vi "Decode PTU File Header.vi"(8 "error in (no error)":errorcluster, 11 "Tag Array":T1[](array[typedef]) {"TagType" format="%.0x"}) -> (0 "error out":errorcluster, 1 "Tags with Error":string[](array[string]), 3 "PicoQuant Data File Information":T2)   [LabVIEW 2021, in "PTU Files.lvlib"]
uses:
  PTU Files.lvlib
  PicoQuant Data File Information.ctl
  PicoQuant File Information.ctl
  PicoQuant Software Information.ctl
  PicoQuant Remote Request Information.ctl
  PicoQuant Hardware Information.ctl
  PicoQuant Input Channels.ctl
  PicoQuant Markers.ctl
  PicoQuant Modules.ctl
  PicoQuant Router Channels.ctl
  PicoQuant Measurement Information.ctl
  PicoQuant Image Information.ctl
  PicoQuant Results Format.ctl
  PicoQuant Measurement Results.ctl
  PicoQuant Header Tag.ctl
  PicoQuant File Header Tags.ctl
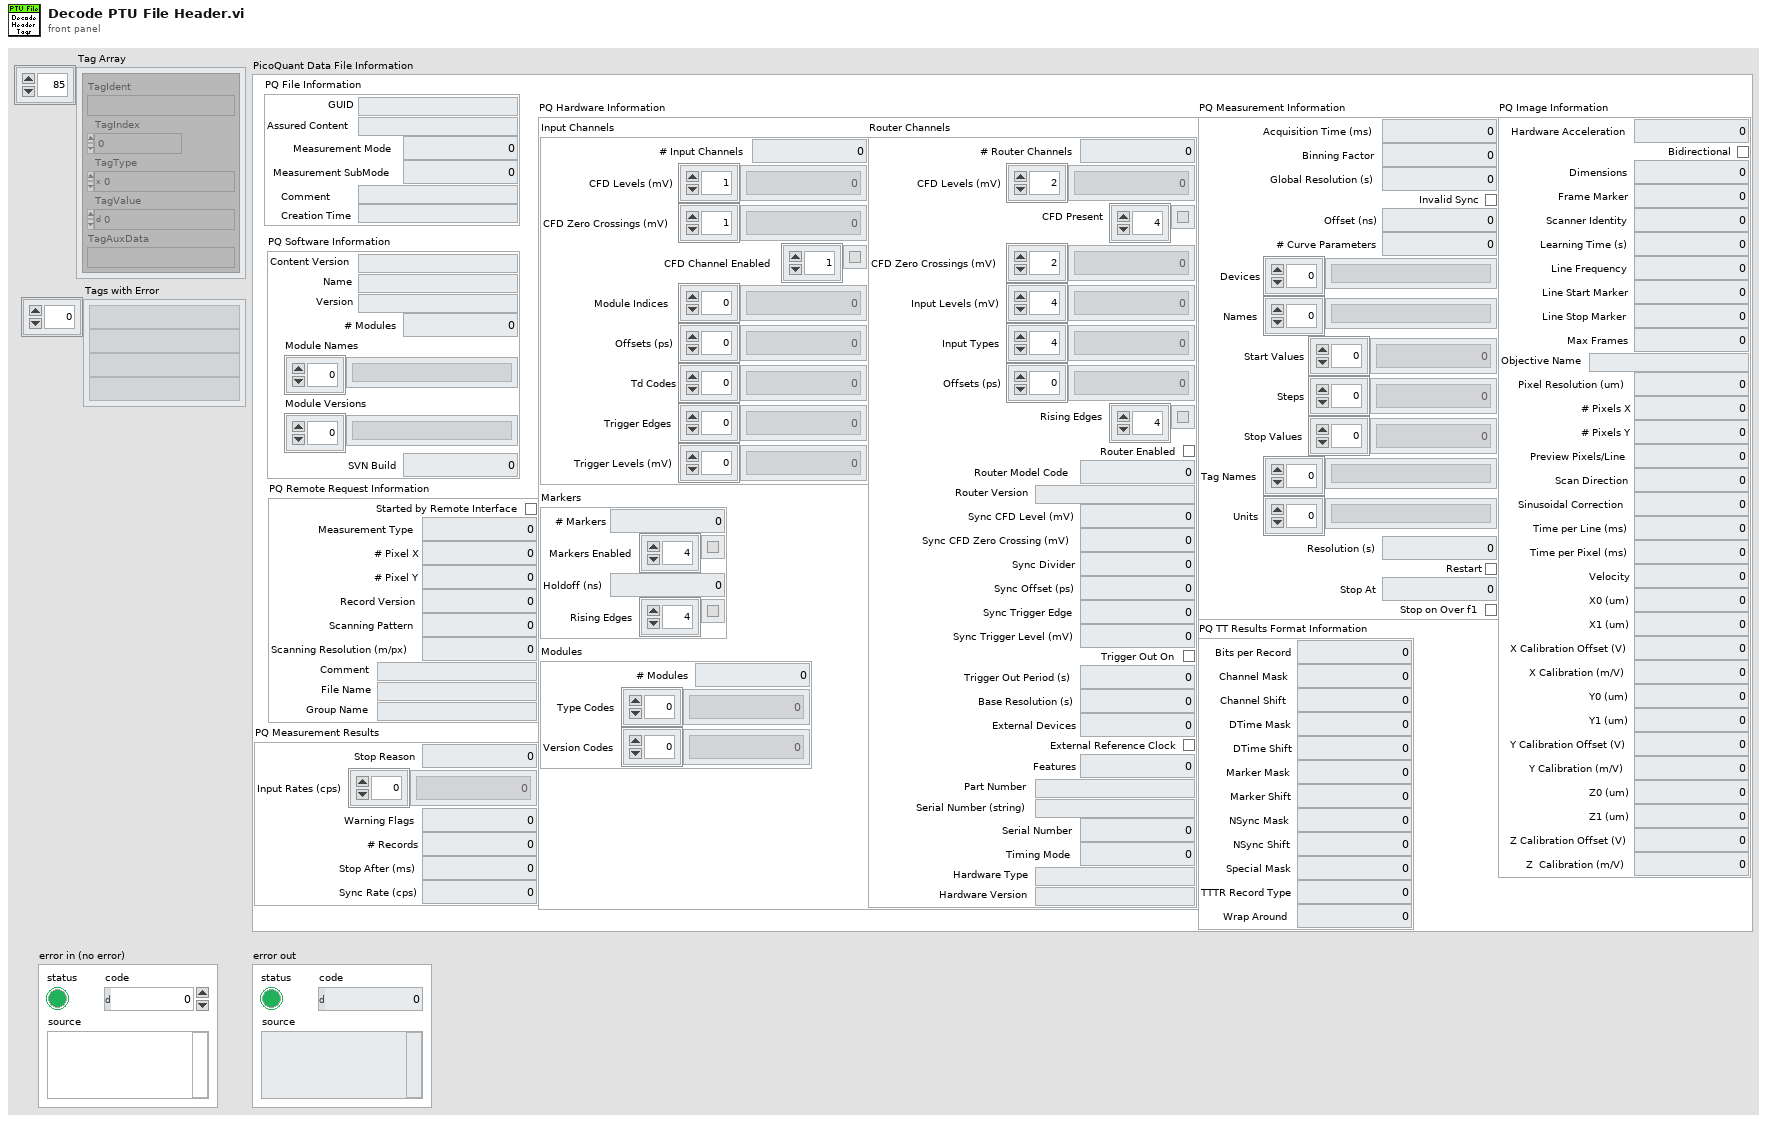
[diagram p1: front panel]
types:
  T1 = typedef "PTU Files.lvlib/PicoQuant Header Tag.ctl" = cluster{"TagIdent":string, "TagIndex":i32, "TagType":i32, "TagValue":i64, "TagAuxData":string}
  T2 = typedef "PTU Files.lvlib/PicoQuant Data File Information.ctl" = cluster{"PQ File Information":T3, "PQ Software Information":T4, "PQ Remote Request Information":T5, "PQ Hardware Information":T6, "PQ Measurement Information":T11, "PQ Image Information":T12, "PQ TT Results Format Information":T13, "PQ Measurement Results":T14}
  T3 = typedef "PTU Files.lvlib/PicoQuant File Information.ctl" = cluster{"GUID":string, "Assured Content":string, "Measurement Mode":i64, "Measurement SubMode":i64, "Comment":string, "Creation Time":string}
  T4 = typedef "PTU Files.lvlib/PicoQuant Software Information.ctl" = cluster{"Content Version":string, "Name":string, "Version":string, "# Modules":i64, "Module Names":string[], "Module Versions":string[], "SVN Build":i64}
  T5 = typedef "PTU Files.lvlib/PicoQuant Remote Request Information.ctl" = cluster{"Started by Remote Interface":bool, "Measurement Type":i64, "# Pixel X":i64, "# Pixel Y":i64, "Record Version":i64, "Scanning Pattern":i64, "Scanning Resolution (m/px)":dbl, "Comment":string, "File Name":string, "Group Name":string}
  T6 = typedef "PTU Files.lvlib/PicoQuant Hardware Information.ctl" = cluster{"Input Channels":T7, "Markers":T8, "Modules":T9, "Router Channels":T10}
  T7 = typedef "PTU Files.lvlib/PicoQuant Input Channels.ctl" = cluster{"# Input Channels":i64, "CFD Levels (mV)":i64[], "CFD Zero Crossings (mV)":i64[], "CFD Channel Enabled":bool[], "Module Indices":i64[], "Offsets (ps)":i64[], "Td Codes":i64[], "Trigger Edges":i64[], "Trigger Levels (mV)":i64[]}
  T8 = typedef "PTU Files.lvlib/PicoQuant Markers.ctl" = cluster{"# Markers":i64, "Markers Enabled":bool[], "Holdoff (ns)":i64, "Rising Edges":bool[]}
  T9 = typedef "PTU Files.lvlib/PicoQuant Modules.ctl" = cluster{"# Modules":i64, "Type Codes":i64[], "Version Codes":i64[]}
  T10 = typedef "PTU Files.lvlib/PicoQuant Router Channels.ctl" = cluster{"# Router Channels":i64, "CFD Levels (mV)":i64[], "CFD Present":bool[], "CFD Zero Crossings (mV)":i64[], "Input Levels (mV)":i64[], "Input Types":i64[], "Offsets (ps)":i64[], "Rising Edges":bool[], "Router Enabled":bool, "Router Model Code":i64, "Router Version":string, "Sync CFD Level (mV)":i64, "Sync CFD Zero Crossing (mV)":i64, "Sync Divider":i64, "Sync Offset (ps)":i64, "Sync Trigger Edge":i64, "Sync Trigger Level (mV)":i64, "Trigger Out On":bool, "Trigger Out Period (s)":dbl, "Base Resolution (s)":dbl, "External Devices":i64, "External Reference Clock":bool, "Features":u64, "Part Number":string, "Serial Number (string)":string, "Serial Number":i64, "Timing Mode":i64, "Hardware Type":string, "Hardware Version":string}
  T11 = typedef "PTU Files.lvlib/PicoQuant Measurement Information.ctl" = cluster{"Acquisition Time (ms)":i64, "Binning Factor":i64, "Global Resolution (s)":dbl, "Invalid Sync":bool, "Offset (ns)":u64, "# Curve Parameters":u64, "Devices":string[], "Names":string[], "Start Values":dbl[], "Steps":dbl[], "Stop Values":dbl[], "Tag Names":string[], "Units":string[], "Resolution (s)":dbl, "Restart":bool, "Stop At":u64, "Stop on Over f1":bool}
  T12 = typedef "PTU Files.lvlib/PicoQuant Image Information.ctl" = cluster{"Hardware Acceleration":i64, "Bidirectional":bool, "Dimensions":i64, "Frame Marker":i64, "Scanner Identity":i64, "Learning Time (s)":i64, "Line Frequency":dbl, "Line Start Marker":i64, "Line Stop Marker":i64, "Max Frames":i64, "Objective Name":string, "Pixel Resolution (um)":dbl, "# Pixels X":i64, "# Pixels Y":i64, "Preview Pixels/Line":i64, "Scan Direction":i64, "Sinusoidal Correction":i64, "Time per Line (ms)":dbl, "Time per Pixel (ms)":i64, "Velocity":i64, "X0 (um)":dbl, "X1 (um)":dbl, "X Calibration Offset (V)":dbl, "X Calibration (m/V)":dbl, "Y0 (um)":dbl, "Y1 (um)":dbl, "Y Calibration Offset (V)":dbl, "Y Calibration (m/V)":dbl, "Z0 (um)":dbl, "Z1 (um)":dbl, "Z Calibration Offset (V)":dbl, "Z  Calibration (m/V)":dbl}
  T13 = typedef "PTU Files.lvlib/PicoQuant Results Format.ctl" = cluster{"Bits per Record":i64, "Channel Mask":i64, "Channel Shift ":i64, "DTime Mask":i64, "DTime Shift":i64, "Marker Mask":i64, "Marker Shift":i64, "NSync Mask":i64, "NSync Shift":i64, "Special Mask":i64, "TTTR Record Type":i64, "Wrap Around":i64}
  T14 = typedef "PTU Files.lvlib/PicoQuant Measurement Results.ctl" = cluster{"Stop Reason":i64, "Input Rates (cps)":i64[], "Warning Flags":u64, "# Records":i64, "Stop After (ms)":i64, "Sync Rate (cps)":i64}
  T15 = typedef "PTU Files.lvlib/PicoQuant File Header Tags.ctl" = enum16{"<File Header>", "File_GUID", "File_AssuredContent", "File_Comment", "File_CreatingTime", "File_ParentResult_GUID", "File_RawData_GUID", "File_EditedBy", "Measurement_Mode", "Measurement_SubMode", "<Creator Software>", "CreatorSW_ContentVersion", "CreatorSW_Name", "CreatorSW_Version", "CreatorSW_Modules", "CreatorSW_ModuleName", "CreatorSW_ModuleVers", "CreatorSW_SVNBuild", "<Remote Request Data>", "$StartedByRemoteInterface", "<Remote Request Header mand.>", "$ReqHdr_MeasurementType", "$ReqHdr_PixelNumber_X", "$ReqHdr_PixelNumber_Y", "$ReqHdr_RecordVersion", "$ReqHdr_ScanningPattern", "$ReqHdr_SpatialResolution", "<Remote Request Header opt.>", "$Comment", "$Filename", "$Groupname", "<Remote Request Header undef.>", "$<Ident>", "<Hardware Header>", "HW_InpChannels", "HWInpChan_CFDLevel", "HWInpChan_CFDZeroCross", "HWInpChan_Enabled", "HWInpChan_ModuleIdx", "HWInpChan_Offset", "HWInpChan_TdCode", "HWInpChan_TrgEdge", "HWInpChan_TrgLevel", "HW_Markers", "HWMarkers_Enabled", "HWMarkers_HoldOff", "HWMarkers_RisingEdge", "HW_Modules", "HWModule_TypeCode", "HWModule_VersCode", "HWRouter_Channels", "HWRouterChan_CFDLevel", "HWRouterChan_CFDPresent", "HWRouterChan_CFDZeroCross", "HWRouterChan_InputLevel", "HWRouterChan_InputType", "HWRouterChan_Offset", "HWRouterChan_RisingEdge", "HWRouter_Enabled", "HWRouter_ModelCode", "HWRouter_Version", "HWSync_CFDLevel", "HWSync_CFDZeroCross", "HWSync_Divider", "HWSync_Offset", "HWSync_TrgEdge", "HWSync_TrgLevel", "HWTriggerOut_On", "HWTriggerOut_Period", "HW_BaseResolution", "HW_ExternalDevices", "HW_ExternalRefClock", "HW_Features", "HW_PartNo", "HW_RoutingChannels", "HW_SerialNo", "HW_Timingmode", "HW_Type", "HW_Version", "<Measurement Description>", "MeasDesc_AcquisitionTime", "MeasDesc_BinningFactor", "MeasDesc_GlobalResolution", "MeasDesc_InvalidSync", "MeasDesc_Offset", "MeasDesc_Params", "MeasDesc_Param_Device", "MeasDesc_Param_Name", "MeasDesc_Param_Start", "MeasDesc_Param_Step", "MeasDesc_Param_Stop", "MeasDesc_Param_TagName", "MeasDesc_Param_Unit", "MeasDesc_Resolution", "MeasDesc_Restart", "MeasDesc_StopAt", "MeasDesc_StopOnOvfl", "<Image Header>", "ImgHdr_Acceleration", "ImgHdr_BiDirect", "ImgHdr_Dimensions", "ImgHdr_Frame", "ImgHdr_Ident", "ImgHdr_LearningTime", "ImgHdr_LineFrequency", "ImgHdr_LineStart", "ImgHdr_LineStop", "ImgHdr_MaxFrames", "ImgHdr_ObjectiveName", "ImgHdr_PixResol", "ImgHdr_PixX", "ImgHdr_PixY", "ImgHdr_PrevPix", "ImgHdr_ScanDirection", "ImgHdr_SinCorrection", "ImgHdr_TimePerLine", "ImgHdr_TimePerPixel", "ImgHdr_TStartFro", "ImgHdr_TStartTo", "ImgHdr_TStopFro", "ImgHdr_TStopTo", "ImgHdr_Velocity", "ImgHdr_X0", "ImgHdr_X1", "ImgHdr_XCalibOffset", "ImgHdr_XCalibration", "ImgHdr_Y0", "ImgHdr_Y1", "ImgHdr_YCalibOffset", "ImgHdr_YCalibration", "ImgHdr_Z0", "ImgHdr_Z1", "ImgHdr_ZCalibOffset", "ImgHdr_ZCalibration", "<TT Measurement Results>", "TTResult_StopReason", "TTResult_InputRate", "TTResult_MDescWarningFlags", "TTResult_NumberOfRecords", "TTResult_StopAfter", "TTResult_SyncRate", "<TT Results Format>", "TTResultFormat_BitsPerRecord", "TTResultFormat_ChannelMask", "TTResultFormat_ChannelShift", "TTResultFormat_DTimeMask", "TTResultFormat_DTimeShift", "TTResultFormat_MarkerMask", "TTResultFormat_MarkerShift", "TTResultFormat_NSyncMask", "TTResultFormat_NSyncShift", "TTResultFormat_SpecialMask", "TTResultFormat_TTTRRecType", "TTResultFormat_WrapAround", "Header_End"}
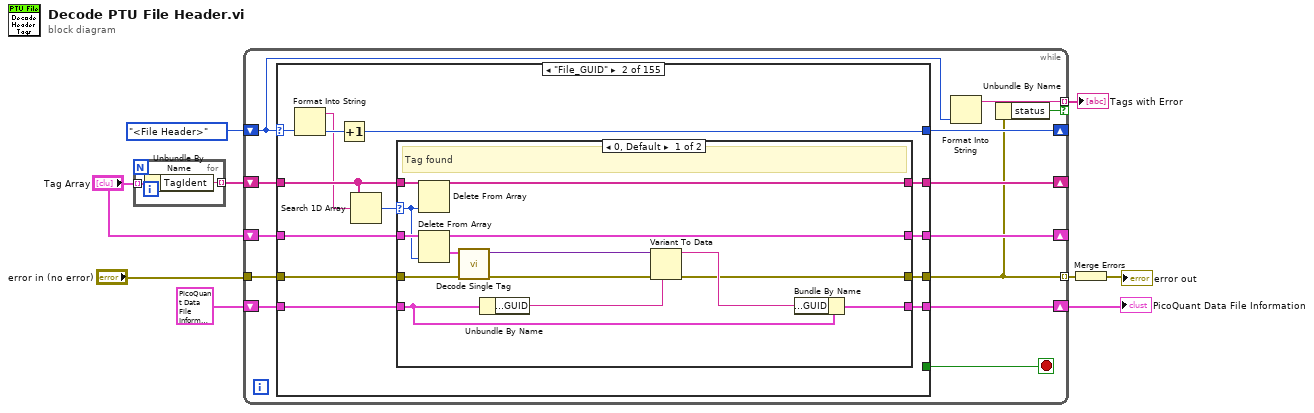
[diagram p0: block diagram]
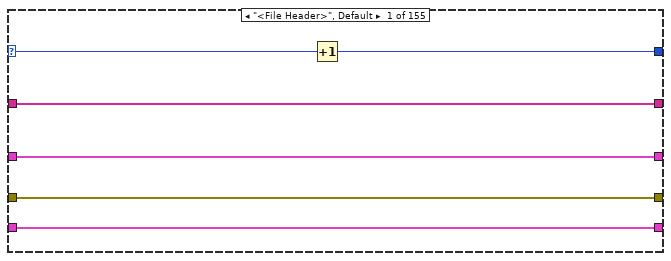
[diagram p2: hidden frame]
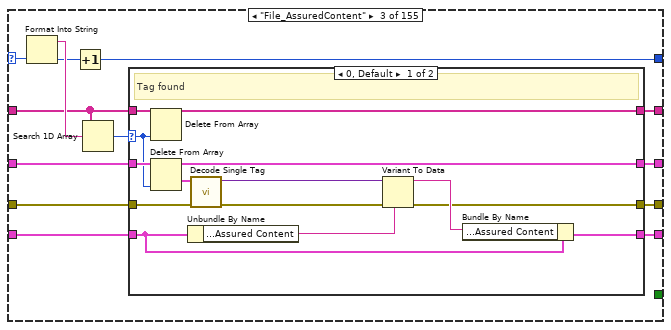
[diagram p4: hidden frame]
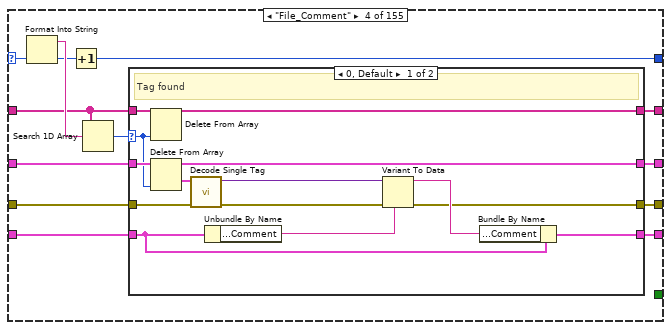
[diagram p6: hidden frame]
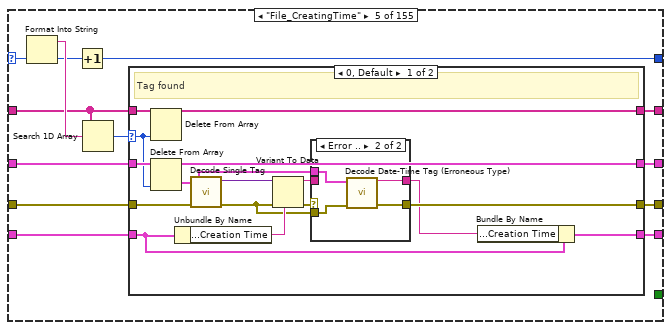
[diagram p8: hidden frame]
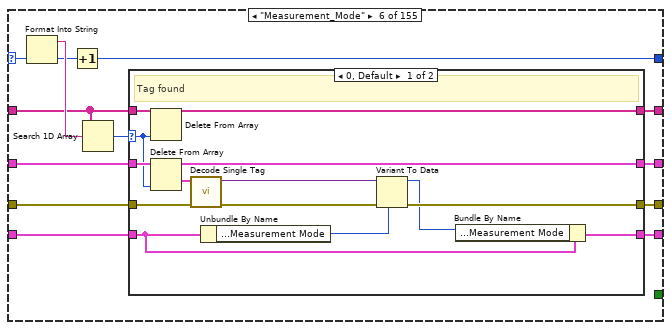
[diagram p11: hidden frame]
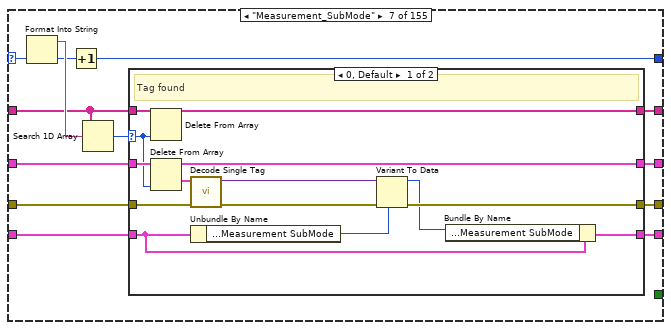
[diagram p13: hidden frame]
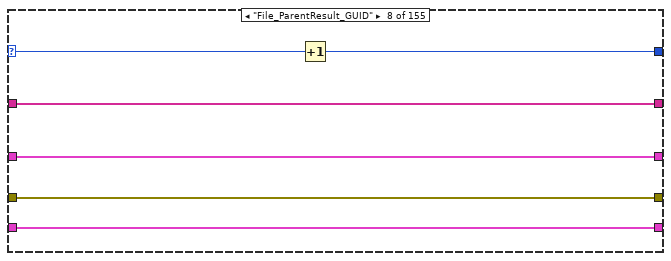
[diagram p15: hidden frame]
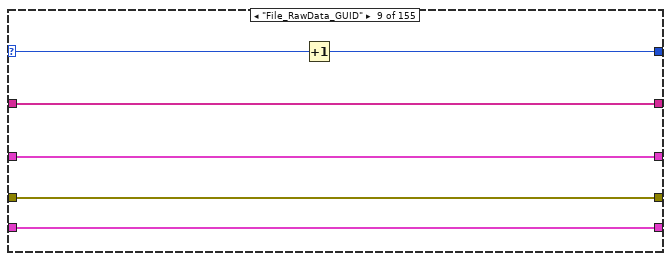
[diagram p16: hidden frame]
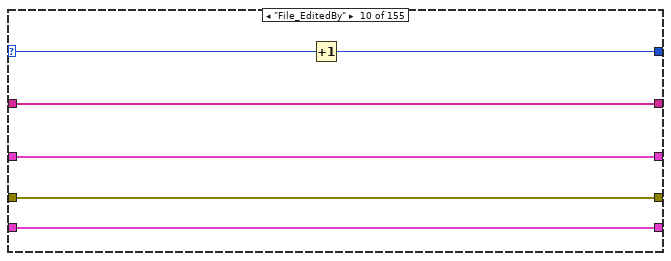
[diagram p17: hidden frame]
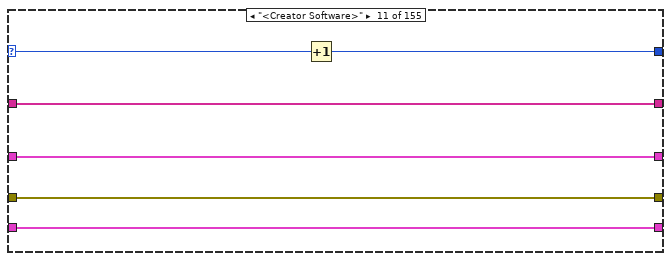
[diagram p18: hidden frame]
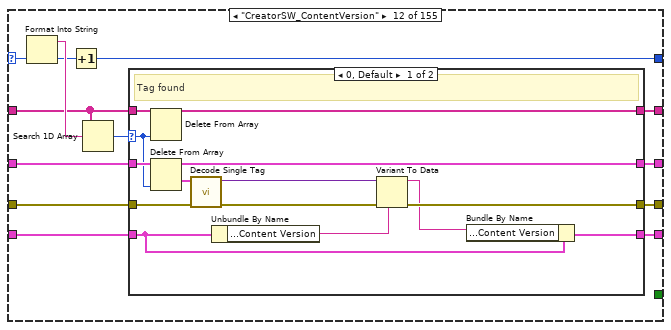
[diagram p19: hidden frame]
diagram:
  n1 = for {
    tunnel: "Tag Array" -> [w11] mode=indexing
    tunnel: [w10] -> w9 mode=indexing
    n2 = Unbundle By Name(w11) -> ("TagIdent"=w10:string)
  }
  n3 = while {
    shift-right: [w23] -> _
    shift-left: w9 -> [w24]
    shift-right: [w16] -> _
    shift-left: PicoQuant_File_Header_Tags."<File Header>" ("PQ File Header Tag") -> [w13]
    shift-right: [w21] -> w6
    shift-left: T2 {"PQ File Information"={"GUID"="", "Assured Content"="", "Measurement Mode"=0, "Measurement SubMode"=0, "Comment"="", "Creation Time"=""}, "PQ Software Information"={"Content Version"="", "Name"="", "Version"="", "# Modules"=0, "Module Names"=[], "Module Versions"=[], "SVN Build"=0}, "PQ Remote Request Information"={"Started by Remote Interface"=FALSE, "Measurement Type"=0, "# Pixel X"=0, "# Pixel Y"=0, "Record Version"=0, "Scanning Pattern"=0, "Scanning Resolution (m/px)"=0.0, "Comment"="", "File Name"="", "Group Name"=""}, "PQ Hardware Information"={"Input Channels"={"# Input Channels"=0, "CFD Levels (mV)"=[], "CFD Zero Crossings (mV)"=[], "CFD Channel Enabled"=[], "Module Indices"=[], "Offsets (ps)"=[], "Td Codes"=[], "Trigger Edges"=[], "Trigger Levels (mV)"=[]}, "Markers"={"# Markers"=0, "Markers Enabled"=[], "Holdoff (ns)"=0, "Rising Edges"=[]}, "Modules"={"# Modules"=0, "Type Codes"=[], "Version Codes"=[]}, "Router Channels"={"# Router Channels"=0, "CFD Levels (mV)"=[], "CFD Present"=[], "CFD Zero Crossings (mV)"=[], "Input Levels (mV)"=[], "Input Types"=[], "Offsets (ps)"=[], "Rising Edges"=[], "Router Enabled"=FALSE, "Router Model Code"=0, "Router Version"="", "Sync CFD Level (mV)"=0, "Sync CFD Zero Crossing (mV)"=0, "Sync Divider"=0, "Sync Offset (ps)"=0, "Sync Trigger Edge"=0, "Sync Trigger Level (mV)"=0, "Trigger Out On"=FALSE, "Trigger Out Period (s)"=0.0, "Base Resolution (s)"=0.0, "External Devices"=0, "External Reference Clock"=FALSE, "Features"=0, "Part Number"="", "Serial Number (string)"="", "Serial Number"=0, "Timing Mode"=0, "Hardware Type"="", "Hardware Version"=""}}, "PQ Measurement Information"={"Acquisition Time (ms)"=0, "Binning Factor"=0, "Global Resolution (s)"=0.0, "Invalid Sync"=FALSE, "Offset (ns)"=0, "# Curve Parameters"=0, "Devices"=[], "Names"=[], "Start Values"=[], "Steps"=[], "Stop Values"=[], "Tag Names"=[], "Units"=[], "Resolution (s)"=0.0, "Restart"=FALSE, "Stop At"=0, "Stop on Over f1"=FALSE}, "PQ Image Information"={"Hardware Acceleration"=0, "Bidirectional"=FALSE, "Dimensions"=0, "Frame Marker"=0, "Scanner Identity"=0, "Learning Time (s)"=0, "Line Frequency"=0.0, "Line Start Marker"=0, "Line Stop Marker"=0, "Max Frames"=0, "Objective Name"="", "Pixel Resolution (um)"=0.0, "# Pixels X"=0, "# Pixels Y"=0, "Preview Pixels/Line"=0, "Scan Direction"=0, "Sinusoidal Correction"=0, "Time per Line (ms)"=0.0, "Time per Pixel (ms)"=0, "Velocity"=0, "X0 (um)"=0.0, "X1 (um)"=0.0, "X Calibration Offset (V)"=0.0, "X Calibration (m/V)"=0.0, "Y0 (um)"=0.0, "Y1 (um)"=0.0, "Y Calibration Offset (V)"=0.0, "Y Calibration (m/V)"=0.0, "Z0 (um)"=0.0, "Z1 (um)"=0.0, "Z Calibration Offset (V)"=0.0, "Z  Calibration (m/V)"=0.0}, "PQ TT Results Format Information"={"Bits per Record"=0, "Channel Mask"=0, "Channel Shift "=0, "DTime Mask"=0, "DTime Shift"=0, "Marker Mask"=0, "Marker Shift"=0, "NSync Mask"=0, "NSync Shift"=0, "Special Mask"=0, "TTTR Record Type"=0, "Wrap Around"=0}, "PQ Measurement Results"={"Stop Reason"=0, "Input Rates (cps)"=[], "Warning Flags"=0, "# Records"=0, "Stop After (ms)"=0, "Sync Rate (cps)"=0}} ("PicoQuant Data File Information") -> [w22]
    shift-right: [w19] -> _
    shift-left: "Tag Array" -> [w20]
    tunnel: "error in (no error)" -> [w18]
    tunnel: [w15] -> w3 mode=indexing
    tunnel: [w12] -> w1 mode=indexing if=w14
    stop <- w17 stop-if-true
    n4 = case shown="\"File_GUID\"" w13 {
      selector: w13 -> [w26 w33 w62 w92 w122 w160 w190 w220 w226 w232 w238 w244 w274 w304 w334 w364 w399 w434 w464 w470 w500 w506 w536 w566 w596 w626 w656 w686 w692 w722 w752 w782 w788 w794 w800 w830 w865 w900 w935 w970 w1005 w1040 w1075 w1110 w1140 w1175 w1205 w1240 w1270 w1305 w1340 w1370 w1405 w1440 w1475 w1510 w1545 w1580 w1615 w1645 w1675 w1705 w1735 w1765 w1795 w1825 w1855 w1885 w1915 w1945 w1975 w2005 w2035 w2065 w2095 w2102 w2145 w2175 w2205 w2235 w2241 w2271 w2301 w2331 w2361 w2391 w2421 w2456 w2491 w2526 w2561 w2596 w2631 w2666 w2696 w2726 w2756 w2786 w2792 w2822 w2860 w2890 w2920 w2950 w2980 w3010 w3040 w3070 w3100 w3130 w3160 w3190 w3220 w3250 w3280 w3310 w3340 w3370 w3376 w3382 w3388 w3394 w3424 w3454 w3484 w3514 w3544 w3574 w3604 w3634 w3664 w3694 w3724 w3754 w3784 w3790 w3820 w3855 w3885 w3915 w3945 w3975 w3981 w4011 w4041 w4071 w4101 w4131 w4161 w4191 w4221 w4251 w4281 w4311 w4340]
      tunnel: w24 -> [w30 w39 w68 w98 w128 w166 w196 w223 w229 w235 w241 w250 w280 w310 w340 w370 w405 w440 w467 w476 w503 w512 w542 w572 w602 w632 w662 w689 w698 w728 w758 w785 w791 w797 w806 w836 w871 w906 w941 w976 w1011 w1046 w1081 w1116 w1146 w1181 w1211 w1246 w1276 w1311 w1346 w1376 w1411 w1446 w1481 w1516 w1551 w1586 w1621 w1651 w1681 w1711 w1741 w1771 w1801 w1831 w1861 w1891 w1921 w1951 w1981 w2011 w2041 w2071 w2098 w2108 w2151 w2181 w2211 w2238 w2247 w2277 w2307 w2337 w2367 w2397 w2427 w2462 w2497 w2532 w2567 w2602 w2637 w2672 w2702 w2732 w2762 w2789 w2798 w2828 w2866 w2896 w2926 w2956 w2986 w3016 w3046 w3076 w3106 w3136 w3166 w3196 w3226 w3256 w3286 w3316 w3346 w3371 w3379 w3385 w3391 w3400 w3430 w3460 w3490 w3520 w3550 w3580 w3610 w3640 w3670 w3700 w3730 w3760 w3787 w3796 w3826 w3861 w3891 w3921 w3951 w3976 w3987 w4017 w4047 w4077 w4107 w4137 w4167 w4197 w4227 w4257 w4287 w4317 w4344]
      tunnel: [w30 w38 w67 w97 w127 w165 w195 w223 w229 w235 w241 w249 w279 w309 w339 w369 w404 w439 w467 w475 w503 w511 w541 w571 w601 w631 w661 w689 w697 w727 w757 w785 w791 w797 w805 w835 w870 w905 w940 w975 w1010 w1045 w1080 w1115 w1145 w1180 w1210 w1245 w1275 w1310 w1345 w1375 w1410 w1445 w1480 w1515 w1550 w1585 w1620 w1650 w1680 w1710 w1740 w1770 w1800 w1830 w1860 w1890 w1920 w1950 w1980 w2010 w2040 w2070 w2098 w2107 w2150 w2180 w2210 w2238 w2246 w2276 w2306 w2336 w2366 w2396 w2426 w2461 w2496 w2531 w2566 w2601 w2636 w2671 w2701 w2731 w2761 w2789 w2797 w2827 w2865 w2895 w2925 w2955 w2985 w3015 w3045 w3075 w3105 w3135 w3165 w3195 w3225 w3255 w3285 w3315 w3345 w3371 w3379 w3385 w3391 w3399 w3429 w3459 w3489 w3519 w3549 w3579 w3609 w3639 w3669 w3699 w3729 w3759 w3787 w3795 w3825 w3860 w3890 w3920 w3950 w3976 w3986 w4016 w4046 w4076 w4106 w4136 w4166 w4196 w4226 w4256 w4286 w4316 w4344] -> w23
      tunnel: w22 -> [w28 w41 w70 w100 w130 w168 w198 w224 w230 w236 w242 w252 w282 w312 w342 w372 w407 w442 w468 w478 w504 w514 w544 w574 w604 w634 w664 w690 w700 w730 w760 w786 w792 w798 w808 w838 w873 w908 w943 w978 w1013 w1048 w1083 w1118 w1148 w1183 w1213 w1248 w1278 w1313 w1348 w1378 w1413 w1448 w1483 w1518 w1553 w1588 w1623 w1653 w1683 w1713 w1743 w1773 w1803 w1833 w1863 w1893 w1923 w1953 w1983 w2013 w2043 w2073 w2099 w2110 w2153 w2183 w2213 w2239 w2249 w2279 w2309 w2339 w2369 w2399 w2429 w2464 w2499 w2534 w2569 w2604 w2639 w2674 w2704 w2734 w2764 w2790 w2800 w2830 w2868 w2898 w2928 w2958 w2988 w3018 w3048 w3078 w3108 w3138 w3168 w3198 w3228 w3258 w3288 w3318 w3348 w3374 w3380 w3386 w3392 w3402 w3432 w3462 w3492 w3522 w3552 w3582 w3612 w3642 w3672 w3702 w3732 w3762 w3788 w3798 w3828 w3863 w3893 w3923 w3953 w3979 w3989 w4019 w4049 w4079 w4109 w4139 w4169 w4199 w4229 w4259 w4289 w4319 w4345]
      tunnel: [w28 w40 w69 w99 w129 w167 w197 w224 w230 w236 w242 w251 w281 w311 w341 w371 w406 w441 w468 w477 w504 w513 w543 w573 w603 w633 w663 w690 w699 w729 w759 w786 w792 w798 w807 w837 w872 w907 w942 w977 w1012 w1047 w1082 w1117 w1147 w1182 w1212 w1247 w1277 w1312 w1347 w1377 w1412 w1447 w1482 w1517 w1552 w1587 w1622 w1652 w1682 w1712 w1742 w1772 w1802 w1832 w1862 w1892 w1922 w1952 w1982 w2012 w2042 w2072 w2099 w2109 w2152 w2182 w2212 w2239 w2248 w2278 w2308 w2338 w2368 w2398 w2428 w2463 w2498 w2533 w2568 w2603 w2638 w2673 w2703 w2733 w2763 w2790 w2799 w2829 w2867 w2897 w2927 w2957 w2987 w3017 w3047 w3077 w3107 w3137 w3167 w3197 w3227 w3257 w3287 w3317 w3347 w3374 w3380 w3386 w3392 w3401 w3431 w3461 w3491 w3521 w3551 w3581 w3611 w3641 w3671 w3701 w3731 w3761 w3788 w3797 w3827 w3862 w3892 w3922 w3952 w3979 w3988 w4018 w4048 w4078 w4108 w4138 w4168 w4198 w4228 w4258 w4288 w4318 w4345] -> w21
      tunnel: w20 -> [w29 w37 w66 w96 w126 w164 w194 w222 w228 w234 w240 w248 w278 w308 w338 w368 w403 w438 w466 w474 w502 w510 w540 w570 w600 w630 w660 w688 w696 w726 w756 w784 w790 w796 w804 w834 w869 w904 w939 w974 w1009 w1044 w1079 w1114 w1144 w1179 w1209 w1244 w1274 w1309 w1344 w1374 w1409 w1444 w1479 w1514 w1549 w1584 w1619 w1649 w1679 w1709 w1739 w1769 w1799 w1829 w1859 w1889 w1919 w1949 w1979 w2009 w2039 w2069 w2097 w2106 w2149 w2179 w2209 w2237 w2245 w2275 w2305 w2335 w2365 w2395 w2425 w2460 w2495 w2530 w2565 w2600 w2635 w2670 w2700 w2730 w2760 w2788 w2796 w2826 w2864 w2894 w2924 w2954 w2984 w3014 w3044 w3074 w3104 w3134 w3164 w3194 w3224 w3254 w3284 w3314 w3344 w3373 w3378 w3384 w3390 w3398 w3428 w3458 w3488 w3518 w3548 w3578 w3608 w3638 w3668 w3698 w3728 w3758 w3786 w3794 w3824 w3859 w3889 w3919 w3949 w3978 w3985 w4015 w4045 w4075 w4105 w4135 w4165 w4195 w4225 w4255 w4285 w4315 w4343]
      tunnel: [w29 w36 w65 w95 w125 w163 w193 w222 w228 w234 w240 w247 w277 w307 w337 w367 w402 w437 w466 w473 w502 w509 w539 w569 w599 w629 w659 w688 w695 w725 w755 w784 w790 w796 w803 w833 w868 w903 w938 w973 w1008 w1043 w1078 w1113 w1143 w1178 w1208 w1243 w1273 w1308 w1343 w1373 w1408 w1443 w1478 w1513 w1548 w1583 w1618 w1648 w1678 w1708 w1738 w1768 w1798 w1828 w1858 w1888 w1918 w1948 w1978 w2008 w2038 w2068 w2097 w2105 w2148 w2178 w2208 w2237 w2244 w2274 w2304 w2334 w2364 w2394 w2424 w2459 w2494 w2529 w2564 w2599 w2634 w2669 w2699 w2729 w2759 w2788 w2795 w2825 w2863 w2893 w2923 w2953 w2983 w3013 w3043 w3073 w3103 w3133 w3163 w3193 w3223 w3253 w3283 w3313 w3343 w3373 w3378 w3384 w3390 w3397 w3427 w3457 w3487 w3517 w3547 w3577 w3607 w3637 w3667 w3697 w3727 w3757 w3786 w3793 w3823 w3858 w3888 w3918 w3948 w3978 w3984 w4014 w4044 w4074 w4104 w4134 w4164 w4194 w4224 w4254 w4284 w4314 w4343] -> w19
      tunnel: [w27 w35 w64 w94 w124 w162 w192 w221 w227 w233 w239 w246 w276 w306 w336 w366 w401 w436 w465 w472 w501 w508 w538 w568 w598 w628 w658 w687 w694 w724 w754 w783 w789 w795 w802 w832 w867 w902 w937 w972 w1007 w1042 w1077 w1112 w1142 w1177 w1207 w1242 w1272 w1307 w1342 w1372 w1407 w1442 w1477 w1512 w1547 w1582 w1617 w1647 w1677 w1707 w1737 w1767 w1797 w1827 w1857 w1887 w1917 w1947 w1977 w2007 w2037 w2067 w2096 w2104 w2147 w2177 w2207 w2236 w2243 w2273 w2303 w2333 w2363 w2393 w2423 w2458 w2493 w2528 w2563 w2598 w2633 w2668 w2698 w2728 w2758 w2787 w2794 w2824 w2862 w2892 w2922 w2952 w2982 w3012 w3042 w3072 w3102 w3132 w3162 w3192 w3222 w3252 w3282 w3312 w3342 w3372 w3377 w3383 w3389 w3396 w3426 w3456 w3486 w3516 w3546 w3576 w3606 w3636 w3666 w3696 w3726 w3756 w3785 w3792 w3822 w3857 w3887 w3917 w3947 w3977 w3983 w4013 w4043 w4073 w4103 w4133 w4163 w4193 w4223 w4253 w4283 w4313 w4342] -> w15
      tunnel: w18 -> [w27 w34 w63 w93 w123 w161 w191 w221 w227 w233 w239 w245 w275 w305 w335 w365 w400 w435 w465 w471 w501 w507 w537 w567 w597 w627 w657 w687 w693 w723 w753 w783 w789 w795 w801 w831 w866 w901 w936 w971 w1006 w1041 w1076 w1111 w1141 w1176 w1206 w1241 w1271 w1306 w1341 w1371 w1406 w1441 w1476 w1511 w1546 w1581 w1616 w1646 w1676 w1706 w1736 w1766 w1796 w1826 w1856 w1886 w1916 w1946 w1976 w2006 w2036 w2066 w2096 w2103 w2146 w2176 w2206 w2236 w2242 w2272 w2302 w2332 w2362 w2392 w2422 w2457 w2492 w2527 w2562 w2597 w2632 w2667 w2697 w2727 w2757 w2787 w2793 w2823 w2861 w2891 w2921 w2951 w2981 w3011 w3041 w3071 w3101 w3131 w3161 w3191 w3221 w3251 w3281 w3311 w3341 w3372 w3377 w3383 w3389 w3395 w3425 w3455 w3485 w3515 w3545 w3575 w3605 w3635 w3665 w3695 w3725 w3755 w3785 w3791 w3821 w3856 w3886 w3916 w3946 w3977 w3982 w4012 w4042 w4072 w4102 w4132 w4162 w4192 w4222 w4252 w4282 w4312 w4342]
      tunnel: [_ _ _ _ _ _ _ _ _ _ _ _ _ _ _ _ _ _ _ _ _ _ _ _ _ _ _ _ _ _ _ _ _ _ _ _ _ _ _ _ _ _ _ _ _ _ _ _ _ _ _ _ _ _ _ _ _ _ _ _ _ _ _ _ _ _ _ _ _ _ _ _ _ _ _ _ _ _ _ _ _ _ _ _ _ _ _ _ _ _ _ _ _ _ _ _ _ _ _ _ _ _ _ _ _ _ _ _ _ _ _ _ _ _ _ _ _ _ _ _ _ _ _ _ _ _ _ _ _ _ _ _ _ _ _ _ _ _ _ _ _ _ _ _ _ _ _ _ _ _ _ _ _ _ TRUE] -> w17
      tunnel: [w25 w32 w61 w91 w121 w159 w189 w219 w225 w231 w237 w243 w273 w303 w333 w363 w398 w433 w463 w469 w499 w505 w535 w565 w595 w625 w655 w685 w691 w721 w751 w781 w787 w793 w799 w829 w864 w899 w934 w969 w1004 w1039 w1074 w1109 w1139 w1174 w1204 w1239 w1269 w1304 w1339 w1369 w1404 w1439 w1474 w1509 w1544 w1579 w1614 w1644 w1674 w1704 w1734 w1764 w1794 w1824 w1854 w1884 w1914 w1944 w1974 w2004 w2034 w2064 w2094 w2101 w2144 w2174 w2204 w2234 w2240 w2270 w2300 w2330 w2360 w2390 w2420 w2455 w2490 w2525 w2560 w2595 w2630 w2665 w2695 w2725 w2755 w2785 w2791 w2821 w2859 w2889 w2919 w2949 w2979 w3009 w3039 w3069 w3099 w3129 w3159 w3189 w3219 w3249 w3279 w3309 w3339 w3369 w3375 w3381 w3387 w3393 w3423 w3453 w3483 w3513 w3543 w3573 w3603 w3633 w3663 w3693 w3723 w3753 w3783 w3789 w3819 w3854 w3884 w3914 w3944 w3974 w3980 w4010 w4040 w4070 w4100 w4130 w4160 w4190 w4220 w4250 w4280 w4310 w4340] -> w16
      frame "<File Header>", Default {
        n5 = Increment(x=w26) -> (x+1=w25:T15)
      }
      frame "File_GUID" {
        n6 = Format Into String(w33) -> (resulting string=w31:string)  [unwired: 3 in, 1 out]
        n7 = Increment(x=w33) -> (x+1=w32:T15)
        n8 = Search 1D Array(1D array=w39, element=w31) -> (index of element=w42:i32)  [unwired: 1 in]
        n9 = case shown="0, Default" w42 {
          selector: w42 -> [w52 _]
          tunnel: w41 -> [w46 w60]
          tunnel: [w51 w60] -> w40
          tunnel: w39 -> [w56 w59]
          tunnel: [w55 w59] -> w38
          tunnel: w37 -> [w54 w58]
          tunnel: [w53 w58] -> w36
          tunnel: [w44 w57] -> w35
          tunnel: w34 -> [w43 w57]
          frame 0, Default {
            # "Tag found"
            n10 = Delete From Array(array=w56, index=w52) -> (array with subset deleted=w55:string[])  [unwired: 1 in, 1 out]
            n11 = Delete From Array(array=w54, index=w52) -> (deleted portion=w50:T1, array with subset deleted=w53:T1[])  [unwired: 1 in]
            n12 = call "Decode Single Tag.vi"("Error In"=w43, "PicoQuant Tag"=w50) -> ("Error Out"=w48:errorcluster, "Variant"=w49:variant)  [unwired: 8 in]
            n13 = Unbundle By Name(w46) -> ("PQ File Information.GUID"=w45:string)
            n14 = Variant To Data(error in=w48, type=w45, Variant=w49) -> (data=w47:string, error out=w44:errorcluster)
            n15 = Bundle By Name(cluster=w46, "PQ File Information.GUID"=w47) -> (w51:T2)
          }
          frame -1 {
            # "Tag not found"
          }
        }
      }
      frame "File_AssuredContent" {
        n16 = Format Into String(w62) -> (resulting string=w72:string)  [unwired: 3 in, 1 out]
        n17 = Increment(x=w62) -> (x+1=w61:T15)
        n18 = Search 1D Array(1D array=w68, element=w72) -> (index of element=w71:i32)  [unwired: 1 in]
        n19 = case shown="0, Default" w71 {
          selector: w71 -> [w82 _]
          tunnel: w70 -> [w76 w90]
          tunnel: [w81 w90] -> w69
          tunnel: w68 -> [w86 w89]
          tunnel: [w85 w89] -> w67
          tunnel: w66 -> [w84 w88]
          tunnel: [w83 w88] -> w65
          tunnel: [w74 w87] -> w64
          tunnel: w63 -> [w73 w87]
          frame 0, Default {
            # "Tag found"
            n20 = Delete From Array(array=w86, index=w82) -> (array with subset deleted=w85:string[])  [unwired: 1 in, 1 out]
            n21 = Delete From Array(array=w84, index=w82) -> (deleted portion=w80:T1, array with subset deleted=w83:T1[])  [unwired: 1 in]
            n22 = Unbundle By Name(w76) -> ("PQ File Information.Assured Content"=w75:string)
            n23 = call "Decode Single Tag.vi"("Error In"=w73, "PicoQuant Tag"=w80) -> ("Error Out"=w78:errorcluster, "Variant"=w79:variant)  [unwired: 8 in]
            n24 = Variant To Data(error in=w78, type=w75, Variant=w79) -> (data=w77:string, error out=w74:errorcluster)
            n25 = Bundle By Name(cluster=w76, "PQ File Information.Assured Content"=w77) -> (w81:T2)
          }
          frame -1 {
            # "Tag not found"
          }
        }
      }
      frame "File_Comment" {
        n26 = Format Into String(w92) -> (resulting string=w102:string)  [unwired: 3 in, 1 out]
        n27 = Increment(x=w92) -> (x+1=w91:T15)
        n28 = Search 1D Array(1D array=w98, element=w102) -> (index of element=w101:i32)  [unwired: 1 in]
        n29 = case shown="0, Default" w101 {
          selector: w101 -> [w112 _]
          tunnel: w100 -> [w106 w120]
          tunnel: [w111 w120] -> w99
          tunnel: w98 -> [w116 w119]
          tunnel: [w115 w119] -> w97
          tunnel: w96 -> [w114 w118]
          tunnel: [w113 w118] -> w95
          tunnel: [w104 w117] -> w94
          tunnel: w93 -> [w103 w117]
          frame 0, Default {
            # "Tag found"
            n30 = Delete From Array(array=w116, index=w112) -> (array with subset deleted=w115:string[])  [unwired: 1 in, 1 out]
            n31 = Delete From Array(array=w114, index=w112) -> (deleted portion=w110:T1, array with subset deleted=w113:T1[])  [unwired: 1 in]
            n32 = call "Decode Single Tag.vi"("Error In"=w103, "PicoQuant Tag"=w110) -> ("Error Out"=w108:errorcluster, "Variant"=w109:variant)  [unwired: 8 in]
            n33 = Unbundle By Name(w106) -> ("PQ File Information.Comment"=w105:string)
            n34 = Variant To Data(error in=w108, type=w105, Variant=w109) -> (data=w107:string, error out=w104:errorcluster)
            n35 = Bundle By Name(cluster=w106, "PQ File Information.Comment"=w107) -> (w111:T2)
          }
          frame -1 {
            # "Tag not found"
          }
        }
      }
      frame "File_CreatingTime" {
        n36 = Format Into String(w122) -> (resulting string=w132:string)  [unwired: 3 in, 1 out]
        n37 = Increment(x=w122) -> (x+1=w121:T15)
        n38 = Search 1D Array(1D array=w128, element=w132) -> (index of element=w131:i32)  [unwired: 1 in]
        n39 = case shown="0, Default" w131 {
          selector: w131 -> [w144 _]
          tunnel: w130 -> [w142 w158]
          tunnel: [w143 w158] -> w129
          tunnel: w128 -> [w148 w157]
          tunnel: [w147 w157] -> w127
          tunnel: w126 -> [w146 w156]
          tunnel: [w145 w156] -> w125
          tunnel: [w136 w155] -> w124
          tunnel: w123 -> [w140 w155]
          frame 0, Default {
            # "Tag found"
            n40 = Delete From Array(array=w148, index=w144) -> (array with subset deleted=w147:string[])  [unwired: 1 in, 1 out]
            n41 = Delete From Array(array=w146, index=w144) -> (deleted portion=w133:T1, array with subset deleted=w145:T1[])  [unwired: 1 in]
            n42 = Unbundle By Name(w142) -> ("PQ File Information.Creation Time"=w141:string)
            n43 = call "Decode Single Tag.vi"("Error In"=w140, "PicoQuant Tag"=w133) -> ("Error Out"=w137:errorcluster, "Variant"=w138:variant)  [unwired: 8 in]
            n44 = Variant To Data(error in=w137, type=w141, Variant=w138) -> (data=w135:string, error out=w139:errorcluster)
            n45 = case shown="Error .." w139 {
              tunnel: w133 -> [_ w154]
              tunnel: w137 -> [w149 w153]
              tunnel: [w149 w152] -> w136
              tunnel: w135 -> [w150 _]
              tunnel: [w150 w151] -> w134
              frame No Error {
              }
              frame Error {
                n46 = call "Decode Date-Time Tag (Erroneous Type).vi"("error in (no error)"=w153, "PicoQuant Tag"=w154) -> ("error out"=w152:errorcluster, "Creation Time"=w151:string)  [unwired: 8 in]
              }
            }
            n47 = Bundle By Name(cluster=w142, "PQ File Information.Creation Time"=w134) -> (w143:T2)
          }
          frame -1 {
            # "Tag not found"
          }
        }
      }
      frame "Measurement_Mode" {
        n48 = Format Into String(w160) -> (resulting string=w170:string)  [unwired: 3 in, 1 out]
        n49 = Increment(x=w160) -> (x+1=w159:T15)
        n50 = Search 1D Array(1D array=w166, element=w170) -> (index of element=w169:i32)  [unwired: 1 in]
        n51 = case shown="0, Default" w169 {
          selector: w169 -> [w180 _]
          tunnel: w168 -> [w176 w188]
          tunnel: [w179 w188] -> w167
          tunnel: w166 -> [w184 w187]
          tunnel: [w183 w187] -> w165
          tunnel: w164 -> [w182 w186]
          tunnel: [w181 w186] -> w163
          tunnel: [w173 w185] -> w162
          tunnel: w161 -> [w174 w185]
          frame 0, Default {
            # "Tag found"
            n52 = Delete From Array(array=w184, index=w180) -> (array with subset deleted=w183:string[])  [unwired: 1 in, 1 out]
            n53 = Delete From Array(array=w182, index=w180) -> (deleted portion=w178:T1, array with subset deleted=w181:T1[])  [unwired: 1 in]
            n54 = call "Decode Single Tag.vi"("Error In"=w174, "PicoQuant Tag"=w178) -> ("Error Out"=w177:errorcluster, "Variant"=w171:variant)  [unwired: 8 in]
            n55 = Unbundle By Name(w176) -> ("PQ File Information.Measurement Mode"=w175:i64)
            n56 = Variant To Data(error in=w177, type=w175, Variant=w171) -> (data=w172:i64, error out=w173:errorcluster)
            n57 = Bundle By Name(cluster=w176, "PQ File Information.Measurement Mode"=w172) -> (w179:T2)
          }
          frame -1 {
            # "Tag not found"
          }
        }
      }
      frame "Measurement_SubMode" {
        n58 = Format Into String(w190) -> (resulting string=w200:string)  [unwired: 3 in, 1 out]
        n59 = Increment(x=w190) -> (x+1=w189:T15)
        n60 = Search 1D Array(1D array=w196, element=w200) -> (index of element=w199:i32)  [unwired: 1 in]
        n61 = case shown="0, Default" w199 {
          selector: w199 -> [w210 _]
          tunnel: w198 -> [w206 w218]
          tunnel: [w209 w218] -> w197
          tunnel: w196 -> [w214 w217]
          tunnel: [w213 w217] -> w195
          tunnel: w194 -> [w212 w216]
          tunnel: [w211 w216] -> w193
          tunnel: [w203 w215] -> w192
          tunnel: w191 -> [w204 w215]
          frame 0, Default {
            # "Tag found"
            n62 = Delete From Array(array=w214, index=w210) -> (array with subset deleted=w213:string[])  [unwired: 1 in, 1 out]
            n63 = Delete From Array(array=w212, index=w210) -> (deleted portion=w208:T1, array with subset deleted=w211:T1[])  [unwired: 1 in]
            n64 = call "Decode Single Tag.vi"("Error In"=w204, "PicoQuant Tag"=w208) -> ("Error Out"=w207:errorcluster, "Variant"=w201:variant)  [unwired: 8 in]
            n65 = Unbundle By Name(w206) -> ("PQ File Information.Measurement SubMode"=w205:i64)
            n66 = Variant To Data(error in=w207, type=w205, Variant=w201) -> (data=w202:i64, error out=w203:errorcluster)
            n67 = Bundle By Name(cluster=w206, "PQ File Information.Measurement SubMode"=w202) -> (w209:T2)
          }
          frame -1 {
            # "Tag not found"
          }
        }
      }
      frame "File_ParentResult_GUID" {
        n68 = Increment(x=w220) -> (x+1=w219:T15)
      }
      frame "File_RawData_GUID" {
        n69 = Increment(x=w226) -> (x+1=w225:T15)
      }
      frame "File_EditedBy" {
        n70 = Increment(x=w232) -> (x+1=w231:T15)
      }
      frame "<Creator Software>" {
        n71 = Increment(x=w238) -> (x+1=w237:T15)
      }
      frame "CreatorSW_ContentVersion" {
        n72 = Format Into String(w244) -> (resulting string=w254:string)  [unwired: 3 in, 1 out]
        n73 = Increment(x=w244) -> (x+1=w243:T15)
        n74 = Search 1D Array(1D array=w250, element=w254) -> (index of element=w253:i32)  [unwired: 1 in]
        n75 = case shown="0, Default" w253 {
          selector: w253 -> [w264 _]
          tunnel: w252 -> [w260 w272]
          tunnel: [w263 w272] -> w251
          tunnel: w250 -> [w268 w271]
          tunnel: [w267 w271] -> w249
          tunnel: w248 -> [w266 w270]
          tunnel: [w265 w270] -> w247
          tunnel: [w257 w269] -> w246
          tunnel: w245 -> [w258 w269]
          frame 0, Default {
            # "Tag found"
            n76 = Delete From Array(array=w268, index=w264) -> (array with subset deleted=w267:string[])  [unwired: 1 in, 1 out]
            n77 = Delete From Array(array=w266, index=w264) -> (deleted portion=w262:T1, array with subset deleted=w265:T1[])  [unwired: 1 in]
            n78 = call "Decode Single Tag.vi"("Error In"=w258, "PicoQuant Tag"=w262) -> ("Error Out"=w261:errorcluster, "Variant"=w255:variant)  [unwired: 8 in]
            n79 = Unbundle By Name(w260) -> ("PQ Software Information.Content Version"=w259:string)
            n80 = Variant To Data(error in=w261, type=w259, Variant=w255) -> (data=w256:string, error out=w257:errorcluster)
            n81 = Bundle By Name(cluster=w260, "PQ Software Information.Content Version"=w256) -> (w263:T2)
          }
          frame -1 {
            # "Tag not found"
          }
        }
      }
      frame "CreatorSW_Name" {
        n82 = Format Into String(w274) -> (resulting string=w284:string)  [unwired: 3 in, 1 out]
        n83 = Increment(x=w274) -> (x+1=w273:T15)
        n84 = Search 1D Array(1D array=w280, element=w284) -> (index of element=w283:i32)  [unwired: 1 in]
        n85 = case shown="0, Default" w283 {
          selector: w283 -> [w294 _]
          tunnel: w282 -> [w290 w302]
          tunnel: [w293 w302] -> w281
          tunnel: w280 -> [w298 w301]
          tunnel: [w297 w301] -> w279
          tunnel: w278 -> [w296 w300]
          tunnel: [w295 w300] -> w277
          tunnel: [w287 w299] -> w276
          tunnel: w275 -> [w288 w299]
          frame 0, Default {
            # "Tag found"
            n86 = Delete From Array(array=w298, index=w294) -> (array with subset deleted=w297:string[])  [unwired: 1 in, 1 out]
            n87 = Delete From Array(array=w296, index=w294) -> (deleted portion=w292:T1, array with subset deleted=w295:T1[])  [unwired: 1 in]
            n88 = call "Decode Single Tag.vi"("Error In"=w288, "PicoQuant Tag"=w292) -> ("Error Out"=w291:errorcluster, "Variant"=w285:variant)  [unwired: 8 in]
            n89 = Unbundle By Name(w290) -> ("PQ Software Information.Name"=w289:string)
            n90 = Variant To Data(error in=w291, type=w289, Variant=w285) -> (data=w286:string, error out=w287:errorcluster)
            n91 = Bundle By Name(cluster=w290, "PQ Software Information.Name"=w286) -> (w293:T2)
          }
          frame -1 {
            # "Tag not found"
          }
        }
      }
      frame "CreatorSW_Version" {
        n92 = Format Into String(w304) -> (resulting string=w314:string)  [unwired: 3 in, 1 out]
        n93 = Increment(x=w304) -> (x+1=w303:T15)
        n94 = Search 1D Array(1D array=w310, element=w314) -> (index of element=w313:i32)  [unwired: 1 in]
        n95 = case shown="0, Default" w313 {
          selector: w313 -> [w324 _]
          tunnel: w312 -> [w320 w332]
          tunnel: [w323 w332] -> w311
          tunnel: w310 -> [w328 w331]
          tunnel: [w327 w331] -> w309
          tunnel: w308 -> [w326 w330]
          tunnel: [w325 w330] -> w307
          tunnel: [w317 w329] -> w306
          tunnel: w305 -> [w318 w329]
          frame 0, Default {
            # "Tag found"
            n96 = Delete From Array(array=w328, index=w324) -> (array with subset deleted=w327:string[])  [unwired: 1 in, 1 out]
            n97 = Delete From Array(array=w326, index=w324) -> (deleted portion=w322:T1, array with subset deleted=w325:T1[])  [unwired: 1 in]
            n98 = call "Decode Single Tag.vi"("Error In"=w318, "PicoQuant Tag"=w322) -> ("Error Out"=w321:errorcluster, "Variant"=w315:variant)  [unwired: 8 in]
            n99 = Unbundle By Name(w320) -> ("PQ Software Information.Version"=w319:string)
            n100 = Variant To Data(error in=w321, type=w319, Variant=w315) -> (data=w316:string, error out=w317:errorcluster)
            n101 = Bundle By Name(cluster=w320, "PQ Software Information.Version"=w316) -> (w323:T2)
          }
          frame -1 {
            # "Tag not found"
          }
        }
      }
      frame "CreatorSW_Modules" {
        n102 = Format Into String(w334) -> (resulting string=w344:string)  [unwired: 3 in, 1 out]
        n103 = Increment(x=w334) -> (x+1=w333:T15)
        n104 = Search 1D Array(1D array=w340, element=w344) -> (index of element=w343:i32)  [unwired: 1 in]
        n105 = case shown="0, Default" w343 {
          selector: w343 -> [w354 _]
          tunnel: w342 -> [w350 w362]
          tunnel: [w353 w362] -> w341
          tunnel: w340 -> [w358 w361]
          tunnel: [w357 w361] -> w339
          tunnel: w338 -> [w356 w360]
          tunnel: [w355 w360] -> w337
          tunnel: [w347 w359] -> w336
          tunnel: w335 -> [w348 w359]
          frame 0, Default {
            # "Tag found"
            n106 = Delete From Array(array=w358, index=w354) -> (array with subset deleted=w357:string[])  [unwired: 1 in, 1 out]
            n107 = Delete From Array(array=w356, index=w354) -> (deleted portion=w352:T1, array with subset deleted=w355:T1[])  [unwired: 1 in]
            n108 = call "Decode Single Tag.vi"("Error In"=w348, "PicoQuant Tag"=w352) -> ("Error Out"=w351:errorcluster, "Variant"=w346:variant)  [unwired: 8 in]
            n109 = Unbundle By Name(w350) -> ("PQ Software Information.# Modules"=w349:i64)
            n110 = Variant To Data(error in=w351, type=w349, Variant=w346) -> (data=w345:i64, error out=w347:errorcluster)
            n111 = Bundle By Name(cluster=w350, "PQ Software Information.# Modules"=w345) -> (w353:T2)
          }
          frame -1 {
            # "Tag not found"
          }
        }
      }
      frame "CreatorSW_ModuleName" {
        n112 = Format Into String(w364) -> (resulting string=w374:string)  [unwired: 3 in, 1 out]
        n113 = Search 1D Array(1D array=w370, element=w374) -> (index of element=w373:i32)  [unwired: 1 in]
        n114 = case shown="0, Default" w373 {
          selector: w373 -> [w387 _]
          tunnel: w372 -> [w383 w397]
          tunnel: [w386 w397] -> w371
          tunnel: w370 -> [w391 w396]
          tunnel: [w390 w396] -> w369
          tunnel: w368 -> [w389 w395]
          tunnel: [w388 w395] -> w367
          tunnel: [w380 w394] -> w366
          tunnel: w365 -> [w381 w394]
          tunnel: w364 -> [w375 w393]
          tunnel: [w375 w392] -> w363
          frame 0, Default {
            # "Tag found"
            n115 = Delete From Array(array=w391, index=w387) -> (array with subset deleted=w390:string[])  [unwired: 1 in, 1 out]
            n116 = Delete From Array(array=w389, index=w387) -> (deleted portion=w385:T1, array with subset deleted=w388:T1[])  [unwired: 1 in]
            n117 = Unbundle By Name(w383) -> ("PQ Software Information.Module Names"=w382:string[])
            n118 = call "Decode Single Tag.vi"("Error In"=w381, "PicoQuant Tag"=w385) -> ("Error Out"=w384:errorcluster, "Variant"=w379:variant)  [unwired: 8 in]
            n119 = Variant To Data(error in=w384, type=" ", Variant=w379) -> (data=w377:string, error out=w380:errorcluster)
            n120 = Build Array (concatenate)(w382, w377) -> (w376:string[])
            n121 = Bundle By Name(cluster=w383, "PQ Software Information.Module Names"=w376) -> (w386:T2)
          }
          frame -1 {
            # "Tag not found"
            n122 = Increment(x=w393) -> (x+1=w392:T15)
          }
        }
      }
      frame "CreatorSW_ModuleVers" {
        n123 = Format Into String(w399) -> (resulting string=w409:string)  [unwired: 3 in, 1 out]
        n124 = Search 1D Array(1D array=w405, element=w409) -> (index of element=w408:i32)  [unwired: 1 in]
        n125 = case shown="-1" w408 {
          selector: w408 -> [w422 _]
          tunnel: w407 -> [w418 w432]
          tunnel: [w421 w432] -> w406
          tunnel: w405 -> [w426 w431]
          tunnel: [w425 w431] -> w404
          tunnel: w403 -> [w424 w430]
          tunnel: [w423 w430] -> w402
          tunnel: [w415 w429] -> w401
          tunnel: w400 -> [w416 w429]
          tunnel: w399 -> [w410 w428]
          tunnel: [w410 w427] -> w398
          frame 0, Default {
            # "Tag found"
            n126 = Delete From Array(array=w426, index=w422) -> (array with subset deleted=w425:string[])  [unwired: 1 in, 1 out]
            n127 = Delete From Array(array=w424, index=w422) -> (deleted portion=w420:T1, array with subset deleted=w423:T1[])  [unwired: 1 in]
            n128 = Unbundle By Name(w418) -> ("PQ Software Information.Module Versions"=w417:string[])
            n129 = call "Decode Single Tag.vi"("Error In"=w416, "PicoQuant Tag"=w420) -> ("Error Out"=w419:errorcluster, "Variant"=w414:variant)  [unwired: 8 in]
            n130 = Variant To Data(error in=w419, type=" ", Variant=w414) -> (data=w412:string, error out=w415:errorcluster)
            n131 = Build Array (concatenate)(w417, w412) -> (w411:string[])
            n132 = Bundle By Name(cluster=w418, "PQ Software Information.Module Versions"=w411) -> (w421:T2)
          }
          frame -1 {
            # "Tag not found"
            n133 = Increment(x=w428) -> (x+1=w427:T15)
          }
        }
      }
      frame "CreatorSW_SVNBuild" {
        n134 = Format Into String(w434) -> (resulting string=w444:string)  [unwired: 3 in, 1 out]
        n135 = Increment(x=w434) -> (x+1=w433:T15)
        n136 = Search 1D Array(1D array=w440, element=w444) -> (index of element=w443:i32)  [unwired: 1 in]
        n137 = case shown="0, Default" w443 {
          selector: w443 -> [w454 _]
          tunnel: w442 -> [w450 w462]
          tunnel: [w453 w462] -> w441
          tunnel: w440 -> [w458 w461]
          tunnel: [w457 w461] -> w439
          tunnel: w438 -> [w456 w460]
          tunnel: [w455 w460] -> w437
          tunnel: [w448 w459] -> w436
          tunnel: w435 -> [w449 w459]
          frame 0, Default {
            # "Tag found"
            n138 = Delete From Array(array=w458, index=w454) -> (array with subset deleted=w457:string[])  [unwired: 1 in, 1 out]
            n139 = Delete From Array(array=w456, index=w454) -> (deleted portion=w452:T1, array with subset deleted=w455:T1[])  [unwired: 1 in]
            n140 = Unbundle By Name(w450) -> ("PQ Software Information.SVN Build"=w446:i64)
            n141 = call "Decode Single Tag.vi"("Error In"=w449, "PicoQuant Tag"=w452) -> ("Error Out"=w451:errorcluster, "Variant"=w447:variant)  [unwired: 8 in]
            n142 = Variant To Data(error in=w451, type=w446, Variant=w447) -> (data=w445:i64, error out=w448:errorcluster)
            n143 = Bundle By Name(cluster=w450, "PQ Software Information.SVN Build"=w445) -> (w453:T2)
          }
          frame -1 {
            # "Tag not found"
          }
        }
      }
      frame "<Remote Request Data>" {
        n144 = Increment(x=w464) -> (x+1=w463:T15)
      }
      frame "$StartedByRemoteInterface" {
        n145 = Format Into String(w470) -> (resulting string=w480:string)  [unwired: 3 in, 1 out]
        n146 = Increment(x=w470) -> (x+1=w469:T15)
        n147 = Search 1D Array(1D array=w476, element=w480) -> (index of element=w479:i32)  [unwired: 1 in]
        n148 = case shown="0, Default" w479 {
          selector: w479 -> [w490 _]
          tunnel: w478 -> [w486 w498]
          tunnel: [w489 w498] -> w477
          tunnel: w476 -> [w494 w497]
          tunnel: [w493 w497] -> w475
          tunnel: w474 -> [w492 w496]
          tunnel: [w491 w496] -> w473
          tunnel: [w484 w495] -> w472
          tunnel: w471 -> [w485 w495]
          frame 0, Default {
            # "Tag found"
            n149 = Unbundle By Name(w486) -> ("PQ Remote Request Information.Started by Remote Interface"=w482:bool)
            n150 = Delete From Array(array=w494, index=w490) -> (array with subset deleted=w493:string[])  [unwired: 1 in, 1 out]
            n151 = Delete From Array(array=w492, index=w490) -> (deleted portion=w488:T1, array with subset deleted=w491:T1[])  [unwired: 1 in]
            n152 = call "Decode Single Tag.vi"("Error In"=w485, "PicoQuant Tag"=w488) -> ("Error Out"=w487:errorcluster, "Variant"=w483:variant)  [unwired: 8 in]
            n153 = Variant To Data(error in=w487, type=w482, Variant=w483) -> (data=w481:bool, error out=w484:errorcluster)
            n154 = Bundle By Name(cluster=w486, "PQ Remote Request Information.Started by Remote Interface"=w481) -> (w489:T2)
          }
          frame -1 {
            # "Tag not found"
          }
        }
      }
      frame "<Remote Request Header mand.>" {
        n155 = Increment(x=w500) -> (x+1=w499:T15)
      }
      frame "$ReqHdr_MeasurementType" {
        n156 = Format Into String(w506) -> (resulting string=w516:string)  [unwired: 3 in, 1 out]
        n157 = Increment(x=w506) -> (x+1=w505:T15)
        n158 = Search 1D Array(1D array=w512, element=w516) -> (index of element=w515:i32)  [unwired: 1 in]
        n159 = case shown="0, Default" w515 {
          selector: w515 -> [w526 _]
          tunnel: w514 -> [w522 w534]
          tunnel: [w525 w534] -> w513
          tunnel: w512 -> [w530 w533]
          tunnel: [w529 w533] -> w511
          tunnel: w510 -> [w528 w532]
          tunnel: [w527 w532] -> w509
          tunnel: [w520 w531] -> w508
          tunnel: w507 -> [w521 w531]
          frame 0, Default {
            # "Tag found"
            n160 = Delete From Array(array=w530, index=w526) -> (array with subset deleted=w529:string[])  [unwired: 1 in, 1 out]
            n161 = Delete From Array(array=w528, index=w526) -> (deleted portion=w524:T1, array with subset deleted=w527:T1[])  [unwired: 1 in]
            n162 = Unbundle By Name(w522) -> ("PQ Remote Request Information.Measurement Type"=w518:i64)
            n163 = call "Decode Single Tag.vi"("Error In"=w521, "PicoQuant Tag"=w524) -> ("Error Out"=w523:errorcluster, "Variant"=w519:variant)  [unwired: 8 in]
            n164 = Variant To Data(error in=w523, type=w518, Variant=w519) -> (data=w517:i64, error out=w520:errorcluster)
            n165 = Bundle By Name(cluster=w522, "PQ Remote Request Information.Measurement Type"=w517) -> (w525:T2)
          }
          frame -1 {
            # "Tag not found"
          }
        }
      }
      frame "$ReqHdr_PixelNumber_X" {
        n166 = Format Into String(w536) -> (resulting string=w546:string)  [unwired: 3 in, 1 out]
        n167 = Increment(x=w536) -> (x+1=w535:T15)
        n168 = Search 1D Array(1D array=w542, element=w546) -> (index of element=w545:i32)  [unwired: 1 in]
        n169 = case shown="0, Default" w545 {
          selector: w545 -> [w556 _]
          tunnel: w544 -> [w552 w564]
          tunnel: [w555 w564] -> w543
          tunnel: w542 -> [w560 w563]
          tunnel: [w559 w563] -> w541
          tunnel: w540 -> [w558 w562]
          tunnel: [w557 w562] -> w539
          tunnel: [w550 w561] -> w538
          tunnel: w537 -> [w551 w561]
          frame 0, Default {
            # "Tag found"
            n170 = Delete From Array(array=w560, index=w556) -> (array with subset deleted=w559:string[])  [unwired: 1 in, 1 out]
            n171 = Delete From Array(array=w558, index=w556) -> (deleted portion=w554:T1, array with subset deleted=w557:T1[])  [unwired: 1 in]
            n172 = call "Decode Single Tag.vi"("Error In"=w551, "PicoQuant Tag"=w554) -> ("Error Out"=w553:errorcluster, "Variant"=w549:variant)  [unwired: 8 in]
            n173 = Unbundle By Name(w552) -> ("PQ Remote Request Information.# Pixel X"=w548:i64)
            n174 = Variant To Data(error in=w553, type=w548, Variant=w549) -> (data=w547:i64, error out=w550:errorcluster)
            n175 = Bundle By Name(cluster=w552, "PQ Remote Request Information.# Pixel X"=w547) -> (w555:T2)
          }
          frame -1 {
            # "Tag not found"
          }
        }
      }
      frame "$ReqHdr_PixelNumber_Y" {
        n176 = Format Into String(w566) -> (resulting string=w576:string)  [unwired: 3 in, 1 out]
        n177 = Increment(x=w566) -> (x+1=w565:T15)
        n178 = Search 1D Array(1D array=w572, element=w576) -> (index of element=w575:i32)  [unwired: 1 in]
        n179 = case shown="0, Default" w575 {
          selector: w575 -> [w586 _]
          tunnel: w574 -> [w582 w594]
          tunnel: [w585 w594] -> w573
          tunnel: w572 -> [w590 w593]
          tunnel: [w589 w593] -> w571
          tunnel: w570 -> [w588 w592]
          tunnel: [w587 w592] -> w569
          tunnel: [w580 w591] -> w568
          tunnel: w567 -> [w581 w591]
          frame 0, Default {
            # "Tag found"
            n180 = Delete From Array(array=w590, index=w586) -> (array with subset deleted=w589:string[])  [unwired: 1 in, 1 out]
            n181 = Delete From Array(array=w588, index=w586) -> (deleted portion=w584:T1, array with subset deleted=w587:T1[])  [unwired: 1 in]
            n182 = call "Decode Single Tag.vi"("Error In"=w581, "PicoQuant Tag"=w584) -> ("Error Out"=w583:errorcluster, "Variant"=w579:variant)  [unwired: 8 in]
            n183 = Unbundle By Name(w582) -> ("PQ Remote Request Information.# Pixel Y"=w578:i64)
            n184 = Variant To Data(error in=w583, type=w578, Variant=w579) -> (data=w577:i64, error out=w580:errorcluster)
            n185 = Bundle By Name(cluster=w582, "PQ Remote Request Information.# Pixel Y"=w577) -> (w585:T2)
          }
          frame -1 {
            # "Tag not found"
          }
        }
      }
      frame "$ReqHdr_RecordVersion" {
        n186 = Format Into String(w596) -> (resulting string=w606:string)  [unwired: 3 in, 1 out]
        n187 = Increment(x=w596) -> (x+1=w595:T15)
        n188 = Search 1D Array(1D array=w602, element=w606) -> (index of element=w605:i32)  [unwired: 1 in]
        n189 = case shown="0, Default" w605 {
          selector: w605 -> [w616 _]
          tunnel: w604 -> [w612 w624]
          tunnel: [w615 w624] -> w603
          tunnel: w602 -> [w620 w623]
          tunnel: [w619 w623] -> w601
          tunnel: w600 -> [w618 w622]
          tunnel: [w617 w622] -> w599
          tunnel: [w610 w621] -> w598
          tunnel: w597 -> [w611 w621]
          frame 0, Default {
            # "Tag found"
            n190 = Delete From Array(array=w620, index=w616) -> (array with subset deleted=w619:string[])  [unwired: 1 in, 1 out]
            n191 = Delete From Array(array=w618, index=w616) -> (deleted portion=w614:T1, array with subset deleted=w617:T1[])  [unwired: 1 in]
            n192 = Unbundle By Name(w612) -> ("PQ Remote Request Information.Record Version"=w608:i64)
            n193 = call "Decode Single Tag.vi"("Error In"=w611, "PicoQuant Tag"=w614) -> ("Error Out"=w613:errorcluster, "Variant"=w609:variant)  [unwired: 8 in]
            n194 = Variant To Data(error in=w613, type=w608, Variant=w609) -> (data=w607:i64, error out=w610:errorcluster)
            n195 = Bundle By Name(cluster=w612, "PQ Remote Request Information.Record Version"=w607) -> (w615:T2)
          }
          frame -1 {
            # "Tag not found"
          }
        }
      }
      frame "$ReqHdr_ScanningPattern" {
        n196 = Format Into String(w626) -> (resulting string=w636:string)  [unwired: 3 in, 1 out]
        n197 = Increment(x=w626) -> (x+1=w625:T15)
        n198 = Search 1D Array(1D array=w632, element=w636) -> (index of element=w635:i32)  [unwired: 1 in]
        n199 = case shown="0, Default" w635 {
          selector: w635 -> [w646 _]
          tunnel: w634 -> [w642 w654]
          tunnel: [w645 w654] -> w633
          tunnel: w632 -> [w650 w653]
          tunnel: [w649 w653] -> w631
          tunnel: w630 -> [w648 w652]
          tunnel: [w647 w652] -> w629
          tunnel: [w640 w651] -> w628
          tunnel: w627 -> [w641 w651]
          frame 0, Default {
            # "Tag found"
            n200 = Delete From Array(array=w650, index=w646) -> (array with subset deleted=w649:string[])  [unwired: 1 in, 1 out]
            n201 = Delete From Array(array=w648, index=w646) -> (deleted portion=w644:T1, array with subset deleted=w647:T1[])  [unwired: 1 in]
            n202 = Unbundle By Name(w642) -> ("PQ Remote Request Information.Scanning Pattern"=w638:i64)
            n203 = call "Decode Single Tag.vi"("Error In"=w641, "PicoQuant Tag"=w644) -> ("Error Out"=w643:errorcluster, "Variant"=w639:variant)  [unwired: 8 in]
            n204 = Variant To Data(error in=w643, type=w638, Variant=w639) -> (data=w637:i64, error out=w640:errorcluster)
            n205 = Bundle By Name(cluster=w642, "PQ Remote Request Information.Scanning Pattern"=w637) -> (w645:T2)
          }
          frame -1 {
            # "Tag not found"
          }
        }
      }
      frame "$ReqHdr_SpatialResolution" {
        n206 = Format Into String(w656) -> (resulting string=w666:string)  [unwired: 3 in, 1 out]
        n207 = Increment(x=w656) -> (x+1=w655:T15)
        n208 = Search 1D Array(1D array=w662, element=w666) -> (index of element=w665:i32)  [unwired: 1 in]
        n209 = case shown="0, Default" w665 {
          selector: w665 -> [w676 _]
          tunnel: w664 -> [w672 w684]
          tunnel: [w675 w684] -> w663
          tunnel: w662 -> [w680 w683]
          tunnel: [w679 w683] -> w661
          tunnel: w660 -> [w678 w682]
          tunnel: [w677 w682] -> w659
          tunnel: [w670 w681] -> w658
          tunnel: w657 -> [w671 w681]
          frame 0, Default {
            # "Tag found"
            n210 = Delete From Array(array=w680, index=w676) -> (array with subset deleted=w679:string[])  [unwired: 1 in, 1 out]
            n211 = Delete From Array(array=w678, index=w676) -> (deleted portion=w674:T1, array with subset deleted=w677:T1[])  [unwired: 1 in]
            n212 = Unbundle By Name(w672) -> ("PQ Remote Request Information.Scanning Resolution (m/px)"=w668:dbl)
            n213 = call "Decode Single Tag.vi"("Error In"=w671, "PicoQuant Tag"=w674) -> ("Error Out"=w673:errorcluster, "Variant"=w669:variant)  [unwired: 8 in]
            n214 = Variant To Data(error in=w673, type=w668, Variant=w669) -> (data=w667:dbl, error out=w670:errorcluster)
            n215 = Bundle By Name(cluster=w672, "PQ Remote Request Information.Scanning Resolution (m/px)"=w667) -> (w675:T2)
          }
          frame -1 {
            # "Tag not found"
          }
        }
      }
      frame "<Remote Request Header opt.>" {
        n216 = Increment(x=w686) -> (x+1=w685:T15)
      }
      frame "$Comment" {
        n217 = Format Into String(w692) -> (resulting string=w702:string)  [unwired: 3 in, 1 out]
        n218 = Increment(x=w692) -> (x+1=w691:T15)
        n219 = Search 1D Array(1D array=w698, element=w702) -> (index of element=w701:i32)  [unwired: 1 in]
        n220 = case shown="0, Default" w701 {
          selector: w701 -> [w712 _]
          tunnel: w700 -> [w708 w720]
          tunnel: [w711 w720] -> w699
          tunnel: w698 -> [w716 w719]
          tunnel: [w715 w719] -> w697
          tunnel: w696 -> [w714 w718]
          tunnel: [w713 w718] -> w695
          tunnel: [w706 w717] -> w694
          tunnel: w693 -> [w707 w717]
          frame 0, Default {
            # "Tag found"
            n221 = Delete From Array(array=w716, index=w712) -> (array with subset deleted=w715:string[])  [unwired: 1 in, 1 out]
            n222 = Delete From Array(array=w714, index=w712) -> (deleted portion=w710:T1, array with subset deleted=w713:T1[])  [unwired: 1 in]
            n223 = call "Decode Single Tag.vi"("Error In"=w707, "PicoQuant Tag"=w710) -> ("Error Out"=w709:errorcluster, "Variant"=w705:variant)  [unwired: 8 in]
            n224 = Unbundle By Name(w708) -> ("PQ Remote Request Information.Comment"=w704:string)
            n225 = Variant To Data(error in=w709, type=w704, Variant=w705) -> (data=w703:string, error out=w706:errorcluster)
            n226 = Bundle By Name(cluster=w708, "PQ Remote Request Information.Comment"=w703) -> (w711:T2)
          }
          frame -1 {
            # "Tag not found"
          }
        }
      }
      frame "$Filename" {
        n227 = Format Into String(w722) -> (resulting string=w732:string)  [unwired: 3 in, 1 out]
        n228 = Increment(x=w722) -> (x+1=w721:T15)
        n229 = Search 1D Array(1D array=w728, element=w732) -> (index of element=w731:i32)  [unwired: 1 in]
        n230 = case shown="0, Default" w731 {
          selector: w731 -> [w742 _]
          tunnel: w730 -> [w738 w750]
          tunnel: [w741 w750] -> w729
          tunnel: w728 -> [w746 w749]
          tunnel: [w745 w749] -> w727
          tunnel: w726 -> [w744 w748]
          tunnel: [w743 w748] -> w725
          tunnel: [w736 w747] -> w724
          tunnel: w723 -> [w737 w747]
          frame 0, Default {
            # "Tag found"
            n231 = Delete From Array(array=w746, index=w742) -> (array with subset deleted=w745:string[])  [unwired: 1 in, 1 out]
            n232 = Delete From Array(array=w744, index=w742) -> (deleted portion=w740:T1, array with subset deleted=w743:T1[])  [unwired: 1 in]
            n233 = call "Decode Single Tag.vi"("Error In"=w737, "PicoQuant Tag"=w740) -> ("Error Out"=w739:errorcluster, "Variant"=w735:variant)  [unwired: 8 in]
            n234 = Unbundle By Name(w738) -> ("PQ Remote Request Information.File Name"=w734:string)
            n235 = Variant To Data(error in=w739, type=w734, Variant=w735) -> (data=w733:string, error out=w736:errorcluster)
            n236 = Bundle By Name(cluster=w738, "PQ Remote Request Information.File Name"=w733) -> (w741:T2)
          }
          frame -1 {
            # "Tag not found"
          }
        }
      }
      frame "$Groupname" {
        n237 = Format Into String(w752) -> (resulting string=w762:string)  [unwired: 3 in, 1 out]
        n238 = Increment(x=w752) -> (x+1=w751:T15)
        n239 = Search 1D Array(1D array=w758, element=w762) -> (index of element=w761:i32)  [unwired: 1 in]
        n240 = case shown="0, Default" w761 {
          selector: w761 -> [w772 _]
          tunnel: w760 -> [w768 w780]
          tunnel: [w771 w780] -> w759
          tunnel: w758 -> [w776 w779]
          tunnel: [w775 w779] -> w757
          tunnel: w756 -> [w774 w778]
          tunnel: [w773 w778] -> w755
          tunnel: [w766 w777] -> w754
          tunnel: w753 -> [w767 w777]
          frame 0, Default {
            # "Tag found"
            n241 = Delete From Array(array=w776, index=w772) -> (array with subset deleted=w775:string[])  [unwired: 1 in, 1 out]
            n242 = Delete From Array(array=w774, index=w772) -> (deleted portion=w770:T1, array with subset deleted=w773:T1[])  [unwired: 1 in]
            n243 = call "Decode Single Tag.vi"("Error In"=w767, "PicoQuant Tag"=w770) -> ("Error Out"=w769:errorcluster, "Variant"=w765:variant)  [unwired: 8 in]
            n244 = Unbundle By Name(w768) -> ("PQ Remote Request Information.Group Name"=w764:string)
            n245 = Variant To Data(error in=w769, type=w764, Variant=w765) -> (data=w763:string, error out=w766:errorcluster)
            n246 = Bundle By Name(cluster=w768, "PQ Remote Request Information.Group Name"=w763) -> (w771:T2)
          }
          frame -1 {
            # "Tag not found"
          }
        }
      }
      frame "<Remote Request Header undef.>" {
        n247 = Increment(x=w782) -> (x+1=w781:T15)
      }
      frame "$<Ident>" {
        n248 = Increment(x=w788) -> (x+1=w787:T15)
      }
      frame "<Hardware Header>" {
        n249 = Increment(x=w794) -> (x+1=w793:T15)
      }
      frame "HW_InpChannels" {
        n250 = Format Into String(w800) -> (resulting string=w810:string)  [unwired: 3 in, 1 out]
        n251 = Increment(x=w800) -> (x+1=w799:T15)
        n252 = Search 1D Array(1D array=w806, element=w810) -> (index of element=w809:i32)  [unwired: 1 in]
        n253 = case shown="0, Default" w809 {
          selector: w809 -> [w820 _]
          tunnel: w808 -> [w816 w828]
          tunnel: [w819 w828] -> w807
          tunnel: w806 -> [w824 w827]
          tunnel: [w823 w827] -> w805
          tunnel: w804 -> [w822 w826]
          tunnel: [w821 w826] -> w803
          tunnel: [w814 w825] -> w802
          tunnel: w801 -> [w815 w825]
          frame 0, Default {
            # "Tag found"
            n254 = Delete From Array(array=w824, index=w820) -> (array with subset deleted=w823:string[])  [unwired: 1 in, 1 out]
            n255 = Delete From Array(array=w822, index=w820) -> (deleted portion=w818:T1, array with subset deleted=w821:T1[])  [unwired: 1 in]
            n256 = call "Decode Single Tag.vi"("Error In"=w815, "PicoQuant Tag"=w818) -> ("Error Out"=w817:errorcluster, "Variant"=w813:variant)  [unwired: 8 in]
            n257 = Unbundle By Name(w816) -> ("PQ Hardware Information.Input Channels.# Input Channels"=w812:i64)
            n258 = Variant To Data(error in=w817, type=w812, Variant=w813) -> (data=w811:i64, error out=w814:errorcluster)
            n259 = Bundle By Name(cluster=w816, "PQ Hardware Information.Input Channels.# Input Channels"=w811) -> (w819:T2)
          }
          frame -1 {
            # "Tag not found"
          }
        }
      }
      frame "HWInpChan_CFDLevel" {
        n260 = Format Into String(w830) -> (resulting string=w840:string)  [unwired: 3 in, 1 out]
        n261 = Search 1D Array(1D array=w836, element=w840) -> (index of element=w839:i32)  [unwired: 1 in]
        n262 = case shown="-1" w839 {
          selector: w839 -> [w853 _]
          tunnel: w838 -> [w849 w863]
          tunnel: [w852 w863] -> w837
          tunnel: w836 -> [w857 w862]
          tunnel: [w856 w862] -> w835
          tunnel: w834 -> [w855 w861]
          tunnel: [w854 w861] -> w833
          tunnel: [w847 w860] -> w832
          tunnel: w831 -> [w848 w860]
          tunnel: w830 -> [w841 w859]
          tunnel: [w841 w858] -> w829
          frame 0, Default {
            # "Tag found"
            n263 = Delete From Array(array=w857, index=w853) -> (array with subset deleted=w856:string[])  [unwired: 1 in, 1 out]
            n264 = Delete From Array(array=w855, index=w853) -> (deleted portion=w851:T1, array with subset deleted=w854:T1[])  [unwired: 1 in]
            n265 = call "Decode Single Tag.vi"("Error In"=w848, "PicoQuant Tag"=w851) -> ("Error Out"=w850:errorcluster, "Variant"=w846:variant)  [unwired: 8 in]
            n266 = Unbundle By Name(w849) -> ("PQ Hardware Information.Input Channels.CFD Levels (mV)"=w845:i64[])
            n267 = Variant To Data(error in=w850, type=i64 0 ("array"), Variant=w846) -> (data=w842:i64, error out=w847:errorcluster)
            n268 = Build Array (concatenate)(w845, w842) -> (w844:i64[])
            n269 = Bundle By Name(cluster=w849, "PQ Hardware Information.Input Channels.CFD Levels (mV)"=w844) -> (w852:T2)
          }
          frame -1 {
            # "Tag not found"
            n270 = Increment(x=w859) -> (x+1=w858:T15)
          }
        }
      }
      frame "HWInpChan_CFDZeroCross" {
        n271 = Format Into String(w865) -> (resulting string=w875:string)  [unwired: 3 in, 1 out]
        n272 = Search 1D Array(1D array=w871, element=w875) -> (index of element=w874:i32)  [unwired: 1 in]
        n273 = case shown="-1" w874 {
          selector: w874 -> [w888 _]
          tunnel: w873 -> [w884 w898]
          tunnel: [w887 w898] -> w872
          tunnel: w871 -> [w892 w897]
          tunnel: [w891 w897] -> w870
          tunnel: w869 -> [w890 w896]
          tunnel: [w889 w896] -> w868
          tunnel: [w882 w895] -> w867
          tunnel: w866 -> [w883 w895]
          tunnel: w865 -> [w876 w894]
          tunnel: [w876 w893] -> w864
          frame 0, Default {
            # "Tag found"
            n274 = Delete From Array(array=w892, index=w888) -> (array with subset deleted=w891:string[])  [unwired: 1 in, 1 out]
            n275 = Delete From Array(array=w890, index=w888) -> (deleted portion=w886:T1, array with subset deleted=w889:T1[])  [unwired: 1 in]
            n276 = Unbundle By Name(w884) -> ("PQ Hardware Information.Input Channels.CFD Zero Crossings (mV)"=w880:i64[])
            n277 = call "Decode Single Tag.vi"("Error In"=w883, "PicoQuant Tag"=w886) -> ("Error Out"=w885:errorcluster, "Variant"=w881:variant)  [unwired: 8 in]
            n278 = Variant To Data(error in=w885, type=i64 0 ("array"), Variant=w881) -> (data=w877:i64, error out=w882:errorcluster)
            n279 = Build Array (concatenate)(w880, w877) -> (w879:i64[])
            n280 = Bundle By Name(cluster=w884, "PQ Hardware Information.Input Channels.CFD Zero Crossings (mV)"=w879) -> (w887:T2)
          }
          frame -1 {
            # "Tag not found"
            n281 = Increment(x=w894) -> (x+1=w893:T15)
          }
        }
      }
      frame "HWInpChan_Enabled" {
        n282 = Format Into String(w900) -> (resulting string=w910:string)  [unwired: 3 in, 1 out]
        n283 = Search 1D Array(1D array=w906, element=w910) -> (index of element=w909:i32)  [unwired: 1 in]
        n284 = case shown="-1" w909 {
          selector: w909 -> [w923 _]
          tunnel: w908 -> [w919 w933]
          tunnel: [w922 w933] -> w907
          tunnel: w906 -> [w927 w932]
          tunnel: [w926 w932] -> w905
          tunnel: w904 -> [w925 w931]
          tunnel: [w924 w931] -> w903
          tunnel: [w917 w930] -> w902
          tunnel: w901 -> [w918 w930]
          tunnel: w900 -> [w911 w929]
          tunnel: [w911 w928] -> w899
          frame 0, Default {
            # "Tag found"
            n285 = Delete From Array(array=w927, index=w923) -> (array with subset deleted=w926:string[])  [unwired: 1 in, 1 out]
            n286 = Delete From Array(array=w925, index=w923) -> (deleted portion=w921:T1, array with subset deleted=w924:T1[])  [unwired: 1 in]
            n287 = call "Decode Single Tag.vi"("Error In"=w918, "PicoQuant Tag"=w921) -> ("Error Out"=w920:errorcluster, "Variant"=w916:variant)  [unwired: 8 in]
            n288 = Unbundle By Name(w919) -> ("PQ Hardware Information.Input Channels.CFD Channel Enabled"=w915:bool[])
            n289 = Variant To Data(error in=w920, type=FALSE, Variant=w916) -> (data=w912:bool, error out=w917:errorcluster)
            n290 = Build Array (concatenate)(w915, w912) -> (w914:bool[])
            n291 = Bundle By Name(cluster=w919, "PQ Hardware Information.Input Channels.CFD Channel Enabled"=w914) -> (w922:T2)
          }
          frame -1 {
            # "Tag not found"
            n292 = Increment(x=w929) -> (x+1=w928:T15)
          }
        }
      }
      frame "HWInpChan_ModuleIdx" {
        n293 = Format Into String(w935) -> (resulting string=w945:string)  [unwired: 3 in, 1 out]
        n294 = Search 1D Array(1D array=w941, element=w945) -> (index of element=w944:i32)  [unwired: 1 in]
        n295 = case shown="-1" w944 {
          selector: w944 -> [w958 _]
          tunnel: w943 -> [w954 w968]
          tunnel: [w957 w968] -> w942
          tunnel: w941 -> [w962 w967]
          tunnel: [w961 w967] -> w940
          tunnel: w939 -> [w960 w966]
          tunnel: [w959 w966] -> w938
          tunnel: [w952 w965] -> w937
          tunnel: w936 -> [w953 w965]
          tunnel: w935 -> [w946 w964]
          tunnel: [w946 w963] -> w934
          frame 0, Default {
            # "Tag found"
            n296 = Delete From Array(array=w962, index=w958) -> (array with subset deleted=w961:string[])  [unwired: 1 in, 1 out]
            n297 = Delete From Array(array=w960, index=w958) -> (deleted portion=w956:T1, array with subset deleted=w959:T1[])  [unwired: 1 in]
            n298 = call "Decode Single Tag.vi"("Error In"=w953, "PicoQuant Tag"=w956) -> ("Error Out"=w955:errorcluster, "Variant"=w951:variant)  [unwired: 8 in]
            n299 = Unbundle By Name(w954) -> ("PQ Hardware Information.Input Channels.Module Indices"=w950:i64[])
            n300 = Variant To Data(error in=w955, type=i64 0 ("PQ Hardware Information.Input Channels.Module Indices"), Variant=w951) -> (data=w948:i64, error out=w952:errorcluster)
            n301 = Build Array (concatenate)(w950, w948) -> (w949:i64[])
            n302 = Bundle By Name(cluster=w954, "PQ Hardware Information.Input Channels.Module Indices"=w949) -> (w957:T2)
          }
          frame -1 {
            # "Tag not found"
            n303 = Increment(x=w964) -> (x+1=w963:T15)
          }
        }
      }
      frame "HWInpChan_Offset" {
        n304 = Format Into String(w970) -> (resulting string=w980:string)  [unwired: 3 in, 1 out]
        n305 = Search 1D Array(1D array=w976, element=w980) -> (index of element=w979:i32)  [unwired: 1 in]
        n306 = case shown="-1" w979 {
          selector: w979 -> [w993 _]
          tunnel: w978 -> [w989 w1003]
          tunnel: [w992 w1003] -> w977
          tunnel: w976 -> [w997 w1002]
          tunnel: [w996 w1002] -> w975
          tunnel: w974 -> [w995 w1001]
          tunnel: [w994 w1001] -> w973
          tunnel: [w987 w1000] -> w972
          tunnel: w971 -> [w988 w1000]
          tunnel: w970 -> [w981 w999]
          tunnel: [w981 w998] -> w969
          frame 0, Default {
            # "Tag found"
            n307 = Delete From Array(array=w997, index=w993) -> (array with subset deleted=w996:string[])  [unwired: 1 in, 1 out]
            n308 = Delete From Array(array=w995, index=w993) -> (deleted portion=w991:T1, array with subset deleted=w994:T1[])  [unwired: 1 in]
            n309 = call "Decode Single Tag.vi"("Error In"=w988, "PicoQuant Tag"=w991) -> ("Error Out"=w990:errorcluster, "Variant"=w986:variant)  [unwired: 8 in]
            n310 = Unbundle By Name(w989) -> ("PQ Hardware Information.Input Channels.Offsets (ps)"=w985:i64[])
            n311 = Variant To Data(error in=w990, type=i64 0 ("PQ Hardware Information.Input Channels.Module Indices"), Variant=w986) -> (data=w983:i64, error out=w987:errorcluster)
            n312 = Build Array (concatenate)(w985, w983) -> (w984:i64[])
            n313 = Bundle By Name(cluster=w989, "PQ Hardware Information.Input Channels.Offsets (ps)"=w984) -> (w992:T2)
          }
          frame -1 {
            # "Tag not found"
            n314 = Increment(x=w999) -> (x+1=w998:T15)
          }
        }
      }
      frame "HWInpChan_TdCode" {
        n315 = Format Into String(w1005) -> (resulting string=w1015:string)  [unwired: 3 in, 1 out]
        n316 = Search 1D Array(1D array=w1011, element=w1015) -> (index of element=w1014:i32)  [unwired: 1 in]
        n317 = case shown="-1" w1014 {
          selector: w1014 -> [w1028 _]
          tunnel: w1013 -> [w1024 w1038]
          tunnel: [w1027 w1038] -> w1012
          tunnel: w1011 -> [w1032 w1037]
          tunnel: [w1031 w1037] -> w1010
          tunnel: w1009 -> [w1030 w1036]
          tunnel: [w1029 w1036] -> w1008
          tunnel: [w1022 w1035] -> w1007
          tunnel: w1006 -> [w1023 w1035]
          tunnel: w1005 -> [w1016 w1034]
          tunnel: [w1016 w1033] -> w1004
          frame 0, Default {
            # "Tag found"
            n318 = Delete From Array(array=w1032, index=w1028) -> (array with subset deleted=w1031:string[])  [unwired: 1 in, 1 out]
            n319 = Delete From Array(array=w1030, index=w1028) -> (deleted portion=w1026:T1, array with subset deleted=w1029:T1[])  [unwired: 1 in]
            n320 = call "Decode Single Tag.vi"("Error In"=w1023, "PicoQuant Tag"=w1026) -> ("Error Out"=w1025:errorcluster, "Variant"=w1021:variant)  [unwired: 8 in]
            n321 = Unbundle By Name(w1024) -> ("PQ Hardware Information.Input Channels.Td Codes"=w1020:i64[])
            n322 = Variant To Data(error in=w1025, type=i64 0 ("PQ Hardware Information.Input Channels.Module Indices"), Variant=w1021) -> (data=w1018:i64, error out=w1022:errorcluster)
            n323 = Build Array (concatenate)(w1020, w1018) -> (w1019:i64[])
            n324 = Bundle By Name(cluster=w1024, "PQ Hardware Information.Input Channels.Td Codes"=w1019) -> (w1027:T2)
          }
          frame -1 {
            # "Tag not found"
            n325 = Increment(x=w1034) -> (x+1=w1033:T15)
          }
        }
      }
      frame "HWInpChan_TrgEdge" {
        n326 = Format Into String(w1040) -> (resulting string=w1050:string)  [unwired: 3 in, 1 out]
        n327 = Search 1D Array(1D array=w1046, element=w1050) -> (index of element=w1049:i32)  [unwired: 1 in]
        n328 = case shown="-1" w1049 {
          selector: w1049 -> [w1063 _]
          tunnel: w1048 -> [w1059 w1073]
          tunnel: [w1062 w1073] -> w1047
          tunnel: w1046 -> [w1067 w1072]
          tunnel: [w1066 w1072] -> w1045
          tunnel: w1044 -> [w1065 w1071]
          tunnel: [w1064 w1071] -> w1043
          tunnel: [w1057 w1070] -> w1042
          tunnel: w1041 -> [w1058 w1070]
          tunnel: w1040 -> [w1051 w1069]
          tunnel: [w1051 w1068] -> w1039
          frame 0, Default {
            # "Tag found"
            n329 = Delete From Array(array=w1067, index=w1063) -> (array with subset deleted=w1066:string[])  [unwired: 1 in, 1 out]
            n330 = Delete From Array(array=w1065, index=w1063) -> (deleted portion=w1061:T1, array with subset deleted=w1064:T1[])  [unwired: 1 in]
            n331 = call "Decode Single Tag.vi"("Error In"=w1058, "PicoQuant Tag"=w1061) -> ("Error Out"=w1060:errorcluster, "Variant"=w1056:variant)  [unwired: 8 in]
            n332 = Unbundle By Name(w1059) -> ("PQ Hardware Information.Input Channels.Trigger Edges"=w1055:i64[])
            n333 = Variant To Data(error in=w1060, type=i64 0 ("PQ Hardware Information.Input Channels.Module Indices"), Variant=w1056) -> (data=w1053:i64, error out=w1057:errorcluster)
            n334 = Build Array (concatenate)(w1055, w1053) -> (w1054:i64[])
            n335 = Bundle By Name(cluster=w1059, "PQ Hardware Information.Input Channels.Trigger Edges"=w1054) -> (w1062:T2)
          }
          frame -1 {
            # "Tag not found"
            n336 = Increment(x=w1069) -> (x+1=w1068:T15)
          }
        }
      }
      frame "HWInpChan_TrgLevel" {
        n337 = Format Into String(w1075) -> (resulting string=w1085:string)  [unwired: 3 in, 1 out]
        n338 = Search 1D Array(1D array=w1081, element=w1085) -> (index of element=w1084:i32)  [unwired: 1 in]
        n339 = case shown="-1" w1084 {
          selector: w1084 -> [w1098 _]
          tunnel: w1083 -> [w1094 w1108]
          tunnel: [w1097 w1108] -> w1082
          tunnel: w1081 -> [w1102 w1107]
          tunnel: [w1101 w1107] -> w1080
          tunnel: w1079 -> [w1100 w1106]
          tunnel: [w1099 w1106] -> w1078
          tunnel: [w1092 w1105] -> w1077
          tunnel: w1076 -> [w1093 w1105]
          tunnel: w1075 -> [w1086 w1104]
          tunnel: [w1086 w1103] -> w1074
          frame 0, Default {
            # "Tag found"
            n340 = Delete From Array(array=w1102, index=w1098) -> (array with subset deleted=w1101:string[])  [unwired: 1 in, 1 out]
            n341 = Delete From Array(array=w1100, index=w1098) -> (deleted portion=w1096:T1, array with subset deleted=w1099:T1[])  [unwired: 1 in]
            n342 = call "Decode Single Tag.vi"("Error In"=w1093, "PicoQuant Tag"=w1096) -> ("Error Out"=w1095:errorcluster, "Variant"=w1091:variant)  [unwired: 8 in]
            n343 = Unbundle By Name(w1094) -> ("PQ Hardware Information.Input Channels.Trigger Levels (mV)"=w1090:i64[])
            n344 = Variant To Data(error in=w1095, type=i64 0 ("PQ Hardware Information.Input Channels.Module Indices"), Variant=w1091) -> (data=w1088:i64, error out=w1092:errorcluster)
            n345 = Build Array (concatenate)(w1090, w1088) -> (w1089:i64[])
            n346 = Bundle By Name(cluster=w1094, "PQ Hardware Information.Input Channels.Trigger Levels (mV)"=w1089) -> (w1097:T2)
          }
          frame -1 {
            # "Tag not found"
            n347 = Increment(x=w1104) -> (x+1=w1103:T15)
          }
        }
      }
      frame "HW_Markers" {
        n348 = Format Into String(w1110) -> (resulting string=w1120:string)  [unwired: 3 in, 1 out]
        n349 = Increment(x=w1110) -> (x+1=w1109:T15)
        n350 = Search 1D Array(1D array=w1116, element=w1120) -> (index of element=w1119:i32)  [unwired: 1 in]
        n351 = case shown="0, Default" w1119 {
          selector: w1119 -> [w1130 _]
          tunnel: w1118 -> [w1126 w1138]
          tunnel: [w1129 w1138] -> w1117
          tunnel: w1116 -> [w1134 w1137]
          tunnel: [w1133 w1137] -> w1115
          tunnel: w1114 -> [w1132 w1136]
          tunnel: [w1131 w1136] -> w1113
          tunnel: [w1124 w1135] -> w1112
          tunnel: w1111 -> [w1125 w1135]
          frame 0, Default {
            # "Tag found"
            n352 = Delete From Array(array=w1134, index=w1130) -> (array with subset deleted=w1133:string[])  [unwired: 1 in, 1 out]
            n353 = Delete From Array(array=w1132, index=w1130) -> (deleted portion=w1128:T1, array with subset deleted=w1131:T1[])  [unwired: 1 in]
            n354 = call "Decode Single Tag.vi"("Error In"=w1125, "PicoQuant Tag"=w1128) -> ("Error Out"=w1127:errorcluster, "Variant"=w1123:variant)  [unwired: 8 in]
            n355 = Unbundle By Name(w1126) -> ("PQ Hardware Information.Markers.# Markers"=w1121:i64)
            n356 = Variant To Data(error in=w1127, type=w1121, Variant=w1123) -> (data=w1122:i64, error out=w1124:errorcluster)
            n357 = Bundle By Name(cluster=w1126, "PQ Hardware Information.Markers.# Markers"=w1122) -> (w1129:T2)
          }
          frame -1 {
            # "Tag not found"
          }
        }
      }
      frame "HWMarkers_Enabled" {
        n358 = Format Into String(w1140) -> (resulting string=w1150:string)  [unwired: 3 in, 1 out]
        n359 = Search 1D Array(1D array=w1146, element=w1150) -> (index of element=w1149:i32)  [unwired: 1 in]
        n360 = case shown="-1" w1149 {
          selector: w1149 -> [w1163 _]
          tunnel: w1148 -> [w1159 w1173]
          tunnel: [w1162 w1173] -> w1147
          tunnel: w1146 -> [w1167 w1172]
          tunnel: [w1166 w1172] -> w1145
          tunnel: w1144 -> [w1165 w1171]
          tunnel: [w1164 w1171] -> w1143
          tunnel: [w1157 w1170] -> w1142
          tunnel: w1141 -> [w1158 w1170]
          tunnel: w1140 -> [w1151 w1169]
          tunnel: [w1151 w1168] -> w1139
          frame 0, Default {
            # "Tag found"
            n361 = Delete From Array(array=w1167, index=w1163) -> (array with subset deleted=w1166:string[])  [unwired: 1 in, 1 out]
            n362 = Delete From Array(array=w1165, index=w1163) -> (deleted portion=w1161:T1, array with subset deleted=w1164:T1[])  [unwired: 1 in]
            n363 = call "Decode Single Tag.vi"("Error In"=w1158, "PicoQuant Tag"=w1161) -> ("Error Out"=w1160:errorcluster, "Variant"=w1156:variant)  [unwired: 8 in]
            n364 = Unbundle By Name(w1159) -> ("PQ Hardware Information.Markers.Markers Enabled"=w1152:bool[])
            n365 = Variant To Data(error in=w1160, type=FALSE ("CFD Channel Enabled"), Variant=w1156) -> (data=w1153:bool, error out=w1157:errorcluster)
            n366 = Build Array (concatenate)(w1152, w1153) -> (w1155:bool[])
            n367 = Bundle By Name(cluster=w1159, "PQ Hardware Information.Markers.Markers Enabled"=w1155) -> (w1162:T2)
          }
          frame -1 {
            # "Tag not found"
            n368 = Increment(x=w1169) -> (x+1=w1168:T15)
          }
        }
      }
      frame "HWMarkers_HoldOff" {
        n369 = Format Into String(w1175) -> (resulting string=w1185:string)  [unwired: 3 in, 1 out]
        n370 = Increment(x=w1175) -> (x+1=w1174:T15)
        n371 = Search 1D Array(1D array=w1181, element=w1185) -> (index of element=w1184:i32)  [unwired: 1 in]
        n372 = case shown="0, Default" w1184 {
          selector: w1184 -> [w1195 _]
          tunnel: w1183 -> [w1191 w1203]
          tunnel: [w1194 w1203] -> w1182
          tunnel: w1181 -> [w1199 w1202]
          tunnel: [w1198 w1202] -> w1180
          tunnel: w1179 -> [w1197 w1201]
          tunnel: [w1196 w1201] -> w1178
          tunnel: [w1189 w1200] -> w1177
          tunnel: w1176 -> [w1190 w1200]
          frame 0, Default {
            # "Tag found"
            n373 = Delete From Array(array=w1199, index=w1195) -> (array with subset deleted=w1198:string[])  [unwired: 1 in, 1 out]
            n374 = Delete From Array(array=w1197, index=w1195) -> (deleted portion=w1193:T1, array with subset deleted=w1196:T1[])  [unwired: 1 in]
            n375 = call "Decode Single Tag.vi"("Error In"=w1190, "PicoQuant Tag"=w1193) -> ("Error Out"=w1192:errorcluster, "Variant"=w1188:variant)  [unwired: 8 in]
            n376 = Unbundle By Name(w1191) -> ("PQ Hardware Information.Markers.Holdoff (ns)"=w1186:i64)
            n377 = Variant To Data(error in=w1192, type=w1186, Variant=w1188) -> (data=w1187:i64, error out=w1189:errorcluster)
            n378 = Bundle By Name(cluster=w1191, "PQ Hardware Information.Markers.Holdoff (ns)"=w1187) -> (w1194:T2)
          }
          frame -1 {
            # "Tag not found"
          }
        }
      }
      frame "HWMarkers_RisingEdge" {
        n379 = Format Into String(w1205) -> (resulting string=w1215:string)  [unwired: 3 in, 1 out]
        n380 = Search 1D Array(1D array=w1211, element=w1215) -> (index of element=w1214:i32)  [unwired: 1 in]
        n381 = case shown="-1" w1214 {
          selector: w1214 -> [w1228 _]
          tunnel: w1213 -> [w1224 w1238]
          tunnel: [w1227 w1238] -> w1212
          tunnel: w1211 -> [w1232 w1237]
          tunnel: [w1231 w1237] -> w1210
          tunnel: w1209 -> [w1230 w1236]
          tunnel: [w1229 w1236] -> w1208
          tunnel: [w1222 w1235] -> w1207
          tunnel: w1206 -> [w1223 w1235]
          tunnel: w1205 -> [w1216 w1234]
          tunnel: [w1216 w1233] -> w1204
          frame 0, Default {
            # "Tag found"
            n382 = Delete From Array(array=w1232, index=w1228) -> (array with subset deleted=w1231:string[])  [unwired: 1 in, 1 out]
            n383 = Delete From Array(array=w1230, index=w1228) -> (deleted portion=w1226:T1, array with subset deleted=w1229:T1[])  [unwired: 1 in]
            n384 = call "Decode Single Tag.vi"("Error In"=w1223, "PicoQuant Tag"=w1226) -> ("Error Out"=w1225:errorcluster, "Variant"=w1221:variant)  [unwired: 8 in]
            n385 = Unbundle By Name(w1224) -> ("PQ Hardware Information.Markers.Rising Edges"=w1217:bool[])
            n386 = Variant To Data(error in=w1225, type=FALSE ("Rising Edge"), Variant=w1221) -> (data=w1218:bool, error out=w1222:errorcluster)
            n387 = Build Array (concatenate)(w1217, w1218) -> (w1220:bool[])
            n388 = Bundle By Name(cluster=w1224, "PQ Hardware Information.Markers.Rising Edges"=w1220) -> (w1227:T2)
          }
          frame -1 {
            # "Tag not found"
            n389 = Increment(x=w1234) -> (x+1=w1233:T15)
          }
        }
      }
      frame "HW_Modules" {
        n390 = Format Into String(w1240) -> (resulting string=w1250:string)  [unwired: 3 in, 1 out]
        n391 = Increment(x=w1240) -> (x+1=w1239:T15)
        n392 = Search 1D Array(1D array=w1246, element=w1250) -> (index of element=w1249:i32)  [unwired: 1 in]
        n393 = case shown="0, Default" w1249 {
          selector: w1249 -> [w1260 _]
          tunnel: w1248 -> [w1256 w1268]
          tunnel: [w1259 w1268] -> w1247
          tunnel: w1246 -> [w1264 w1267]
          tunnel: [w1263 w1267] -> w1245
          tunnel: w1244 -> [w1262 w1266]
          tunnel: [w1261 w1266] -> w1243
          tunnel: [w1254 w1265] -> w1242
          tunnel: w1241 -> [w1255 w1265]
          frame 0, Default {
            # "Tag found"
            n394 = Delete From Array(array=w1264, index=w1260) -> (array with subset deleted=w1263:string[])  [unwired: 1 in, 1 out]
            n395 = Delete From Array(array=w1262, index=w1260) -> (deleted portion=w1258:T1, array with subset deleted=w1261:T1[])  [unwired: 1 in]
            n396 = call "Decode Single Tag.vi"("Error In"=w1255, "PicoQuant Tag"=w1258) -> ("Error Out"=w1257:errorcluster, "Variant"=w1253:variant)  [unwired: 8 in]
            n397 = Unbundle By Name(w1256) -> ("PQ Hardware Information.Modules.# Modules"=w1252:i64)
            n398 = Variant To Data(error in=w1257, type=w1252, Variant=w1253) -> (data=w1251:i64, error out=w1254:errorcluster)
            n399 = Bundle By Name(cluster=w1256, "PQ Hardware Information.Modules.# Modules"=w1251) -> (w1259:T2)
          }
          frame -1 {
            # "Tag not found"
          }
        }
      }
      frame "HWModule_TypeCode" {
        n400 = Format Into String(w1270) -> (resulting string=w1280:string)  [unwired: 3 in, 1 out]
        n401 = Search 1D Array(1D array=w1276, element=w1280) -> (index of element=w1279:i32)  [unwired: 1 in]
        n402 = case shown="-1" w1279 {
          selector: w1279 -> [w1293 _]
          tunnel: w1278 -> [w1289 w1303]
          tunnel: [w1292 w1303] -> w1277
          tunnel: w1276 -> [w1297 w1302]
          tunnel: [w1296 w1302] -> w1275
          tunnel: w1274 -> [w1295 w1301]
          tunnel: [w1294 w1301] -> w1273
          tunnel: [w1287 w1300] -> w1272
          tunnel: w1271 -> [w1288 w1300]
          tunnel: w1270 -> [w1281 w1299]
          tunnel: [w1281 w1298] -> w1269
          frame 0, Default {
            # "Tag found"
            n403 = Delete From Array(array=w1297, index=w1293) -> (array with subset deleted=w1296:string[])  [unwired: 1 in, 1 out]
            n404 = Delete From Array(array=w1295, index=w1293) -> (deleted portion=w1291:T1, array with subset deleted=w1294:T1[])  [unwired: 1 in]
            n405 = call "Decode Single Tag.vi"("Error In"=w1288, "PicoQuant Tag"=w1291) -> ("Error Out"=w1290:errorcluster, "Variant"=w1286:variant)  [unwired: 8 in]
            n406 = Unbundle By Name(w1289) -> ("PQ Hardware Information.Modules.Type Codes"=w1283:i64[])
            n407 = Variant To Data(error in=w1290, type=i64 0 ("PQ Hardware Information.Modules.Type Codes"), Variant=w1286) -> (data=w1284:i64, error out=w1287:errorcluster)
            n408 = Build Array (concatenate)(w1283, w1284) -> (w1285:i64[])
            n409 = Bundle By Name(cluster=w1289, "PQ Hardware Information.Modules.Type Codes"=w1285) -> (w1292:T2)
          }
          frame -1 {
            # "Tag not found"
            n410 = Increment(x=w1299) -> (x+1=w1298:T15)
          }
        }
      }
      frame "HWModule_VersCode" {
        n411 = Format Into String(w1305) -> (resulting string=w1315:string)  [unwired: 3 in, 1 out]
        n412 = Search 1D Array(1D array=w1311, element=w1315) -> (index of element=w1314:i32)  [unwired: 1 in]
        n413 = case shown="-1" w1314 {
          selector: w1314 -> [w1328 _]
          tunnel: w1313 -> [w1324 w1338]
          tunnel: [w1327 w1338] -> w1312
          tunnel: w1311 -> [w1332 w1337]
          tunnel: [w1331 w1337] -> w1310
          tunnel: w1309 -> [w1330 w1336]
          tunnel: [w1329 w1336] -> w1308
          tunnel: [w1322 w1335] -> w1307
          tunnel: w1306 -> [w1323 w1335]
          tunnel: w1305 -> [w1316 w1334]
          tunnel: [w1316 w1333] -> w1304
          frame 0, Default {
            # "Tag found"
            n414 = Delete From Array(array=w1332, index=w1328) -> (array with subset deleted=w1331:string[])  [unwired: 1 in, 1 out]
            n415 = Delete From Array(array=w1330, index=w1328) -> (deleted portion=w1326:T1, array with subset deleted=w1329:T1[])  [unwired: 1 in]
            n416 = call "Decode Single Tag.vi"("Error In"=w1323, "PicoQuant Tag"=w1326) -> ("Error Out"=w1325:errorcluster, "Variant"=w1321:variant)  [unwired: 8 in]
            n417 = Unbundle By Name(w1324) -> ("PQ Hardware Information.Modules.Version Codes"=w1318:i64[])
            n418 = Variant To Data(error in=w1325, type=i64 0 ("PQ Hardware Information.Modules.Type Codes"), Variant=w1321) -> (data=w1319:i64, error out=w1322:errorcluster)
            n419 = Build Array (concatenate)(w1318, w1319) -> (w1320:i64[])
            n420 = Bundle By Name(cluster=w1324, "PQ Hardware Information.Modules.Version Codes"=w1320) -> (w1327:T2)
          }
          frame -1 {
            # "Tag not found"
            n421 = Increment(x=w1334) -> (x+1=w1333:T15)
          }
        }
      }
      frame "HWRouter_Channels" {
        n422 = Format Into String(w1340) -> (resulting string=w1350:string)  [unwired: 3 in, 1 out]
        n423 = Increment(x=w1340) -> (x+1=w1339:T15)
        n424 = Search 1D Array(1D array=w1346, element=w1350) -> (index of element=w1349:i32)  [unwired: 1 in]
        n425 = case shown="0, Default" w1349 {
          selector: w1349 -> [w1360 _]
          tunnel: w1348 -> [w1356 w1368]
          tunnel: [w1359 w1368] -> w1347
          tunnel: w1346 -> [w1364 w1367]
          tunnel: [w1363 w1367] -> w1345
          tunnel: w1344 -> [w1362 w1366]
          tunnel: [w1361 w1366] -> w1343
          tunnel: [w1354 w1365] -> w1342
          tunnel: w1341 -> [w1355 w1365]
          frame 0, Default {
            # "Tag found"
            n426 = Delete From Array(array=w1364, index=w1360) -> (array with subset deleted=w1363:string[])  [unwired: 1 in, 1 out]
            n427 = Delete From Array(array=w1362, index=w1360) -> (deleted portion=w1358:T1, array with subset deleted=w1361:T1[])  [unwired: 1 in]
            n428 = call "Decode Single Tag.vi"("Error In"=w1355, "PicoQuant Tag"=w1358) -> ("Error Out"=w1357:errorcluster, "Variant"=w1353:variant)  [unwired: 8 in]
            n429 = Unbundle By Name(w1356) -> ("PQ Hardware Information.Router Channels.# Router Channels"=w1352:i64)
            n430 = Variant To Data(error in=w1357, type=w1352, Variant=w1353) -> (data=w1351:i64, error out=w1354:errorcluster)
            n431 = Bundle By Name(cluster=w1356, "PQ Hardware Information.Router Channels.# Router Channels"=w1351) -> (w1359:T2)
          }
          frame -1 {
            # "Tag not found"
          }
        }
      }
      frame "HWRouterChan_CFDLevel" {
        n432 = Format Into String(w1370) -> (resulting string=w1380:string)  [unwired: 3 in, 1 out]
        n433 = Search 1D Array(1D array=w1376, element=w1380) -> (index of element=w1379:i32)  [unwired: 1 in]
        n434 = case shown="-1" w1379 {
          selector: w1379 -> [w1393 _]
          tunnel: w1378 -> [w1389 w1403]
          tunnel: [w1392 w1403] -> w1377
          tunnel: w1376 -> [w1397 w1402]
          tunnel: [w1396 w1402] -> w1375
          tunnel: w1374 -> [w1395 w1401]
          tunnel: [w1394 w1401] -> w1373
          tunnel: [w1387 w1400] -> w1372
          tunnel: w1371 -> [w1388 w1400]
          tunnel: w1370 -> [w1381 w1399]
          tunnel: [w1381 w1398] -> w1369
          frame 0, Default {
            # "Tag found"
            n435 = Delete From Array(array=w1397, index=w1393) -> (array with subset deleted=w1396:string[])  [unwired: 1 in, 1 out]
            n436 = Delete From Array(array=w1395, index=w1393) -> (deleted portion=w1391:T1, array with subset deleted=w1394:T1[])  [unwired: 1 in]
            n437 = call "Decode Single Tag.vi"("Error In"=w1388, "PicoQuant Tag"=w1391) -> ("Error Out"=w1390:errorcluster, "Variant"=w1386:variant)  [unwired: 8 in]
            n438 = Unbundle By Name(w1389) -> ("PQ Hardware Information.Router Channels.CFD Levels (mV)"=w1384:i64[])
            n439 = Variant To Data(error in=w1390, type=i64 0 ("PQ Hardware Information.Modules.Type Codes"), Variant=w1386) -> (data=w1385:i64, error out=w1387:errorcluster)
            n440 = Build Array (concatenate)(w1384, w1385) -> (w1382:i64[])
            n441 = Bundle By Name(cluster=w1389, "PQ Hardware Information.Router Channels.CFD Levels (mV)"=w1382) -> (w1392:T2)
          }
          frame -1 {
            # "Tag not found"
            n442 = Increment(x=w1399) -> (x+1=w1398:T15)
          }
        }
      }
      frame "HWRouterChan_CFDPresent" {
        n443 = Format Into String(w1405) -> (resulting string=w1415:string)  [unwired: 3 in, 1 out]
        n444 = Search 1D Array(1D array=w1411, element=w1415) -> (index of element=w1414:i32)  [unwired: 1 in]
        n445 = case shown="-1" w1414 {
          selector: w1414 -> [w1428 _]
          tunnel: w1413 -> [w1424 w1438]
          tunnel: [w1427 w1438] -> w1412
          tunnel: w1411 -> [w1432 w1437]
          tunnel: [w1431 w1437] -> w1410
          tunnel: w1409 -> [w1430 w1436]
          tunnel: [w1429 w1436] -> w1408
          tunnel: [w1422 w1435] -> w1407
          tunnel: w1406 -> [w1423 w1435]
          tunnel: w1405 -> [w1416 w1434]
          tunnel: [w1416 w1433] -> w1404
          frame 0, Default {
            # "Tag found"
            n446 = Delete From Array(array=w1432, index=w1428) -> (array with subset deleted=w1431:string[])  [unwired: 1 in, 1 out]
            n447 = Delete From Array(array=w1430, index=w1428) -> (deleted portion=w1426:T1, array with subset deleted=w1429:T1[])  [unwired: 1 in]
            n448 = call "Decode Single Tag.vi"("Error In"=w1423, "PicoQuant Tag"=w1426) -> ("Error Out"=w1425:errorcluster, "Variant"=w1421:variant)  [unwired: 8 in]
            n449 = Unbundle By Name(w1424) -> ("PQ Hardware Information.Router Channels.CFD Present"=w1419:bool[])
            n450 = Variant To Data(error in=w1425, type=FALSE, Variant=w1421) -> (data=w1420:bool, error out=w1422:errorcluster)
            n451 = Build Array (concatenate)(w1419, w1420) -> (w1417:bool[])
            n452 = Bundle By Name(cluster=w1424, "PQ Hardware Information.Router Channels.CFD Present"=w1417) -> (w1427:T2)
          }
          frame -1 {
            # "Tag not found"
            n453 = Increment(x=w1434) -> (x+1=w1433:T15)
          }
        }
      }
      frame "HWRouterChan_CFDZeroCross" {
        n454 = Format Into String(w1440) -> (resulting string=w1450:string)  [unwired: 3 in, 1 out]
        n455 = Search 1D Array(1D array=w1446, element=w1450) -> (index of element=w1449:i32)  [unwired: 1 in]
        n456 = case shown="-1" w1449 {
          selector: w1449 -> [w1463 _]
          tunnel: w1448 -> [w1459 w1473]
          tunnel: [w1462 w1473] -> w1447
          tunnel: w1446 -> [w1467 w1472]
          tunnel: [w1466 w1472] -> w1445
          tunnel: w1444 -> [w1465 w1471]
          tunnel: [w1464 w1471] -> w1443
          tunnel: [w1457 w1470] -> w1442
          tunnel: w1441 -> [w1458 w1470]
          tunnel: w1440 -> [w1451 w1469]
          tunnel: [w1451 w1468] -> w1439
          frame 0, Default {
            # "Tag found"
            n457 = Delete From Array(array=w1467, index=w1463) -> (array with subset deleted=w1466:string[])  [unwired: 1 in, 1 out]
            n458 = Delete From Array(array=w1465, index=w1463) -> (deleted portion=w1461:T1, array with subset deleted=w1464:T1[])  [unwired: 1 in]
            n459 = Unbundle By Name(w1459) -> ("PQ Hardware Information.Router Channels.CFD Zero Crossings (mV)"=w1454:i64[])
            n460 = call "Decode Single Tag.vi"("Error In"=w1458, "PicoQuant Tag"=w1461) -> ("Error Out"=w1460:errorcluster, "Variant"=w1456:variant)  [unwired: 8 in]
            n461 = Variant To Data(error in=w1460, type=i64 0 ("PQ Hardware Information.Router Channels.CFD Zero Crossings (mV)"), Variant=w1456) -> (data=w1455:i64, error out=w1457:errorcluster)
            n462 = Build Array (concatenate)(w1454, w1455) -> (w1453:i64[])
            n463 = Bundle By Name(cluster=w1459, "PQ Hardware Information.Router Channels.CFD Zero Crossings (mV)"=w1453) -> (w1462:T2)
          }
          frame -1 {
            # "Tag not found"
            n464 = Increment(x=w1469) -> (x+1=w1468:T15)
          }
        }
      }
      frame "HWRouterChan_InputLevel" {
        n465 = Format Into String(w1475) -> (resulting string=w1485:string)  [unwired: 3 in, 1 out]
        n466 = Search 1D Array(1D array=w1481, element=w1485) -> (index of element=w1484:i32)  [unwired: 1 in]
        n467 = case shown="-1" w1484 {
          selector: w1484 -> [w1498 _]
          tunnel: w1483 -> [w1494 w1508]
          tunnel: [w1497 w1508] -> w1482
          tunnel: w1481 -> [w1502 w1507]
          tunnel: [w1501 w1507] -> w1480
          tunnel: w1479 -> [w1500 w1506]
          tunnel: [w1499 w1506] -> w1478
          tunnel: [w1492 w1505] -> w1477
          tunnel: w1476 -> [w1493 w1505]
          tunnel: w1475 -> [w1486 w1504]
          tunnel: [w1486 w1503] -> w1474
          frame 0, Default {
            # "Tag found"
            n468 = Delete From Array(array=w1502, index=w1498) -> (array with subset deleted=w1501:string[])  [unwired: 1 in, 1 out]
            n469 = Delete From Array(array=w1500, index=w1498) -> (deleted portion=w1496:T1, array with subset deleted=w1499:T1[])  [unwired: 1 in]
            n470 = call "Decode Single Tag.vi"("Error In"=w1493, "PicoQuant Tag"=w1496) -> ("Error Out"=w1495:errorcluster, "Variant"=w1491:variant)  [unwired: 8 in]
            n471 = Unbundle By Name(w1494) -> ("PQ Hardware Information.Router Channels.Input Levels (mV)"=w1489:i64[])
            n472 = Variant To Data(error in=w1495, type=i64 0 ("PQ Hardware Information.Router Channels.CFD Zero Crossings (mV)"), Variant=w1491) -> (data=w1490:i64, error out=w1492:errorcluster)
            n473 = Build Array (concatenate)(w1489, w1490) -> (w1488:i64[])
            n474 = Bundle By Name(cluster=w1494, "PQ Hardware Information.Router Channels.Input Levels (mV)"=w1488) -> (w1497:T2)
          }
          frame -1 {
            # "Tag not found"
            n475 = Increment(x=w1504) -> (x+1=w1503:T15)
          }
        }
      }
      frame "HWRouterChan_InputType" {
        n476 = Format Into String(w1510) -> (resulting string=w1520:string)  [unwired: 3 in, 1 out]
        n477 = Search 1D Array(1D array=w1516, element=w1520) -> (index of element=w1519:i32)  [unwired: 1 in]
        n478 = case shown="-1" w1519 {
          selector: w1519 -> [w1533 _]
          tunnel: w1518 -> [w1529 w1543]
          tunnel: [w1532 w1543] -> w1517
          tunnel: w1516 -> [w1537 w1542]
          tunnel: [w1536 w1542] -> w1515
          tunnel: w1514 -> [w1535 w1541]
          tunnel: [w1534 w1541] -> w1513
          tunnel: [w1527 w1540] -> w1512
          tunnel: w1511 -> [w1528 w1540]
          tunnel: w1510 -> [w1521 w1539]
          tunnel: [w1521 w1538] -> w1509
          frame 0, Default {
            # "Tag found"
            n479 = Delete From Array(array=w1537, index=w1533) -> (array with subset deleted=w1536:string[])  [unwired: 1 in, 1 out]
            n480 = Delete From Array(array=w1535, index=w1533) -> (deleted portion=w1531:T1, array with subset deleted=w1534:T1[])  [unwired: 1 in]
            n481 = call "Decode Single Tag.vi"("Error In"=w1528, "PicoQuant Tag"=w1531) -> ("Error Out"=w1530:errorcluster, "Variant"=w1526:variant)  [unwired: 8 in]
            n482 = Unbundle By Name(w1529) -> ("PQ Hardware Information.Router Channels.Input Types"=w1524:i64[])
            n483 = Variant To Data(error in=w1530, type=i64 0 ("PQ Hardware Information.Router Channels.CFD Zero Crossings (mV)"), Variant=w1526) -> (data=w1525:i64, error out=w1527:errorcluster)
            n484 = Build Array (concatenate)(w1524, w1525) -> (w1523:i64[])
            n485 = Bundle By Name(cluster=w1529, "PQ Hardware Information.Router Channels.Input Types"=w1523) -> (w1532:T2)
          }
          frame -1 {
            # "Tag not found"
            n486 = Increment(x=w1539) -> (x+1=w1538:T15)
          }
        }
      }
      frame "HWRouterChan_Offset" {
        n487 = Format Into String(w1545) -> (resulting string=w1555:string)  [unwired: 3 in, 1 out]
        n488 = Search 1D Array(1D array=w1551, element=w1555) -> (index of element=w1554:i32)  [unwired: 1 in]
        n489 = case shown="-1" w1554 {
          selector: w1554 -> [w1568 _]
          tunnel: w1553 -> [w1564 w1578]
          tunnel: [w1567 w1578] -> w1552
          tunnel: w1551 -> [w1572 w1577]
          tunnel: [w1571 w1577] -> w1550
          tunnel: w1549 -> [w1570 w1576]
          tunnel: [w1569 w1576] -> w1548
          tunnel: [w1562 w1575] -> w1547
          tunnel: w1546 -> [w1563 w1575]
          tunnel: w1545 -> [w1556 w1574]
          tunnel: [w1556 w1573] -> w1544
          frame 0, Default {
            # "Tag found"
            n490 = Delete From Array(array=w1572, index=w1568) -> (array with subset deleted=w1571:string[])  [unwired: 1 in, 1 out]
            n491 = Delete From Array(array=w1570, index=w1568) -> (deleted portion=w1566:T1, array with subset deleted=w1569:T1[])  [unwired: 1 in]
            n492 = call "Decode Single Tag.vi"("Error In"=w1563, "PicoQuant Tag"=w1566) -> ("Error Out"=w1565:errorcluster, "Variant"=w1561:variant)  [unwired: 8 in]
            n493 = Unbundle By Name(w1564) -> ("PQ Hardware Information.Router Channels.Offsets (ps)"=w1559:i64[])
            n494 = Variant To Data(error in=w1565, type=i64 0 ("PQ Hardware Information.Router Channels.CFD Zero Crossings (mV)"), Variant=w1561) -> (data=w1560:i64, error out=w1562:errorcluster)
            n495 = Build Array (concatenate)(w1559, w1560) -> (w1558:i64[])
            n496 = Bundle By Name(cluster=w1564, "PQ Hardware Information.Router Channels.Offsets (ps)"=w1558) -> (w1567:T2)
          }
          frame -1 {
            # "Tag not found"
            n497 = Increment(x=w1574) -> (x+1=w1573:T15)
          }
        }
      }
      frame "HWRouterChan_RisingEdge" {
        n498 = Format Into String(w1580) -> (resulting string=w1590:string)  [unwired: 3 in, 1 out]
        n499 = Search 1D Array(1D array=w1586, element=w1590) -> (index of element=w1589:i32)  [unwired: 1 in]
        n500 = case shown="-1" w1589 {
          selector: w1589 -> [w1603 _]
          tunnel: w1588 -> [w1599 w1613]
          tunnel: [w1602 w1613] -> w1587
          tunnel: w1586 -> [w1607 w1612]
          tunnel: [w1606 w1612] -> w1585
          tunnel: w1584 -> [w1605 w1611]
          tunnel: [w1604 w1611] -> w1583
          tunnel: [w1597 w1610] -> w1582
          tunnel: w1581 -> [w1598 w1610]
          tunnel: w1580 -> [w1591 w1609]
          tunnel: [w1591 w1608] -> w1579
          frame 0, Default {
            # "Tag found"
            n501 = Delete From Array(array=w1607, index=w1603) -> (array with subset deleted=w1606:string[])  [unwired: 1 in, 1 out]
            n502 = Delete From Array(array=w1605, index=w1603) -> (deleted portion=w1601:T1, array with subset deleted=w1604:T1[])  [unwired: 1 in]
            n503 = call "Decode Single Tag.vi"("Error In"=w1598, "PicoQuant Tag"=w1601) -> ("Error Out"=w1600:errorcluster, "Variant"=w1596:variant)  [unwired: 8 in]
            n504 = Unbundle By Name(w1599) -> ("PQ Hardware Information.Router Channels.Rising Edges"=w1594:bool[])
            n505 = Variant To Data(error in=w1600, type=FALSE, Variant=w1596) -> (data=w1595:bool, error out=w1597:errorcluster)
            n506 = Build Array (concatenate)(w1594, w1595) -> (w1593:bool[])
            n507 = Bundle By Name(cluster=w1599, "PQ Hardware Information.Router Channels.Rising Edges"=w1593) -> (w1602:T2)
          }
          frame -1 {
            # "Tag not found"
            n508 = Increment(x=w1609) -> (x+1=w1608:T15)
          }
        }
      }
      frame "HWRouter_Enabled" {
        n509 = Format Into String(w1615) -> (resulting string=w1625:string)  [unwired: 3 in, 1 out]
        n510 = Increment(x=w1615) -> (x+1=w1614:T15)
        n511 = Search 1D Array(1D array=w1621, element=w1625) -> (index of element=w1624:i32)  [unwired: 1 in]
        n512 = case shown="0, Default" w1624 {
          selector: w1624 -> [w1635 _]
          tunnel: w1623 -> [w1631 w1643]
          tunnel: [w1634 w1643] -> w1622
          tunnel: w1621 -> [w1639 w1642]
          tunnel: [w1638 w1642] -> w1620
          tunnel: w1619 -> [w1637 w1641]
          tunnel: [w1636 w1641] -> w1618
          tunnel: [w1629 w1640] -> w1617
          tunnel: w1616 -> [w1630 w1640]
          frame 0, Default {
            # "Tag found"
            n513 = Delete From Array(array=w1639, index=w1635) -> (array with subset deleted=w1638:string[])  [unwired: 1 in, 1 out]
            n514 = Delete From Array(array=w1637, index=w1635) -> (deleted portion=w1633:T1, array with subset deleted=w1636:T1[])  [unwired: 1 in]
            n515 = call "Decode Single Tag.vi"("Error In"=w1630, "PicoQuant Tag"=w1633) -> ("Error Out"=w1632:errorcluster, "Variant"=w1628:variant)  [unwired: 8 in]
            n516 = Unbundle By Name(w1631) -> ("PQ Hardware Information.Router Channels.Router Enabled"=w1627:bool)
            n517 = Variant To Data(error in=w1632, type=w1627, Variant=w1628) -> (data=w1626:bool, error out=w1629:errorcluster)
            n518 = Bundle By Name(cluster=w1631, "PQ Hardware Information.Router Channels.Router Enabled"=w1626) -> (w1634:T2)
          }
          frame -1 {
            # "Tag not found"
          }
        }
      }
      frame "HWRouter_ModelCode" {
        n519 = Format Into String(w1645) -> (resulting string=w1655:string)  [unwired: 3 in, 1 out]
        n520 = Increment(x=w1645) -> (x+1=w1644:T15)
        n521 = Search 1D Array(1D array=w1651, element=w1655) -> (index of element=w1654:i32)  [unwired: 1 in]
        n522 = case shown="0, Default" w1654 {
          selector: w1654 -> [w1665 _]
          tunnel: w1653 -> [w1661 w1673]
          tunnel: [w1664 w1673] -> w1652
          tunnel: w1651 -> [w1669 w1672]
          tunnel: [w1668 w1672] -> w1650
          tunnel: w1649 -> [w1667 w1671]
          tunnel: [w1666 w1671] -> w1648
          tunnel: [w1659 w1670] -> w1647
          tunnel: w1646 -> [w1660 w1670]
          frame 0, Default {
            # "Tag found"
            n523 = Delete From Array(array=w1669, index=w1665) -> (array with subset deleted=w1668:string[])  [unwired: 1 in, 1 out]
            n524 = Delete From Array(array=w1667, index=w1665) -> (deleted portion=w1663:T1, array with subset deleted=w1666:T1[])  [unwired: 1 in]
            n525 = call "Decode Single Tag.vi"("Error In"=w1660, "PicoQuant Tag"=w1663) -> ("Error Out"=w1662:errorcluster, "Variant"=w1658:variant)  [unwired: 8 in]
            n526 = Unbundle By Name(w1661) -> ("PQ Hardware Information.Router Channels.Router Model Code"=w1657:i64)
            n527 = Variant To Data(error in=w1662, type=w1657, Variant=w1658) -> (data=w1656:i64, error out=w1659:errorcluster)
            n528 = Bundle By Name(cluster=w1661, "PQ Hardware Information.Router Channels.Router Model Code"=w1656) -> (w1664:T2)
          }
          frame -1 {
            # "Tag not found"
          }
        }
      }
      frame "HWRouter_Version" {
        n529 = Format Into String(w1675) -> (resulting string=w1685:string)  [unwired: 3 in, 1 out]
        n530 = Increment(x=w1675) -> (x+1=w1674:T15)
        n531 = Search 1D Array(1D array=w1681, element=w1685) -> (index of element=w1684:i32)  [unwired: 1 in]
        n532 = case shown="0, Default" w1684 {
          selector: w1684 -> [w1695 _]
          tunnel: w1683 -> [w1691 w1703]
          tunnel: [w1694 w1703] -> w1682
          tunnel: w1681 -> [w1699 w1702]
          tunnel: [w1698 w1702] -> w1680
          tunnel: w1679 -> [w1697 w1701]
          tunnel: [w1696 w1701] -> w1678
          tunnel: [w1689 w1700] -> w1677
          tunnel: w1676 -> [w1690 w1700]
          frame 0, Default {
            # "Tag found"
            n533 = Delete From Array(array=w1699, index=w1695) -> (array with subset deleted=w1698:string[])  [unwired: 1 in, 1 out]
            n534 = Delete From Array(array=w1697, index=w1695) -> (deleted portion=w1693:T1, array with subset deleted=w1696:T1[])  [unwired: 1 in]
            n535 = call "Decode Single Tag.vi"("Error In"=w1690, "PicoQuant Tag"=w1693) -> ("Error Out"=w1692:errorcluster, "Variant"=w1688:variant)  [unwired: 8 in]
            n536 = Unbundle By Name(w1691) -> ("PQ Hardware Information.Router Channels.Router Version"=w1687:string)
            n537 = Variant To Data(error in=w1692, type=w1687, Variant=w1688) -> (data=w1686:string, error out=w1689:errorcluster)
            n538 = Bundle By Name(cluster=w1691, "PQ Hardware Information.Router Channels.Router Version"=w1686) -> (w1694:T2)
          }
          frame -1 {
            # "Tag not found"
          }
        }
      }
      frame "HWSync_CFDLevel" {
        n539 = Format Into String(w1705) -> (resulting string=w1715:string)  [unwired: 3 in, 1 out]
        n540 = Increment(x=w1705) -> (x+1=w1704:T15)
        n541 = Search 1D Array(1D array=w1711, element=w1715) -> (index of element=w1714:i32)  [unwired: 1 in]
        n542 = case shown="0, Default" w1714 {
          selector: w1714 -> [w1725 _]
          tunnel: w1713 -> [w1721 w1733]
          tunnel: [w1724 w1733] -> w1712
          tunnel: w1711 -> [w1729 w1732]
          tunnel: [w1728 w1732] -> w1710
          tunnel: w1709 -> [w1727 w1731]
          tunnel: [w1726 w1731] -> w1708
          tunnel: [w1719 w1730] -> w1707
          tunnel: w1706 -> [w1720 w1730]
          frame 0, Default {
            # "Tag found"
            n543 = Delete From Array(array=w1729, index=w1725) -> (array with subset deleted=w1728:string[])  [unwired: 1 in, 1 out]
            n544 = Delete From Array(array=w1727, index=w1725) -> (deleted portion=w1723:T1, array with subset deleted=w1726:T1[])  [unwired: 1 in]
            n545 = call "Decode Single Tag.vi"("Error In"=w1720, "PicoQuant Tag"=w1723) -> ("Error Out"=w1722:errorcluster, "Variant"=w1718:variant)  [unwired: 8 in]
            n546 = Unbundle By Name(w1721) -> ("PQ Hardware Information.Router Channels.Sync CFD Level (mV)"=w1717:i64)
            n547 = Variant To Data(error in=w1722, type=w1717, Variant=w1718) -> (data=w1716:i64, error out=w1719:errorcluster)
            n548 = Bundle By Name(cluster=w1721, "PQ Hardware Information.Router Channels.Sync CFD Level (mV)"=w1716) -> (w1724:T2)
          }
          frame -1 {
            # "Tag not found"
          }
        }
      }
      frame "HWSync_CFDZeroCross" {
        n549 = Format Into String(w1735) -> (resulting string=w1745:string)  [unwired: 3 in, 1 out]
        n550 = Increment(x=w1735) -> (x+1=w1734:T15)
        n551 = Search 1D Array(1D array=w1741, element=w1745) -> (index of element=w1744:i32)  [unwired: 1 in]
        n552 = case shown="0, Default" w1744 {
          selector: w1744 -> [w1755 _]
          tunnel: w1743 -> [w1751 w1763]
          tunnel: [w1754 w1763] -> w1742
          tunnel: w1741 -> [w1759 w1762]
          tunnel: [w1758 w1762] -> w1740
          tunnel: w1739 -> [w1757 w1761]
          tunnel: [w1756 w1761] -> w1738
          tunnel: [w1749 w1760] -> w1737
          tunnel: w1736 -> [w1750 w1760]
          frame 0, Default {
            # "Tag found"
            n553 = Delete From Array(array=w1759, index=w1755) -> (array with subset deleted=w1758:string[])  [unwired: 1 in, 1 out]
            n554 = Delete From Array(array=w1757, index=w1755) -> (deleted portion=w1753:T1, array with subset deleted=w1756:T1[])  [unwired: 1 in]
            n555 = Unbundle By Name(w1751) -> ("PQ Hardware Information.Router Channels.Sync CFD Zero Crossing (mV)"=w1747:i64)
            n556 = call "Decode Single Tag.vi"("Error In"=w1750, "PicoQuant Tag"=w1753) -> ("Error Out"=w1752:errorcluster, "Variant"=w1748:variant)  [unwired: 8 in]
            n557 = Variant To Data(error in=w1752, type=w1747, Variant=w1748) -> (data=w1746:i64, error out=w1749:errorcluster)
            n558 = Bundle By Name(cluster=w1751, "PQ Hardware Information.Router Channels.Sync CFD Zero Crossing (mV)"=w1746) -> (w1754:T2)
          }
          frame -1 {
            # "Tag not found"
          }
        }
      }
      frame "HWSync_Divider" {
        n559 = Format Into String(w1765) -> (resulting string=w1775:string)  [unwired: 3 in, 1 out]
        n560 = Increment(x=w1765) -> (x+1=w1764:T15)
        n561 = Search 1D Array(1D array=w1771, element=w1775) -> (index of element=w1774:i32)  [unwired: 1 in]
        n562 = case shown="0, Default" w1774 {
          selector: w1774 -> [w1785 _]
          tunnel: w1773 -> [w1781 w1793]
          tunnel: [w1784 w1793] -> w1772
          tunnel: w1771 -> [w1789 w1792]
          tunnel: [w1788 w1792] -> w1770
          tunnel: w1769 -> [w1787 w1791]
          tunnel: [w1786 w1791] -> w1768
          tunnel: [w1779 w1790] -> w1767
          tunnel: w1766 -> [w1780 w1790]
          frame 0, Default {
            # "Tag found"
            n563 = Delete From Array(array=w1789, index=w1785) -> (array with subset deleted=w1788:string[])  [unwired: 1 in, 1 out]
            n564 = Delete From Array(array=w1787, index=w1785) -> (deleted portion=w1783:T1, array with subset deleted=w1786:T1[])  [unwired: 1 in]
            n565 = call "Decode Single Tag.vi"("Error In"=w1780, "PicoQuant Tag"=w1783) -> ("Error Out"=w1782:errorcluster, "Variant"=w1778:variant)  [unwired: 8 in]
            n566 = Unbundle By Name(w1781) -> ("PQ Hardware Information.Router Channels.Sync Divider"=w1777:i64)
            n567 = Variant To Data(error in=w1782, type=w1777, Variant=w1778) -> (data=w1776:i64, error out=w1779:errorcluster)
            n568 = Bundle By Name(cluster=w1781, "PQ Hardware Information.Router Channels.Sync Divider"=w1776) -> (w1784:T2)
          }
          frame -1 {
            # "Tag not found"
          }
        }
      }
      frame "HWSync_Offset" {
        n569 = Format Into String(w1795) -> (resulting string=w1805:string)  [unwired: 3 in, 1 out]
        n570 = Increment(x=w1795) -> (x+1=w1794:T15)
        n571 = Search 1D Array(1D array=w1801, element=w1805) -> (index of element=w1804:i32)  [unwired: 1 in]
        n572 = case shown="0, Default" w1804 {
          selector: w1804 -> [w1815 _]
          tunnel: w1803 -> [w1811 w1823]
          tunnel: [w1814 w1823] -> w1802
          tunnel: w1801 -> [w1819 w1822]
          tunnel: [w1818 w1822] -> w1800
          tunnel: w1799 -> [w1817 w1821]
          tunnel: [w1816 w1821] -> w1798
          tunnel: [w1809 w1820] -> w1797
          tunnel: w1796 -> [w1810 w1820]
          frame 0, Default {
            # "Tag found"
            n573 = Delete From Array(array=w1819, index=w1815) -> (array with subset deleted=w1818:string[])  [unwired: 1 in, 1 out]
            n574 = Delete From Array(array=w1817, index=w1815) -> (deleted portion=w1813:T1, array with subset deleted=w1816:T1[])  [unwired: 1 in]
            n575 = call "Decode Single Tag.vi"("Error In"=w1810, "PicoQuant Tag"=w1813) -> ("Error Out"=w1812:errorcluster, "Variant"=w1808:variant)  [unwired: 8 in]
            n576 = Unbundle By Name(w1811) -> ("PQ Hardware Information.Router Channels.Sync Offset (ps)"=w1807:i64)
            n577 = Variant To Data(error in=w1812, type=w1807, Variant=w1808) -> (data=w1806:i64, error out=w1809:errorcluster)
            n578 = Bundle By Name(cluster=w1811, "PQ Hardware Information.Router Channels.Sync Offset (ps)"=w1806) -> (w1814:T2)
          }
          frame -1 {
            # "Tag not found"
          }
        }
      }
      frame "HWSync_TrgEdge" {
        n579 = Format Into String(w1825) -> (resulting string=w1835:string)  [unwired: 3 in, 1 out]
        n580 = Increment(x=w1825) -> (x+1=w1824:T15)
        n581 = Search 1D Array(1D array=w1831, element=w1835) -> (index of element=w1834:i32)  [unwired: 1 in]
        n582 = case shown="0, Default" w1834 {
          selector: w1834 -> [w1845 _]
          tunnel: w1833 -> [w1841 w1853]
          tunnel: [w1844 w1853] -> w1832
          tunnel: w1831 -> [w1849 w1852]
          tunnel: [w1848 w1852] -> w1830
          tunnel: w1829 -> [w1847 w1851]
          tunnel: [w1846 w1851] -> w1828
          tunnel: [w1839 w1850] -> w1827
          tunnel: w1826 -> [w1840 w1850]
          frame 0, Default {
            # "Tag found"
            n583 = Delete From Array(array=w1849, index=w1845) -> (array with subset deleted=w1848:string[])  [unwired: 1 in, 1 out]
            n584 = Delete From Array(array=w1847, index=w1845) -> (deleted portion=w1843:T1, array with subset deleted=w1846:T1[])  [unwired: 1 in]
            n585 = call "Decode Single Tag.vi"("Error In"=w1840, "PicoQuant Tag"=w1843) -> ("Error Out"=w1842:errorcluster, "Variant"=w1838:variant)  [unwired: 8 in]
            n586 = Unbundle By Name(w1841) -> ("PQ Hardware Information.Router Channels.Sync Trigger Edge"=w1837:i64)
            n587 = Variant To Data(error in=w1842, type=w1837, Variant=w1838) -> (data=w1836:i64, error out=w1839:errorcluster)
            n588 = Bundle By Name(cluster=w1841, "PQ Hardware Information.Router Channels.Sync Trigger Edge"=w1836) -> (w1844:T2)
          }
          frame -1 {
            # "Tag not found"
          }
        }
      }
      frame "HWSync_TrgLevel" {
        n589 = Format Into String(w1855) -> (resulting string=w1865:string)  [unwired: 3 in, 1 out]
        n590 = Increment(x=w1855) -> (x+1=w1854:T15)
        n591 = Search 1D Array(1D array=w1861, element=w1865) -> (index of element=w1864:i32)  [unwired: 1 in]
        n592 = case shown="0, Default" w1864 {
          selector: w1864 -> [w1875 _]
          tunnel: w1863 -> [w1871 w1883]
          tunnel: [w1874 w1883] -> w1862
          tunnel: w1861 -> [w1879 w1882]
          tunnel: [w1878 w1882] -> w1860
          tunnel: w1859 -> [w1877 w1881]
          tunnel: [w1876 w1881] -> w1858
          tunnel: [w1869 w1880] -> w1857
          tunnel: w1856 -> [w1870 w1880]
          frame 0, Default {
            # "Tag found"
            n593 = Delete From Array(array=w1879, index=w1875) -> (array with subset deleted=w1878:string[])  [unwired: 1 in, 1 out]
            n594 = Delete From Array(array=w1877, index=w1875) -> (deleted portion=w1873:T1, array with subset deleted=w1876:T1[])  [unwired: 1 in]
            n595 = Unbundle By Name(w1871) -> ("PQ Hardware Information.Router Channels.Sync Trigger Level (mV)"=w1867:i64)
            n596 = call "Decode Single Tag.vi"("Error In"=w1870, "PicoQuant Tag"=w1873) -> ("Error Out"=w1872:errorcluster, "Variant"=w1868:variant)  [unwired: 8 in]
            n597 = Variant To Data(error in=w1872, type=w1867, Variant=w1868) -> (data=w1866:i64, error out=w1869:errorcluster)
            n598 = Bundle By Name(cluster=w1871, "PQ Hardware Information.Router Channels.Sync Trigger Level (mV)"=w1866) -> (w1874:T2)
          }
          frame -1 {
            # "Tag not found"
          }
        }
      }
      frame "HWTriggerOut_On" {
        n599 = Format Into String(w1885) -> (resulting string=w1895:string)  [unwired: 3 in, 1 out]
        n600 = Increment(x=w1885) -> (x+1=w1884:T15)
        n601 = Search 1D Array(1D array=w1891, element=w1895) -> (index of element=w1894:i32)  [unwired: 1 in]
        n602 = case shown="0, Default" w1894 {
          selector: w1894 -> [w1905 _]
          tunnel: w1893 -> [w1901 w1913]
          tunnel: [w1904 w1913] -> w1892
          tunnel: w1891 -> [w1909 w1912]
          tunnel: [w1908 w1912] -> w1890
          tunnel: w1889 -> [w1907 w1911]
          tunnel: [w1906 w1911] -> w1888
          tunnel: [w1899 w1910] -> w1887
          tunnel: w1886 -> [w1900 w1910]
          frame 0, Default {
            # "Tag found"
            n603 = Delete From Array(array=w1909, index=w1905) -> (array with subset deleted=w1908:string[])  [unwired: 1 in, 1 out]
            n604 = Delete From Array(array=w1907, index=w1905) -> (deleted portion=w1903:T1, array with subset deleted=w1906:T1[])  [unwired: 1 in]
            n605 = call "Decode Single Tag.vi"("Error In"=w1900, "PicoQuant Tag"=w1903) -> ("Error Out"=w1902:errorcluster, "Variant"=w1898:variant)  [unwired: 8 in]
            n606 = Unbundle By Name(w1901) -> ("PQ Hardware Information.Router Channels.Trigger Out On"=w1897:bool)
            n607 = Variant To Data(error in=w1902, type=w1897, Variant=w1898) -> (data=w1896:bool, error out=w1899:errorcluster)
            n608 = Bundle By Name(cluster=w1901, "PQ Hardware Information.Router Channels.Trigger Out On"=w1896) -> (w1904:T2)
          }
          frame -1 {
            # "Tag not found"
          }
        }
      }
      frame "HWTriggerOut_Period" {
        n609 = Format Into String(w1915) -> (resulting string=w1925:string)  [unwired: 3 in, 1 out]
        n610 = Increment(x=w1915) -> (x+1=w1914:T15)
        n611 = Search 1D Array(1D array=w1921, element=w1925) -> (index of element=w1924:i32)  [unwired: 1 in]
        n612 = case shown="0, Default" w1924 {
          selector: w1924 -> [w1935 _]
          tunnel: w1923 -> [w1931 w1943]
          tunnel: [w1934 w1943] -> w1922
          tunnel: w1921 -> [w1939 w1942]
          tunnel: [w1938 w1942] -> w1920
          tunnel: w1919 -> [w1937 w1941]
          tunnel: [w1936 w1941] -> w1918
          tunnel: [w1929 w1940] -> w1917
          tunnel: w1916 -> [w1930 w1940]
          frame 0, Default {
            # "Tag found"
            n613 = Delete From Array(array=w1939, index=w1935) -> (array with subset deleted=w1938:string[])  [unwired: 1 in, 1 out]
            n614 = Delete From Array(array=w1937, index=w1935) -> (deleted portion=w1933:T1, array with subset deleted=w1936:T1[])  [unwired: 1 in]
            n615 = call "Decode Single Tag.vi"("Error In"=w1930, "PicoQuant Tag"=w1933) -> ("Error Out"=w1932:errorcluster, "Variant"=w1928:variant)  [unwired: 8 in]
            n616 = Unbundle By Name(w1931) -> ("PQ Hardware Information.Router Channels.Trigger Out Period (s)"=w1927:dbl)
            n617 = Variant To Data(error in=w1932, type=w1927, Variant=w1928) -> (data=w1926:dbl, error out=w1929:errorcluster)
            n618 = Bundle By Name(cluster=w1931, "PQ Hardware Information.Router Channels.Trigger Out Period (s)"=w1926) -> (w1934:T2)
          }
          frame -1 {
            # "Tag not found"
          }
        }
      }
      frame "HW_BaseResolution" {
        n619 = Format Into String(w1945) -> (resulting string=w1955:string)  [unwired: 3 in, 1 out]
        n620 = Increment(x=w1945) -> (x+1=w1944:T15)
        n621 = Search 1D Array(1D array=w1951, element=w1955) -> (index of element=w1954:i32)  [unwired: 1 in]
        n622 = case shown="0, Default" w1954 {
          selector: w1954 -> [w1965 _]
          tunnel: w1953 -> [w1961 w1973]
          tunnel: [w1964 w1973] -> w1952
          tunnel: w1951 -> [w1969 w1972]
          tunnel: [w1968 w1972] -> w1950
          tunnel: w1949 -> [w1967 w1971]
          tunnel: [w1966 w1971] -> w1948
          tunnel: [w1959 w1970] -> w1947
          tunnel: w1946 -> [w1960 w1970]
          frame 0, Default {
            # "Tag found"
            n623 = Delete From Array(array=w1969, index=w1965) -> (array with subset deleted=w1968:string[])  [unwired: 1 in, 1 out]
            n624 = Delete From Array(array=w1967, index=w1965) -> (deleted portion=w1963:T1, array with subset deleted=w1966:T1[])  [unwired: 1 in]
            n625 = call "Decode Single Tag.vi"("Error In"=w1960, "PicoQuant Tag"=w1963) -> ("Error Out"=w1962:errorcluster, "Variant"=w1958:variant)  [unwired: 8 in]
            n626 = Unbundle By Name(w1961) -> ("PQ Hardware Information.Router Channels.Base Resolution (s)"=w1957:dbl)
            n627 = Variant To Data(error in=w1962, type=w1957, Variant=w1958) -> (data=w1956:dbl, error out=w1959:errorcluster)
            n628 = Bundle By Name(cluster=w1961, "PQ Hardware Information.Router Channels.Base Resolution (s)"=w1956) -> (w1964:T2)
          }
          frame -1 {
            # "Tag not found"
          }
        }
      }
      frame "HW_ExternalDevices" {
        n629 = Format Into String(w1975) -> (resulting string=w1985:string)  [unwired: 3 in, 1 out]
        n630 = Increment(x=w1975) -> (x+1=w1974:T15)
        n631 = Search 1D Array(1D array=w1981, element=w1985) -> (index of element=w1984:i32)  [unwired: 1 in]
        n632 = case shown="0, Default" w1984 {
          selector: w1984 -> [w1995 _]
          tunnel: w1983 -> [w1991 w2003]
          tunnel: [w1994 w2003] -> w1982
          tunnel: w1981 -> [w1999 w2002]
          tunnel: [w1998 w2002] -> w1980
          tunnel: w1979 -> [w1997 w2001]
          tunnel: [w1996 w2001] -> w1978
          tunnel: [w1989 w2000] -> w1977
          tunnel: w1976 -> [w1990 w2000]
          frame 0, Default {
            # "Tag found"
            n633 = Delete From Array(array=w1999, index=w1995) -> (array with subset deleted=w1998:string[])  [unwired: 1 in, 1 out]
            n634 = Delete From Array(array=w1997, index=w1995) -> (deleted portion=w1993:T1, array with subset deleted=w1996:T1[])  [unwired: 1 in]
            n635 = call "Decode Single Tag.vi"("Error In"=w1990, "PicoQuant Tag"=w1993) -> ("Error Out"=w1992:errorcluster, "Variant"=w1988:variant)  [unwired: 8 in]
            n636 = Unbundle By Name(w1991) -> ("PQ Hardware Information.Router Channels.External Devices"=w1987:i64)
            n637 = Variant To Data(error in=w1992, type=w1987, Variant=w1988) -> (data=w1986:i64, error out=w1989:errorcluster)
            n638 = Bundle By Name(cluster=w1991, "PQ Hardware Information.Router Channels.External Devices"=w1986) -> (w1994:T2)
          }
          frame -1 {
            # "Tag not found"
          }
        }
      }
      frame "HW_ExternalRefClock" {
        n639 = Format Into String(w2005) -> (resulting string=w2015:string)  [unwired: 3 in, 1 out]
        n640 = Increment(x=w2005) -> (x+1=w2004:T15)
        n641 = Search 1D Array(1D array=w2011, element=w2015) -> (index of element=w2014:i32)  [unwired: 1 in]
        n642 = case shown="0, Default" w2014 {
          selector: w2014 -> [w2025 _]
          tunnel: w2013 -> [w2021 w2033]
          tunnel: [w2024 w2033] -> w2012
          tunnel: w2011 -> [w2029 w2032]
          tunnel: [w2028 w2032] -> w2010
          tunnel: w2009 -> [w2027 w2031]
          tunnel: [w2026 w2031] -> w2008
          tunnel: [w2019 w2030] -> w2007
          tunnel: w2006 -> [w2020 w2030]
          frame 0, Default {
            # "Tag found"
            n643 = Delete From Array(array=w2029, index=w2025) -> (array with subset deleted=w2028:string[])  [unwired: 1 in, 1 out]
            n644 = Delete From Array(array=w2027, index=w2025) -> (deleted portion=w2023:T1, array with subset deleted=w2026:T1[])  [unwired: 1 in]
            n645 = Unbundle By Name(w2021) -> ("PQ Hardware Information.Router Channels.External Reference Clock"=w2017:bool)
            n646 = call "Decode Single Tag.vi"("Error In"=w2020, "PicoQuant Tag"=w2023) -> ("Error Out"=w2022:errorcluster, "Variant"=w2018:variant)  [unwired: 8 in]
            n647 = Variant To Data(error in=w2022, type=w2017, Variant=w2018) -> (data=w2016:bool, error out=w2019:errorcluster)
            n648 = Bundle By Name(cluster=w2021, "PQ Hardware Information.Router Channels.External Reference Clock"=w2016) -> (w2024:T2)
          }
          frame -1 {
            # "Tag not found"
          }
        }
      }
      frame "HW_Features" {
        n649 = Format Into String(w2035) -> (resulting string=w2045:string)  [unwired: 3 in, 1 out]
        n650 = Increment(x=w2035) -> (x+1=w2034:T15)
        n651 = Search 1D Array(1D array=w2041, element=w2045) -> (index of element=w2044:i32)  [unwired: 1 in]
        n652 = case shown="0, Default" w2044 {
          selector: w2044 -> [w2055 _]
          tunnel: w2043 -> [w2051 w2063]
          tunnel: [w2054 w2063] -> w2042
          tunnel: w2041 -> [w2059 w2062]
          tunnel: [w2058 w2062] -> w2040
          tunnel: w2039 -> [w2057 w2061]
          tunnel: [w2056 w2061] -> w2038
          tunnel: [w2049 w2060] -> w2037
          tunnel: w2036 -> [w2050 w2060]
          frame 0, Default {
            # "Tag found"
            n653 = Delete From Array(array=w2059, index=w2055) -> (array with subset deleted=w2058:string[])  [unwired: 1 in, 1 out]
            n654 = Delete From Array(array=w2057, index=w2055) -> (deleted portion=w2053:T1, array with subset deleted=w2056:T1[])  [unwired: 1 in]
            n655 = call "Decode Single Tag.vi"("Error In"=w2050, "PicoQuant Tag"=w2053) -> ("Error Out"=w2052:errorcluster, "Variant"=w2048:variant)  [unwired: 8 in]
            n656 = Unbundle By Name(w2051) -> ("PQ Hardware Information.Router Channels.Features"=w2047:u64)
            n657 = Variant To Data(error in=w2052, type=w2047, Variant=w2048) -> (data=w2046:u64, error out=w2049:errorcluster)
            n658 = Bundle By Name(cluster=w2051, "PQ Hardware Information.Router Channels.Features"=w2046) -> (w2054:T2)
          }
          frame -1 {
            # "Tag not found"
          }
        }
      }
      frame "HW_PartNo" {
        n659 = Format Into String(w2065) -> (resulting string=w2075:string)  [unwired: 3 in, 1 out]
        n660 = Increment(x=w2065) -> (x+1=w2064:T15)
        n661 = Search 1D Array(1D array=w2071, element=w2075) -> (index of element=w2074:i32)  [unwired: 1 in]
        n662 = case shown="0, Default" w2074 {
          selector: w2074 -> [w2085 _]
          tunnel: w2073 -> [w2081 w2093]
          tunnel: [w2084 w2093] -> w2072
          tunnel: w2071 -> [w2089 w2092]
          tunnel: [w2088 w2092] -> w2070
          tunnel: w2069 -> [w2087 w2091]
          tunnel: [w2086 w2091] -> w2068
          tunnel: [w2079 w2090] -> w2067
          tunnel: w2066 -> [w2080 w2090]
          frame 0, Default {
            # "Tag found"
            n663 = Delete From Array(array=w2089, index=w2085) -> (array with subset deleted=w2088:string[])  [unwired: 1 in, 1 out]
            n664 = Delete From Array(array=w2087, index=w2085) -> (deleted portion=w2083:T1, array with subset deleted=w2086:T1[])  [unwired: 1 in]
            n665 = call "Decode Single Tag.vi"("Error In"=w2080, "PicoQuant Tag"=w2083) -> ("Error Out"=w2082:errorcluster, "Variant"=w2078:variant)  [unwired: 8 in]
            n666 = Unbundle By Name(w2081) -> ("PQ Hardware Information.Router Channels.Part Number"=w2077:string)
            n667 = Variant To Data(error in=w2082, type=w2077, Variant=w2078) -> (data=w2076:string, error out=w2079:errorcluster)
            n668 = Bundle By Name(cluster=w2081, "PQ Hardware Information.Router Channels.Part Number"=w2076) -> (w2084:T2)
          }
          frame -1 {
            # "Tag not found"
          }
        }
      }
      frame "HW_RoutingChannels" {
        # "obsolete for V >= 1.0.00"
        n669 = Format Into String(w2095) -> (resulting string=w2100:string)  [unwired: 3 in, 1 out]
        n670 = Search 1D Array(1D array=w2098, element=w2100) -> ()  [unwired: 1 in, 1 out]
        n671 = Increment(x=w2095) -> (x+1=w2094:T15)
      }
      frame "HW_SerialNo" {
        n672 = Format Into String(w2102) -> (resulting string=w2112:string)  [unwired: 3 in, 1 out]
        n673 = Increment(x=w2102) -> (x+1=w2101:T15)
        n674 = Search 1D Array(1D array=w2108, element=w2112) -> (index of element=w2111:i32)  [unwired: 1 in]
        n675 = case shown="0, Default" w2111 {
          selector: w2111 -> [w2124 _]
          tunnel: w2110 -> [w2121 w2143]
          tunnel: [w2123 w2143] -> w2109
          tunnel: w2108 -> [w2128 w2142]
          tunnel: [w2127 w2142] -> w2107
          tunnel: w2106 -> [w2126 w2141]
          tunnel: [w2125 w2141] -> w2105
          tunnel: [w2113 w2140] -> w2104
          tunnel: w2103 -> [w2120 w2140]
          frame 0, Default {
            # "Tag found"
            n676 = Unbundle By Name(w2121) -> ("PQ Hardware Information.Router Channels.Serial Number (string)"=w2119:string, "PQ Hardware Information.Router Channels.Serial Number"=w2114:i64)
            n677 = Delete From Array(array=w2128, index=w2124) -> (array with subset deleted=w2127:string[])  [unwired: 1 in, 1 out]
            n678 = Delete From Array(array=w2126, index=w2124) -> (deleted portion=w2122:T1, array with subset deleted=w2125:T1[])  [unwired: 1 in]
            n679 = call "Decode Single Tag.vi"("Error In"=w2120, "PicoQuant Tag"=w2122) -> ("Error Out"=w2116:errorcluster, "Variant"=w2115:variant)  [unwired: 8 in]
            n680 = Variant To Data(error in=w2116, type=w2119, Variant=w2115) -> (data=w2118:string, error out=w2117:errorcluster)
            n681 = case shown="No Error" w2117 {
              selector: w2117 -> [w2129 _]
              tunnel: [w2132 w2136] -> w2123
              tunnel: w2121 -> [w2131 w2137]
              tunnel: w2118 -> [w2130 _]
              tunnel: w2116 -> [_ w2139]
              tunnel: w2115 -> [_ w2138]
              tunnel: w2114 -> [_ w2135]
              tunnel: [w2129 w2133] -> w2113
              frame No Error {
                n682 = Bundle By Name(cluster=w2131, "PQ Hardware Information.Router Channels.Serial Number (string)"=w2130) -> (w2132:T2)
              }
              frame Error {
                n683 = Variant To Data(error in=w2139, type=w2135, Variant=w2138) -> (data=w2134:i64, error out=w2133:errorcluster)
                n684 = Bundle By Name(cluster=w2137, "PQ Hardware Information.Router Channels.Serial Number"=w2134) -> (w2136:T2)
              }
            }
          }
          frame -1 {
            # "Tag not found"
          }
        }
      }
      frame "HW_Timingmode" {
        n685 = Format Into String(w2145) -> (resulting string=w2155:string)  [unwired: 3 in, 1 out]
        n686 = Increment(x=w2145) -> (x+1=w2144:T15)
        n687 = Search 1D Array(1D array=w2151, element=w2155) -> (index of element=w2154:i32)  [unwired: 1 in]
        n688 = case shown="0, Default" w2154 {
          selector: w2154 -> [w2165 _]
          tunnel: w2153 -> [w2161 w2173]
          tunnel: [w2164 w2173] -> w2152
          tunnel: w2151 -> [w2169 w2172]
          tunnel: [w2168 w2172] -> w2150
          tunnel: w2149 -> [w2167 w2171]
          tunnel: [w2166 w2171] -> w2148
          tunnel: [w2159 w2170] -> w2147
          tunnel: w2146 -> [w2160 w2170]
          frame 0, Default {
            # "Tag found"
            n689 = Delete From Array(array=w2169, index=w2165) -> (array with subset deleted=w2168:string[])  [unwired: 1 in, 1 out]
            n690 = Delete From Array(array=w2167, index=w2165) -> (deleted portion=w2163:T1, array with subset deleted=w2166:T1[])  [unwired: 1 in]
            n691 = call "Decode Single Tag.vi"("Error In"=w2160, "PicoQuant Tag"=w2163) -> ("Error Out"=w2162:errorcluster, "Variant"=w2158:variant)  [unwired: 8 in]
            n692 = Unbundle By Name(w2161) -> ("PQ Hardware Information.Router Channels.Timing Mode"=w2157:i64)
            n693 = Variant To Data(error in=w2162, type=w2157, Variant=w2158) -> (data=w2156:i64, error out=w2159:errorcluster)
            n694 = Bundle By Name(cluster=w2161, "PQ Hardware Information.Router Channels.Timing Mode"=w2156) -> (w2164:T2)
          }
          frame -1 {
            # "Tag not found"
          }
        }
      }
      frame "HW_Type" {
        n695 = Format Into String(w2175) -> (resulting string=w2185:string)  [unwired: 3 in, 1 out]
        n696 = Increment(x=w2175) -> (x+1=w2174:T15)
        n697 = Search 1D Array(1D array=w2181, element=w2185) -> (index of element=w2184:i32)  [unwired: 1 in]
        n698 = case shown="0, Default" w2184 {
          selector: w2184 -> [w2195 _]
          tunnel: w2183 -> [w2191 w2203]
          tunnel: [w2194 w2203] -> w2182
          tunnel: w2181 -> [w2199 w2202]
          tunnel: [w2198 w2202] -> w2180
          tunnel: w2179 -> [w2197 w2201]
          tunnel: [w2196 w2201] -> w2178
          tunnel: [w2189 w2200] -> w2177
          tunnel: w2176 -> [w2190 w2200]
          frame 0, Default {
            # "Tag found"
            n699 = Delete From Array(array=w2199, index=w2195) -> (array with subset deleted=w2198:string[])  [unwired: 1 in, 1 out]
            n700 = Delete From Array(array=w2197, index=w2195) -> (deleted portion=w2193:T1, array with subset deleted=w2196:T1[])  [unwired: 1 in]
            n701 = call "Decode Single Tag.vi"("Error In"=w2190, "PicoQuant Tag"=w2193) -> ("Error Out"=w2192:errorcluster, "Variant"=w2188:variant)  [unwired: 8 in]
            n702 = Unbundle By Name(w2191) -> ("PQ Hardware Information.Router Channels.Hardware Type"=w2187:string)
            n703 = Variant To Data(error in=w2192, type=w2187, Variant=w2188) -> (data=w2186:string, error out=w2189:errorcluster)
            n704 = Bundle By Name(cluster=w2191, "PQ Hardware Information.Router Channels.Hardware Type"=w2186) -> (w2194:T2)
          }
          frame -1 {
            # "Tag not found"
          }
        }
      }
      frame "HW_Version" {
        n705 = Format Into String(w2205) -> (resulting string=w2215:string)  [unwired: 3 in, 1 out]
        n706 = Increment(x=w2205) -> (x+1=w2204:T15)
        n707 = Search 1D Array(1D array=w2211, element=w2215) -> (index of element=w2214:i32)  [unwired: 1 in]
        n708 = case shown="0, Default" w2214 {
          selector: w2214 -> [w2225 _]
          tunnel: w2213 -> [w2221 w2233]
          tunnel: [w2224 w2233] -> w2212
          tunnel: w2211 -> [w2229 w2232]
          tunnel: [w2228 w2232] -> w2210
          tunnel: w2209 -> [w2227 w2231]
          tunnel: [w2226 w2231] -> w2208
          tunnel: [w2219 w2230] -> w2207
          tunnel: w2206 -> [w2220 w2230]
          frame 0, Default {
            # "Tag found"
            n709 = Delete From Array(array=w2229, index=w2225) -> (array with subset deleted=w2228:string[])  [unwired: 1 in, 1 out]
            n710 = Delete From Array(array=w2227, index=w2225) -> (deleted portion=w2223:T1, array with subset deleted=w2226:T1[])  [unwired: 1 in]
            n711 = call "Decode Single Tag.vi"("Error In"=w2220, "PicoQuant Tag"=w2223) -> ("Error Out"=w2222:errorcluster, "Variant"=w2218:variant)  [unwired: 8 in]
            n712 = Unbundle By Name(w2221) -> ("PQ Hardware Information.Router Channels.Hardware Type"=w2217:string)
            n713 = Variant To Data(error in=w2222, type=w2217, Variant=w2218) -> (data=w2216:string, error out=w2219:errorcluster)
            n714 = Bundle By Name(cluster=w2221, "PQ Hardware Information.Router Channels.Hardware Type"=w2216) -> (w2224:T2)
          }
          frame -1 {
            # "Tag not found"
          }
        }
      }
      frame "<Measurement Description>" {
        n715 = Increment(x=w2235) -> (x+1=w2234:T15)
      }
      frame "MeasDesc_AcquisitionTime" {
        n716 = Format Into String(w2241) -> (resulting string=w2251:string)  [unwired: 3 in, 1 out]
        n717 = Increment(x=w2241) -> (x+1=w2240:T15)
        n718 = Search 1D Array(1D array=w2247, element=w2251) -> (index of element=w2250:i32)  [unwired: 1 in]
        n719 = case shown="0, Default" w2250 {
          selector: w2250 -> [w2261 _]
          tunnel: w2249 -> [w2257 w2269]
          tunnel: [w2260 w2269] -> w2248
          tunnel: w2247 -> [w2265 w2268]
          tunnel: [w2264 w2268] -> w2246
          tunnel: w2245 -> [w2263 w2267]
          tunnel: [w2262 w2267] -> w2244
          tunnel: [w2255 w2266] -> w2243
          tunnel: w2242 -> [w2256 w2266]
          frame 0, Default {
            # "Tag found"
            n720 = Delete From Array(array=w2265, index=w2261) -> (array with subset deleted=w2264:string[])  [unwired: 1 in, 1 out]
            n721 = Delete From Array(array=w2263, index=w2261) -> (deleted portion=w2259:T1, array with subset deleted=w2262:T1[])  [unwired: 1 in]
            n722 = call "Decode Single Tag.vi"("Error In"=w2256, "PicoQuant Tag"=w2259) -> ("Error Out"=w2258:errorcluster, "Variant"=w2254:variant)  [unwired: 8 in]
            n723 = Unbundle By Name(w2257) -> ("PQ Measurement Information.Acquisition Time (ms)"=w2253:i64)
            n724 = Variant To Data(error in=w2258, type=w2253, Variant=w2254) -> (data=w2252:i64, error out=w2255:errorcluster)
            n725 = Bundle By Name(cluster=w2257, "PQ Measurement Information.Acquisition Time (ms)"=w2252) -> (w2260:T2)
          }
          frame -1 {
            # "Tag not found"
          }
        }
      }
      frame "MeasDesc_BinningFactor" {
        n726 = Format Into String(w2271) -> (resulting string=w2281:string)  [unwired: 3 in, 1 out]
        n727 = Increment(x=w2271) -> (x+1=w2270:T15)
        n728 = Search 1D Array(1D array=w2277, element=w2281) -> (index of element=w2280:i32)  [unwired: 1 in]
        n729 = case shown="0, Default" w2280 {
          selector: w2280 -> [w2291 _]
          tunnel: w2279 -> [w2287 w2299]
          tunnel: [w2290 w2299] -> w2278
          tunnel: w2277 -> [w2295 w2298]
          tunnel: [w2294 w2298] -> w2276
          tunnel: w2275 -> [w2293 w2297]
          tunnel: [w2292 w2297] -> w2274
          tunnel: [w2285 w2296] -> w2273
          tunnel: w2272 -> [w2286 w2296]
          frame 0, Default {
            # "Tag found"
            n730 = Delete From Array(array=w2295, index=w2291) -> (array with subset deleted=w2294:string[])  [unwired: 1 in, 1 out]
            n731 = Delete From Array(array=w2293, index=w2291) -> (deleted portion=w2289:T1, array with subset deleted=w2292:T1[])  [unwired: 1 in]
            n732 = call "Decode Single Tag.vi"("Error In"=w2286, "PicoQuant Tag"=w2289) -> ("Error Out"=w2288:errorcluster, "Variant"=w2284:variant)  [unwired: 8 in]
            n733 = Unbundle By Name(w2287) -> ("PQ Measurement Information.Binning Factor"=w2283:i64)
            n734 = Variant To Data(error in=w2288, type=w2283, Variant=w2284) -> (data=w2282:i64, error out=w2285:errorcluster)
            n735 = Bundle By Name(cluster=w2287, "PQ Measurement Information.Binning Factor"=w2282) -> (w2290:T2)
          }
          frame -1 {
            # "Tag not found"
          }
        }
      }
      frame "MeasDesc_GlobalResolution" {
        n736 = Format Into String(w2301) -> (resulting string=w2311:string)  [unwired: 3 in, 1 out]
        n737 = Increment(x=w2301) -> (x+1=w2300:T15)
        n738 = Search 1D Array(1D array=w2307, element=w2311) -> (index of element=w2310:i32)  [unwired: 1 in]
        n739 = case shown="0, Default" w2310 {
          selector: w2310 -> [w2321 _]
          tunnel: w2309 -> [w2317 w2329]
          tunnel: [w2320 w2329] -> w2308
          tunnel: w2307 -> [w2325 w2328]
          tunnel: [w2324 w2328] -> w2306
          tunnel: w2305 -> [w2323 w2327]
          tunnel: [w2322 w2327] -> w2304
          tunnel: [w2315 w2326] -> w2303
          tunnel: w2302 -> [w2316 w2326]
          frame 0, Default {
            # "Tag found"
            n740 = Delete From Array(array=w2325, index=w2321) -> (array with subset deleted=w2324:string[])  [unwired: 1 in, 1 out]
            n741 = Delete From Array(array=w2323, index=w2321) -> (deleted portion=w2319:T1, array with subset deleted=w2322:T1[])  [unwired: 1 in]
            n742 = call "Decode Single Tag.vi"("Error In"=w2316, "PicoQuant Tag"=w2319) -> ("Error Out"=w2318:errorcluster, "Variant"=w2314:variant)  [unwired: 8 in]
            n743 = Unbundle By Name(w2317) -> ("PQ Measurement Information.Global Resolution (s)"=w2313:dbl)
            n744 = Variant To Data(error in=w2318, type=w2313, Variant=w2314) -> (data=w2312:dbl, error out=w2315:errorcluster)
            n745 = Bundle By Name(cluster=w2317, "PQ Measurement Information.Global Resolution (s)"=w2312) -> (w2320:T2)
          }
          frame -1 {
            # "Tag not found"
          }
        }
      }
      frame "MeasDesc_InvalidSync" {
        n746 = Format Into String(w2331) -> (resulting string=w2341:string)  [unwired: 3 in, 1 out]
        n747 = Increment(x=w2331) -> (x+1=w2330:T15)
        n748 = Search 1D Array(1D array=w2337, element=w2341) -> (index of element=w2340:i32)  [unwired: 1 in]
        n749 = case shown="0, Default" w2340 {
          selector: w2340 -> [w2351 _]
          tunnel: w2339 -> [w2347 w2359]
          tunnel: [w2350 w2359] -> w2338
          tunnel: w2337 -> [w2355 w2358]
          tunnel: [w2354 w2358] -> w2336
          tunnel: w2335 -> [w2353 w2357]
          tunnel: [w2352 w2357] -> w2334
          tunnel: [w2345 w2356] -> w2333
          tunnel: w2332 -> [w2346 w2356]
          frame 0, Default {
            # "Tag found"
            n750 = Delete From Array(array=w2355, index=w2351) -> (array with subset deleted=w2354:string[])  [unwired: 1 in, 1 out]
            n751 = Delete From Array(array=w2353, index=w2351) -> (deleted portion=w2349:T1, array with subset deleted=w2352:T1[])  [unwired: 1 in]
            n752 = call "Decode Single Tag.vi"("Error In"=w2346, "PicoQuant Tag"=w2349) -> ("Error Out"=w2348:errorcluster, "Variant"=w2344:variant)  [unwired: 8 in]
            n753 = Unbundle By Name(w2347) -> ("PQ Measurement Information.Invalid Sync"=w2343:bool)
            n754 = Variant To Data(error in=w2348, type=w2343, Variant=w2344) -> (data=w2342:bool, error out=w2345:errorcluster)
            n755 = Bundle By Name(cluster=w2347, "PQ Measurement Information.Invalid Sync"=w2342) -> (w2350:T2)
          }
          frame -1 {
            # "Tag not found"
          }
        }
      }
      frame "MeasDesc_Offset" {
        n756 = Format Into String(w2361) -> (resulting string=w2371:string)  [unwired: 3 in, 1 out]
        n757 = Increment(x=w2361) -> (x+1=w2360:T15)
        n758 = Search 1D Array(1D array=w2367, element=w2371) -> (index of element=w2370:i32)  [unwired: 1 in]
        n759 = case shown="0, Default" w2370 {
          selector: w2370 -> [w2381 _]
          tunnel: w2369 -> [w2377 w2389]
          tunnel: [w2380 w2389] -> w2368
          tunnel: w2367 -> [w2385 w2388]
          tunnel: [w2384 w2388] -> w2366
          tunnel: w2365 -> [w2383 w2387]
          tunnel: [w2382 w2387] -> w2364
          tunnel: [w2375 w2386] -> w2363
          tunnel: w2362 -> [w2376 w2386]
          frame 0, Default {
            # "Tag found"
            n760 = Delete From Array(array=w2385, index=w2381) -> (array with subset deleted=w2384:string[])  [unwired: 1 in, 1 out]
            n761 = Delete From Array(array=w2383, index=w2381) -> (deleted portion=w2379:T1, array with subset deleted=w2382:T1[])  [unwired: 1 in]
            n762 = call "Decode Single Tag.vi"("Error In"=w2376, "PicoQuant Tag"=w2379) -> ("Error Out"=w2378:errorcluster, "Variant"=w2374:variant)  [unwired: 8 in]
            n763 = Unbundle By Name(w2377) -> ("PQ Measurement Information.Offset (ns)"=w2373:u64)
            n764 = Variant To Data(error in=w2378, type=w2373, Variant=w2374) -> (data=w2372:u64, error out=w2375:errorcluster)
            n765 = Bundle By Name(cluster=w2377, "PQ Measurement Information.Offset (ns)"=w2372) -> (w2380:T2)
          }
          frame -1 {
            # "Tag not found"
          }
        }
      }
      frame "MeasDesc_Params" {
        n766 = Format Into String(w2391) -> (resulting string=w2401:string)  [unwired: 3 in, 1 out]
        n767 = Search 1D Array(1D array=w2397, element=w2401) -> (index of element=w2400:i32)  [unwired: 1 in]
        n768 = Increment(x=w2391) -> (x+1=w2390:T15)
        n769 = case shown="0, Default" w2400 {
          selector: w2400 -> [w2411 _]
          tunnel: w2399 -> [w2407 w2419]
          tunnel: [w2410 w2419] -> w2398
          tunnel: w2397 -> [w2415 w2418]
          tunnel: [w2414 w2418] -> w2396
          tunnel: w2395 -> [w2413 w2417]
          tunnel: [w2412 w2417] -> w2394
          tunnel: [w2405 w2416] -> w2393
          tunnel: w2392 -> [w2406 w2416]
          frame 0, Default {
            # "Tag found"
            n770 = Delete From Array(array=w2415, index=w2411) -> (array with subset deleted=w2414:string[])  [unwired: 1 in, 1 out]
            n771 = Delete From Array(array=w2413, index=w2411) -> (deleted portion=w2409:T1, array with subset deleted=w2412:T1[])  [unwired: 1 in]
            n772 = call "Decode Single Tag.vi"("Error In"=w2406, "PicoQuant Tag"=w2409) -> ("Error Out"=w2408:errorcluster, "Variant"=w2404:variant)  [unwired: 8 in]
            n773 = Unbundle By Name(w2407) -> ("PQ Measurement Information.# Curve Parameters"=w2403:u64)
            n774 = Variant To Data(error in=w2408, type=w2403, Variant=w2404) -> (data=w2402:u64, error out=w2405:errorcluster)
            n775 = Bundle By Name(cluster=w2407, "PQ Measurement Information.# Curve Parameters"=w2402) -> (w2410:T2)
          }
          frame -1 {
            # "Tag not found"
          }
        }
      }
      frame "MeasDesc_Param_Device" {
        n776 = Format Into String(w2421) -> (resulting string=w2431:string)  [unwired: 3 in, 1 out]
        n777 = Search 1D Array(1D array=w2427, element=w2431) -> (index of element=w2430:i32)  [unwired: 1 in]
        n778 = case shown="-1" w2430 {
          selector: w2430 -> [w2444 _]
          tunnel: w2429 -> [w2440 w2454]
          tunnel: [w2443 w2454] -> w2428
          tunnel: w2427 -> [w2448 w2453]
          tunnel: [w2447 w2453] -> w2426
          tunnel: w2425 -> [w2446 w2452]
          tunnel: [w2445 w2452] -> w2424
          tunnel: [w2438 w2451] -> w2423
          tunnel: w2422 -> [w2439 w2451]
          tunnel: w2421 -> [w2432 w2450]
          tunnel: [w2432 w2449] -> w2420
          frame 0, Default {
            # "Tag found"
            n779 = Delete From Array(array=w2448, index=w2444) -> (array with subset deleted=w2447:string[])  [unwired: 1 in, 1 out]
            n780 = Delete From Array(array=w2446, index=w2444) -> (deleted portion=w2442:T1, array with subset deleted=w2445:T1[])  [unwired: 1 in]
            n781 = call "Decode Single Tag.vi"("Error In"=w2439, "PicoQuant Tag"=w2442) -> ("Error Out"=w2441:errorcluster, "Variant"=w2437:variant)  [unwired: 8 in]
            n782 = Unbundle By Name(w2440) -> ("PQ Measurement Information.Devices"=w2434:string[])
            n783 = Variant To Data(error in=w2441, type="" ("PQ Measurement Information.Devices"), Variant=w2437) -> (data=w2433:string, error out=w2438:errorcluster)
            n784 = Build Array (concatenate)(w2434, w2433) -> (w2436:string[])
            n785 = Bundle By Name(cluster=w2440, "PQ Measurement Information.Devices"=w2436) -> (w2443:T2)
          }
          frame -1 {
            # "Tag not found"
            n786 = Increment(x=w2450) -> (x+1=w2449:T15)
          }
        }
      }
      frame "MeasDesc_Param_Name" {
        n787 = Format Into String(w2456) -> (resulting string=w2466:string)  [unwired: 3 in, 1 out]
        n788 = Search 1D Array(1D array=w2462, element=w2466) -> (index of element=w2465:i32)  [unwired: 1 in]
        n789 = case shown="-1" w2465 {
          selector: w2465 -> [w2479 _]
          tunnel: w2464 -> [w2475 w2489]
          tunnel: [w2478 w2489] -> w2463
          tunnel: w2462 -> [w2483 w2488]
          tunnel: [w2482 w2488] -> w2461
          tunnel: w2460 -> [w2481 w2487]
          tunnel: [w2480 w2487] -> w2459
          tunnel: [w2473 w2486] -> w2458
          tunnel: w2457 -> [w2474 w2486]
          tunnel: w2456 -> [w2467 w2485]
          tunnel: [w2467 w2484] -> w2455
          frame 0, Default {
            # "Tag found"
            n790 = Delete From Array(array=w2483, index=w2479) -> (array with subset deleted=w2482:string[])  [unwired: 1 in, 1 out]
            n791 = Delete From Array(array=w2481, index=w2479) -> (deleted portion=w2477:T1, array with subset deleted=w2480:T1[])  [unwired: 1 in]
            n792 = call "Decode Single Tag.vi"("Error In"=w2474, "PicoQuant Tag"=w2477) -> ("Error Out"=w2476:errorcluster, "Variant"=w2472:variant)  [unwired: 8 in]
            n793 = Unbundle By Name(w2475) -> ("PQ Measurement Information.Names"=w2469:string[])
            n794 = Variant To Data(error in=w2476, type="" ("PQ Measurement Information.Devices"), Variant=w2472) -> (data=w2468:string, error out=w2473:errorcluster)
            n795 = Build Array (concatenate)(w2469, w2468) -> (w2471:string[])
            n796 = Bundle By Name(cluster=w2475, "PQ Measurement Information.Names"=w2471) -> (w2478:T2)
          }
          frame -1 {
            # "Tag not found"
            n797 = Increment(x=w2485) -> (x+1=w2484:T15)
          }
        }
      }
      frame "MeasDesc_Param_Start" {
        n798 = Format Into String(w2491) -> (resulting string=w2501:string)  [unwired: 3 in, 1 out]
        n799 = Search 1D Array(1D array=w2497, element=w2501) -> (index of element=w2500:i32)  [unwired: 1 in]
        n800 = case shown="-1" w2500 {
          selector: w2500 -> [w2514 _]
          tunnel: w2499 -> [w2510 w2524]
          tunnel: [w2513 w2524] -> w2498
          tunnel: w2497 -> [w2518 w2523]
          tunnel: [w2517 w2523] -> w2496
          tunnel: w2495 -> [w2516 w2522]
          tunnel: [w2515 w2522] -> w2494
          tunnel: [w2508 w2521] -> w2493
          tunnel: w2492 -> [w2509 w2521]
          tunnel: w2491 -> [w2502 w2520]
          tunnel: [w2502 w2519] -> w2490
          frame 0, Default {
            # "Tag found"
            n801 = Delete From Array(array=w2518, index=w2514) -> (array with subset deleted=w2517:string[])  [unwired: 1 in, 1 out]
            n802 = Delete From Array(array=w2516, index=w2514) -> (deleted portion=w2512:T1, array with subset deleted=w2515:T1[])  [unwired: 1 in]
            n803 = call "Decode Single Tag.vi"("Error In"=w2509, "PicoQuant Tag"=w2512) -> ("Error Out"=w2511:errorcluster, "Variant"=w2507:variant)  [unwired: 8 in]
            n804 = Unbundle By Name(w2510) -> ("PQ Measurement Information.Start Values"=w2504:dbl[])
            n805 = Variant To Data(error in=w2511, type=0.0 ("PQ Measurement Information.Devices"), Variant=w2507) -> (data=w2503:dbl, error out=w2508:errorcluster)
            n806 = Build Array (concatenate)(w2504, w2503) -> (w2506:dbl[])
            n807 = Bundle By Name(cluster=w2510, "PQ Measurement Information.Start Values"=w2506) -> (w2513:T2)
          }
          frame -1 {
            # "Tag not found"
            n808 = Increment(x=w2520) -> (x+1=w2519:T15)
          }
        }
      }
      frame "MeasDesc_Param_Step" {
        n809 = Format Into String(w2526) -> (resulting string=w2536:string)  [unwired: 3 in, 1 out]
        n810 = Search 1D Array(1D array=w2532, element=w2536) -> (index of element=w2535:i32)  [unwired: 1 in]
        n811 = case shown="-1" w2535 {
          selector: w2535 -> [w2549 _]
          tunnel: w2534 -> [w2545 w2559]
          tunnel: [w2548 w2559] -> w2533
          tunnel: w2532 -> [w2553 w2558]
          tunnel: [w2552 w2558] -> w2531
          tunnel: w2530 -> [w2551 w2557]
          tunnel: [w2550 w2557] -> w2529
          tunnel: [w2543 w2556] -> w2528
          tunnel: w2527 -> [w2544 w2556]
          tunnel: w2526 -> [w2537 w2555]
          tunnel: [w2537 w2554] -> w2525
          frame 0, Default {
            # "Tag found"
            n812 = Delete From Array(array=w2553, index=w2549) -> (array with subset deleted=w2552:string[])  [unwired: 1 in, 1 out]
            n813 = Delete From Array(array=w2551, index=w2549) -> (deleted portion=w2547:T1, array with subset deleted=w2550:T1[])  [unwired: 1 in]
            n814 = call "Decode Single Tag.vi"("Error In"=w2544, "PicoQuant Tag"=w2547) -> ("Error Out"=w2546:errorcluster, "Variant"=w2542:variant)  [unwired: 8 in]
            n815 = Unbundle By Name(w2545) -> ("PQ Measurement Information.Steps"=w2539:dbl[])
            n816 = Variant To Data(error in=w2546, type=0.0 ("PQ Measurement Information.Devices"), Variant=w2542) -> (data=w2538:dbl, error out=w2543:errorcluster)
            n817 = Build Array (concatenate)(w2539, w2538) -> (w2541:dbl[])
            n818 = Bundle By Name(cluster=w2545, "PQ Measurement Information.Steps"=w2541) -> (w2548:T2)
          }
          frame -1 {
            # "Tag not found"
            n819 = Increment(x=w2555) -> (x+1=w2554:T15)
          }
        }
      }
      frame "MeasDesc_Param_Stop" {
        n820 = Format Into String(w2561) -> (resulting string=w2571:string)  [unwired: 3 in, 1 out]
        n821 = Search 1D Array(1D array=w2567, element=w2571) -> (index of element=w2570:i32)  [unwired: 1 in]
        n822 = case shown="-1" w2570 {
          selector: w2570 -> [w2584 _]
          tunnel: w2569 -> [w2580 w2594]
          tunnel: [w2583 w2594] -> w2568
          tunnel: w2567 -> [w2588 w2593]
          tunnel: [w2587 w2593] -> w2566
          tunnel: w2565 -> [w2586 w2592]
          tunnel: [w2585 w2592] -> w2564
          tunnel: [w2578 w2591] -> w2563
          tunnel: w2562 -> [w2579 w2591]
          tunnel: w2561 -> [w2572 w2590]
          tunnel: [w2572 w2589] -> w2560
          frame 0, Default {
            # "Tag found"
            n823 = Delete From Array(array=w2588, index=w2584) -> (array with subset deleted=w2587:string[])  [unwired: 1 in, 1 out]
            n824 = Delete From Array(array=w2586, index=w2584) -> (deleted portion=w2582:T1, array with subset deleted=w2585:T1[])  [unwired: 1 in]
            n825 = call "Decode Single Tag.vi"("Error In"=w2579, "PicoQuant Tag"=w2582) -> ("Error Out"=w2581:errorcluster, "Variant"=w2577:variant)  [unwired: 8 in]
            n826 = Unbundle By Name(w2580) -> ("PQ Measurement Information.Stop Values"=w2574:dbl[])
            n827 = Variant To Data(error in=w2581, type=0.0 ("PQ Measurement Information.Devices"), Variant=w2577) -> (data=w2573:dbl, error out=w2578:errorcluster)
            n828 = Build Array (concatenate)(w2574, w2573) -> (w2576:dbl[])
            n829 = Bundle By Name(cluster=w2580, "PQ Measurement Information.Stop Values"=w2576) -> (w2583:T2)
          }
          frame -1 {
            # "Tag not found"
            n830 = Increment(x=w2590) -> (x+1=w2589:T15)
          }
        }
      }
      frame "MeasDesc_Param_TagName" {
        n831 = Format Into String(w2596) -> (resulting string=w2606:string)  [unwired: 3 in, 1 out]
        n832 = Search 1D Array(1D array=w2602, element=w2606) -> (index of element=w2605:i32)  [unwired: 1 in]
        n833 = case shown="-1" w2605 {
          selector: w2605 -> [w2619 _]
          tunnel: w2604 -> [w2615 w2629]
          tunnel: [w2618 w2629] -> w2603
          tunnel: w2602 -> [w2623 w2628]
          tunnel: [w2622 w2628] -> w2601
          tunnel: w2600 -> [w2621 w2627]
          tunnel: [w2620 w2627] -> w2599
          tunnel: [w2613 w2626] -> w2598
          tunnel: w2597 -> [w2614 w2626]
          tunnel: w2596 -> [w2607 w2625]
          tunnel: [w2607 w2624] -> w2595
          frame 0, Default {
            # "Tag found"
            n834 = Delete From Array(array=w2623, index=w2619) -> (array with subset deleted=w2622:string[])  [unwired: 1 in, 1 out]
            n835 = Delete From Array(array=w2621, index=w2619) -> (deleted portion=w2617:T1, array with subset deleted=w2620:T1[])  [unwired: 1 in]
            n836 = call "Decode Single Tag.vi"("Error In"=w2614, "PicoQuant Tag"=w2617) -> ("Error Out"=w2616:errorcluster, "Variant"=w2612:variant)  [unwired: 8 in]
            n837 = Unbundle By Name(w2615) -> ("PQ Measurement Information.Tag Names"=w2609:string[])
            n838 = Variant To Data(error in=w2616, type="" ("PQ Measurement Information.Devices"), Variant=w2612) -> (data=w2608:string, error out=w2613:errorcluster)
            n839 = Build Array (concatenate)(w2609, w2608) -> (w2611:string[])
            n840 = Bundle By Name(cluster=w2615, "PQ Measurement Information.Tag Names"=w2611) -> (w2618:T2)
          }
          frame -1 {
            # "Tag not found"
            n841 = Increment(x=w2625) -> (x+1=w2624:T15)
          }
        }
      }
      frame "MeasDesc_Param_Unit" {
        n842 = Format Into String(w2631) -> (resulting string=w2641:string)  [unwired: 3 in, 1 out]
        n843 = Search 1D Array(1D array=w2637, element=w2641) -> (index of element=w2640:i32)  [unwired: 1 in]
        n844 = case shown="-1" w2640 {
          selector: w2640 -> [w2654 _]
          tunnel: w2639 -> [w2650 w2664]
          tunnel: [w2653 w2664] -> w2638
          tunnel: w2637 -> [w2658 w2663]
          tunnel: [w2657 w2663] -> w2636
          tunnel: w2635 -> [w2656 w2662]
          tunnel: [w2655 w2662] -> w2634
          tunnel: [w2648 w2661] -> w2633
          tunnel: w2632 -> [w2649 w2661]
          tunnel: w2631 -> [w2642 w2660]
          tunnel: [w2642 w2659] -> w2630
          frame 0, Default {
            # "Tag found"
            n845 = Delete From Array(array=w2658, index=w2654) -> (array with subset deleted=w2657:string[])  [unwired: 1 in, 1 out]
            n846 = Delete From Array(array=w2656, index=w2654) -> (deleted portion=w2652:T1, array with subset deleted=w2655:T1[])  [unwired: 1 in]
            n847 = call "Decode Single Tag.vi"("Error In"=w2649, "PicoQuant Tag"=w2652) -> ("Error Out"=w2651:errorcluster, "Variant"=w2647:variant)  [unwired: 8 in]
            n848 = Unbundle By Name(w2650) -> ("PQ Measurement Information.Units"=w2644:string[])
            n849 = Variant To Data(error in=w2651, type="" ("PQ Measurement Information.Devices"), Variant=w2647) -> (data=w2643:string, error out=w2648:errorcluster)
            n850 = Build Array (concatenate)(w2644, w2643) -> (w2646:string[])
            n851 = Bundle By Name(cluster=w2650, "PQ Measurement Information.Units"=w2646) -> (w2653:T2)
          }
          frame -1 {
            # "Tag not found"
            n852 = Increment(x=w2660) -> (x+1=w2659:T15)
          }
        }
      }
      frame "MeasDesc_Resolution" {
        n853 = Format Into String(w2666) -> (resulting string=w2676:string)  [unwired: 3 in, 1 out]
        n854 = Increment(x=w2666) -> (x+1=w2665:T15)
        n855 = Search 1D Array(1D array=w2672, element=w2676) -> (index of element=w2675:i32)  [unwired: 1 in]
        n856 = case shown="0, Default" w2675 {
          selector: w2675 -> [w2686 _]
          tunnel: w2674 -> [w2682 w2694]
          tunnel: [w2685 w2694] -> w2673
          tunnel: w2672 -> [w2690 w2693]
          tunnel: [w2689 w2693] -> w2671
          tunnel: w2670 -> [w2688 w2692]
          tunnel: [w2687 w2692] -> w2669
          tunnel: [w2680 w2691] -> w2668
          tunnel: w2667 -> [w2681 w2691]
          frame 0, Default {
            # "Tag found"
            n857 = Delete From Array(array=w2690, index=w2686) -> (array with subset deleted=w2689:string[])  [unwired: 1 in, 1 out]
            n858 = Delete From Array(array=w2688, index=w2686) -> (deleted portion=w2684:T1, array with subset deleted=w2687:T1[])  [unwired: 1 in]
            n859 = call "Decode Single Tag.vi"("Error In"=w2681, "PicoQuant Tag"=w2684) -> ("Error Out"=w2683:errorcluster, "Variant"=w2679:variant)  [unwired: 8 in]
            n860 = Unbundle By Name(w2682) -> ("PQ Measurement Information.Resolution (s)"=w2678:dbl)
            n861 = Variant To Data(error in=w2683, type=w2678, Variant=w2679) -> (data=w2677:dbl, error out=w2680:errorcluster)
            n862 = Bundle By Name(cluster=w2682, "PQ Measurement Information.Resolution (s)"=w2677) -> (w2685:T2)
          }
          frame -1 {
            # "Tag not found"
          }
        }
      }
      frame "MeasDesc_Restart" {
        n863 = Format Into String(w2696) -> (resulting string=w2706:string)  [unwired: 3 in, 1 out]
        n864 = Increment(x=w2696) -> (x+1=w2695:T15)
        n865 = Search 1D Array(1D array=w2702, element=w2706) -> (index of element=w2705:i32)  [unwired: 1 in]
        n866 = case shown="0, Default" w2705 {
          selector: w2705 -> [w2716 _]
          tunnel: w2704 -> [w2712 w2724]
          tunnel: [w2715 w2724] -> w2703
          tunnel: w2702 -> [w2720 w2723]
          tunnel: [w2719 w2723] -> w2701
          tunnel: w2700 -> [w2718 w2722]
          tunnel: [w2717 w2722] -> w2699
          tunnel: [w2710 w2721] -> w2698
          tunnel: w2697 -> [w2711 w2721]
          frame 0, Default {
            # "Tag found"
            n867 = Delete From Array(array=w2720, index=w2716) -> (array with subset deleted=w2719:string[])  [unwired: 1 in, 1 out]
            n868 = Delete From Array(array=w2718, index=w2716) -> (deleted portion=w2714:T1, array with subset deleted=w2717:T1[])  [unwired: 1 in]
            n869 = call "Decode Single Tag.vi"("Error In"=w2711, "PicoQuant Tag"=w2714) -> ("Error Out"=w2713:errorcluster, "Variant"=w2709:variant)  [unwired: 8 in]
            n870 = Unbundle By Name(w2712) -> ("PQ Measurement Information.Restart"=w2708:bool)
            n871 = Variant To Data(error in=w2713, type=w2708, Variant=w2709) -> (data=w2707:bool, error out=w2710:errorcluster)
            n872 = Bundle By Name(cluster=w2712, "PQ Measurement Information.Restart"=w2707) -> (w2715:T2)
          }
          frame -1 {
            # "Tag not found"
          }
        }
      }
      frame "MeasDesc_StopAt" {
        n873 = Format Into String(w2726) -> (resulting string=w2736:string)  [unwired: 3 in, 1 out]
        n874 = Increment(x=w2726) -> (x+1=w2725:T15)
        n875 = Search 1D Array(1D array=w2732, element=w2736) -> (index of element=w2735:i32)  [unwired: 1 in]
        n876 = case shown="0, Default" w2735 {
          selector: w2735 -> [w2746 _]
          tunnel: w2734 -> [w2742 w2754]
          tunnel: [w2745 w2754] -> w2733
          tunnel: w2732 -> [w2750 w2753]
          tunnel: [w2749 w2753] -> w2731
          tunnel: w2730 -> [w2748 w2752]
          tunnel: [w2747 w2752] -> w2729
          tunnel: [w2740 w2751] -> w2728
          tunnel: w2727 -> [w2741 w2751]
          frame 0, Default {
            # "Tag found"
            n877 = Delete From Array(array=w2750, index=w2746) -> (array with subset deleted=w2749:string[])  [unwired: 1 in, 1 out]
            n878 = Delete From Array(array=w2748, index=w2746) -> (deleted portion=w2744:T1, array with subset deleted=w2747:T1[])  [unwired: 1 in]
            n879 = call "Decode Single Tag.vi"("Error In"=w2741, "PicoQuant Tag"=w2744) -> ("Error Out"=w2743:errorcluster, "Variant"=w2739:variant)  [unwired: 8 in]
            n880 = Unbundle By Name(w2742) -> ("PQ Measurement Information.Stop At"=w2738:u64)
            n881 = Variant To Data(error in=w2743, type=w2738, Variant=w2739) -> (data=w2737:u64, error out=w2740:errorcluster)
            n882 = Bundle By Name(cluster=w2742, "PQ Measurement Information.Stop At"=w2737) -> (w2745:T2)
          }
          frame -1 {
            # "Tag not found"
          }
        }
      }
      frame "MeasDesc_StopOnOvfl" {
        n883 = Format Into String(w2756) -> (resulting string=w2766:string)  [unwired: 3 in, 1 out]
        n884 = Increment(x=w2756) -> (x+1=w2755:T15)
        n885 = Search 1D Array(1D array=w2762, element=w2766) -> (index of element=w2765:i32)  [unwired: 1 in]
        n886 = case shown="0, Default" w2765 {
          selector: w2765 -> [w2776 _]
          tunnel: w2764 -> [w2772 w2784]
          tunnel: [w2775 w2784] -> w2763
          tunnel: w2762 -> [w2780 w2783]
          tunnel: [w2779 w2783] -> w2761
          tunnel: w2760 -> [w2778 w2782]
          tunnel: [w2777 w2782] -> w2759
          tunnel: [w2770 w2781] -> w2758
          tunnel: w2757 -> [w2771 w2781]
          frame 0, Default {
            # "Tag found"
            n887 = Delete From Array(array=w2780, index=w2776) -> (array with subset deleted=w2779:string[])  [unwired: 1 in, 1 out]
            n888 = Delete From Array(array=w2778, index=w2776) -> (deleted portion=w2774:T1, array with subset deleted=w2777:T1[])  [unwired: 1 in]
            n889 = call "Decode Single Tag.vi"("Error In"=w2771, "PicoQuant Tag"=w2774) -> ("Error Out"=w2773:errorcluster, "Variant"=w2769:variant)  [unwired: 8 in]
            n890 = Unbundle By Name(w2772) -> ("PQ Measurement Information.Stop on Over f1"=w2768:bool)
            n891 = Variant To Data(error in=w2773, type=w2768, Variant=w2769) -> (data=w2767:bool, error out=w2770:errorcluster)
            n892 = Bundle By Name(cluster=w2772, "PQ Measurement Information.Stop on Over f1"=w2767) -> (w2775:T2)
          }
          frame -1 {
            # "Tag not found"
          }
        }
      }
      frame "<Image Header>" {
        n893 = Increment(x=w2786) -> (x+1=w2785:T15)
      }
      frame "ImgHdr_Acceleration" {
        n894 = Format Into String(w2792) -> (resulting string=w2802:string)  [unwired: 3 in, 1 out]
        n895 = Increment(x=w2792) -> (x+1=w2791:T15)
        n896 = Search 1D Array(1D array=w2798, element=w2802) -> (index of element=w2801:i32)  [unwired: 1 in]
        n897 = case shown="0, Default" w2801 {
          selector: w2801 -> [w2812 _]
          tunnel: w2800 -> [w2808 w2820]
          tunnel: [w2811 w2820] -> w2799
          tunnel: w2798 -> [w2816 w2819]
          tunnel: [w2815 w2819] -> w2797
          tunnel: w2796 -> [w2814 w2818]
          tunnel: [w2813 w2818] -> w2795
          tunnel: [w2806 w2817] -> w2794
          tunnel: w2793 -> [w2807 w2817]
          frame 0, Default {
            # "Tag found"
            n898 = Delete From Array(array=w2816, index=w2812) -> (array with subset deleted=w2815:string[])  [unwired: 1 in, 1 out]
            n899 = Delete From Array(array=w2814, index=w2812) -> (deleted portion=w2810:T1, array with subset deleted=w2813:T1[])  [unwired: 1 in]
            n900 = Unbundle By Name(w2808) -> ("PQ Image Information.Hardware Acceleration"=w2804:i64)
            n901 = call "Decode Single Tag.vi"("Error In"=w2807, "PicoQuant Tag"=w2810) -> ("Error Out"=w2809:errorcluster, "Variant"=w2805:variant)  [unwired: 8 in]
            n902 = Variant To Data(error in=w2809, type=w2804, Variant=w2805) -> (data=w2803:i64, error out=w2806:errorcluster)
            n903 = Bundle By Name(cluster=w2808, "PQ Image Information.Hardware Acceleration"=w2803) -> (w2811:T2)
          }
          frame -1 {
            # "Tag not found"
          }
        }
      }
      frame "ImgHdr_BiDirect" {
        n904 = Format Into String(w2822) -> (resulting string=w2832:string)  [unwired: 3 in, 1 out]
        n905 = Increment(x=w2822) -> (x+1=w2821:T15)
        n906 = Search 1D Array(1D array=w2828, element=w2832) -> (index of element=w2831:i32)  [unwired: 1 in]
        n907 = case shown="0, Default" w2831 {
          selector: w2831 -> [w2844 _]
          tunnel: w2830 -> [w2842 w2858]
          tunnel: [w2843 w2858] -> w2829
          tunnel: w2828 -> [w2848 w2857]
          tunnel: [w2847 w2857] -> w2827
          tunnel: w2826 -> [w2846 w2856]
          tunnel: [w2845 w2856] -> w2825
          tunnel: [w2837 w2855] -> w2824
          tunnel: w2823 -> [w2841 w2855]
          frame 0, Default {
            # "Tag found"
            n908 = Delete From Array(array=w2848, index=w2844) -> (array with subset deleted=w2847:string[])  [unwired: 1 in, 1 out]
            n909 = Delete From Array(array=w2846, index=w2844) -> (deleted portion=w2834:T1, array with subset deleted=w2845:T1[])  [unwired: 1 in]
            n910 = call "Decode Single Tag.vi"("Error In"=w2841, "PicoQuant Tag"=w2834) -> ("Error Out"=w2833:errorcluster, "Variant"=w2840:variant)  [unwired: 8 in]
            n911 = Unbundle By Name(w2842) -> ("PQ Image Information.Bidirectional"=w2839:bool)
            n912 = Variant To Data(error in=w2833, type=w2839, Variant=w2840) -> (data=w2836:bool, error out=w2838:errorcluster)
            n913 = case shown="Error .." w2838 {
              selector: w2838 -> [w2850 _]
              tunnel: [w2850 w2851] -> w2837
              tunnel: w2836 -> [w2849 _]
              tunnel: [w2849 w2852] -> w2835
              tunnel: w2834 -> [_ w2854]
              tunnel: w2833 -> [_ w2853]
              frame No Error {
              }
              frame Error {
                n914 = call "Decode BiDirectional Tag (Erroneous Type).vi"("error in (no error)"=w2853, "PicoQuant Tag"=w2854) -> ("error out"=w2851:errorcluster, "Bidirectional"=w2852:bool)  [unwired: 8 in]
              }
            }
            n915 = Bundle By Name(cluster=w2842, "PQ Image Information.Bidirectional"=w2835) -> (w2843:T2)
          }
          frame -1 {
            # "Tag not found"
          }
        }
      }
      frame "ImgHdr_Dimensions" {
        n916 = Format Into String(w2860) -> (resulting string=w2870:string)  [unwired: 3 in, 1 out]
        n917 = Increment(x=w2860) -> (x+1=w2859:T15)
        n918 = Search 1D Array(1D array=w2866, element=w2870) -> (index of element=w2869:i32)  [unwired: 1 in]
        n919 = case shown="0, Default" w2869 {
          selector: w2869 -> [w2880 _]
          tunnel: w2868 -> [w2876 w2888]
          tunnel: [w2879 w2888] -> w2867
          tunnel: w2866 -> [w2884 w2887]
          tunnel: [w2883 w2887] -> w2865
          tunnel: w2864 -> [w2882 w2886]
          tunnel: [w2881 w2886] -> w2863
          tunnel: [w2874 w2885] -> w2862
          tunnel: w2861 -> [w2875 w2885]
          frame 0, Default {
            # "Tag found"
            n920 = Delete From Array(array=w2884, index=w2880) -> (array with subset deleted=w2883:string[])  [unwired: 1 in, 1 out]
            n921 = Delete From Array(array=w2882, index=w2880) -> (deleted portion=w2878:T1, array with subset deleted=w2881:T1[])  [unwired: 1 in]
            n922 = call "Decode Single Tag.vi"("Error In"=w2875, "PicoQuant Tag"=w2878) -> ("Error Out"=w2877:errorcluster, "Variant"=w2873:variant)  [unwired: 8 in]
            n923 = Unbundle By Name(w2876) -> ("PQ Image Information.Dimensions"=w2872:i64)
            n924 = Variant To Data(error in=w2877, type=w2872, Variant=w2873) -> (data=w2871:i64, error out=w2874:errorcluster)
            n925 = Bundle By Name(cluster=w2876, "PQ Image Information.Dimensions"=w2871) -> (w2879:T2)
          }
          frame -1 {
            # "Tag not found"
          }
        }
      }
      frame "ImgHdr_Frame" {
        n926 = Format Into String(w2890) -> (resulting string=w2900:string)  [unwired: 3 in, 1 out]
        n927 = Increment(x=w2890) -> (x+1=w2889:T15)
        n928 = Search 1D Array(1D array=w2896, element=w2900) -> (index of element=w2899:i32)  [unwired: 1 in]
        n929 = case shown="0, Default" w2899 {
          selector: w2899 -> [w2910 _]
          tunnel: w2898 -> [w2906 w2918]
          tunnel: [w2909 w2918] -> w2897
          tunnel: w2896 -> [w2914 w2917]
          tunnel: [w2913 w2917] -> w2895
          tunnel: w2894 -> [w2912 w2916]
          tunnel: [w2911 w2916] -> w2893
          tunnel: [w2904 w2915] -> w2892
          tunnel: w2891 -> [w2905 w2915]
          frame 0, Default {
            # "Tag found"
            n930 = Delete From Array(array=w2914, index=w2910) -> (array with subset deleted=w2913:string[])  [unwired: 1 in, 1 out]
            n931 = Delete From Array(array=w2912, index=w2910) -> (deleted portion=w2908:T1, array with subset deleted=w2911:T1[])  [unwired: 1 in]
            n932 = call "Decode Single Tag.vi"("Error In"=w2905, "PicoQuant Tag"=w2908) -> ("Error Out"=w2907:errorcluster, "Variant"=w2903:variant)  [unwired: 8 in]
            n933 = Unbundle By Name(w2906) -> ("PQ Image Information.Frame Marker"=w2902:i64)
            n934 = Variant To Data(error in=w2907, type=w2902, Variant=w2903) -> (data=w2901:i64, error out=w2904:errorcluster)
            n935 = Bundle By Name(cluster=w2906, "PQ Image Information.Frame Marker"=w2901) -> (w2909:T2)
          }
          frame -1 {
            # "Tag not found"
          }
        }
      }
      frame "ImgHdr_Ident" {
        n936 = Format Into String(w2920) -> (resulting string=w2930:string)  [unwired: 3 in, 1 out]
        n937 = Increment(x=w2920) -> (x+1=w2919:T15)
        n938 = Search 1D Array(1D array=w2926, element=w2930) -> (index of element=w2929:i32)  [unwired: 1 in]
        n939 = case shown="0, Default" w2929 {
          selector: w2929 -> [w2940 _]
          tunnel: w2928 -> [w2936 w2948]
          tunnel: [w2939 w2948] -> w2927
          tunnel: w2926 -> [w2944 w2947]
          tunnel: [w2943 w2947] -> w2925
          tunnel: w2924 -> [w2942 w2946]
          tunnel: [w2941 w2946] -> w2923
          tunnel: [w2934 w2945] -> w2922
          tunnel: w2921 -> [w2935 w2945]
          frame 0, Default {
            # "Tag found"
            n940 = Delete From Array(array=w2944, index=w2940) -> (array with subset deleted=w2943:string[])  [unwired: 1 in, 1 out]
            n941 = Delete From Array(array=w2942, index=w2940) -> (deleted portion=w2938:T1, array with subset deleted=w2941:T1[])  [unwired: 1 in]
            n942 = call "Decode Single Tag.vi"("Error In"=w2935, "PicoQuant Tag"=w2938) -> ("Error Out"=w2937:errorcluster, "Variant"=w2933:variant)  [unwired: 8 in]
            n943 = Unbundle By Name(w2936) -> ("PQ Image Information.Scanner Identity"=w2932:i64)
            n944 = Variant To Data(error in=w2937, type=w2932, Variant=w2933) -> (data=w2931:i64, error out=w2934:errorcluster)
            n945 = Bundle By Name(cluster=w2936, "PQ Image Information.Scanner Identity"=w2931) -> (w2939:T2)
          }
          frame -1 {
            # "Tag not found"
          }
        }
      }
      frame "ImgHdr_LearningTime" {
        n946 = Format Into String(w2950) -> (resulting string=w2960:string)  [unwired: 3 in, 1 out]
        n947 = Increment(x=w2950) -> (x+1=w2949:T15)
        n948 = Search 1D Array(1D array=w2956, element=w2960) -> (index of element=w2959:i32)  [unwired: 1 in]
        n949 = case shown="0, Default" w2959 {
          selector: w2959 -> [w2970 _]
          tunnel: w2958 -> [w2966 w2978]
          tunnel: [w2969 w2978] -> w2957
          tunnel: w2956 -> [w2974 w2977]
          tunnel: [w2973 w2977] -> w2955
          tunnel: w2954 -> [w2972 w2976]
          tunnel: [w2971 w2976] -> w2953
          tunnel: [w2964 w2975] -> w2952
          tunnel: w2951 -> [w2965 w2975]
          frame 0, Default {
            # "Tag found"
            n950 = Delete From Array(array=w2974, index=w2970) -> (array with subset deleted=w2973:string[])  [unwired: 1 in, 1 out]
            n951 = Delete From Array(array=w2972, index=w2970) -> (deleted portion=w2968:T1, array with subset deleted=w2971:T1[])  [unwired: 1 in]
            n952 = call "Decode Single Tag.vi"("Error In"=w2965, "PicoQuant Tag"=w2968) -> ("Error Out"=w2967:errorcluster, "Variant"=w2963:variant)  [unwired: 8 in]
            n953 = Unbundle By Name(w2966) -> ("PQ Image Information.Learning Time (s)"=w2962:i64)
            n954 = Variant To Data(error in=w2967, type=w2962, Variant=w2963) -> (data=w2961:i64, error out=w2964:errorcluster)
            n955 = Bundle By Name(cluster=w2966, "PQ Image Information.Learning Time (s)"=w2961) -> (w2969:T2)
          }
          frame -1 {
            # "Tag not found"
          }
        }
      }
      frame "ImgHdr_LineFrequency" {
        n956 = Format Into String(w2980) -> (resulting string=w2990:string)  [unwired: 3 in, 1 out]
        n957 = Increment(x=w2980) -> (x+1=w2979:T15)
        n958 = Search 1D Array(1D array=w2986, element=w2990) -> (index of element=w2989:i32)  [unwired: 1 in]
        n959 = case shown="0, Default" w2989 {
          selector: w2989 -> [w3000 _]
          tunnel: w2988 -> [w2996 w3008]
          tunnel: [w2999 w3008] -> w2987
          tunnel: w2986 -> [w3004 w3007]
          tunnel: [w3003 w3007] -> w2985
          tunnel: w2984 -> [w3002 w3006]
          tunnel: [w3001 w3006] -> w2983
          tunnel: [w2994 w3005] -> w2982
          tunnel: w2981 -> [w2995 w3005]
          frame 0, Default {
            # "Tag found"
            n960 = Delete From Array(array=w3004, index=w3000) -> (array with subset deleted=w3003:string[])  [unwired: 1 in, 1 out]
            n961 = Delete From Array(array=w3002, index=w3000) -> (deleted portion=w2998:T1, array with subset deleted=w3001:T1[])  [unwired: 1 in]
            n962 = call "Decode Single Tag.vi"("Error In"=w2995, "PicoQuant Tag"=w2998) -> ("Error Out"=w2997:errorcluster, "Variant"=w2993:variant)  [unwired: 8 in]
            n963 = Unbundle By Name(w2996) -> ("PQ Image Information.Line Frequency"=w2992:dbl)
            n964 = Variant To Data(error in=w2997, type=w2992, Variant=w2993) -> (data=w2991:dbl, error out=w2994:errorcluster)
            n965 = Bundle By Name(cluster=w2996, "PQ Image Information.Line Frequency"=w2991) -> (w2999:T2)
          }
          frame -1 {
            # "Tag not found"
          }
        }
      }
      frame "ImgHdr_LineStart" {
        n966 = Format Into String(w3010) -> (resulting string=w3020:string)  [unwired: 3 in, 1 out]
        n967 = Increment(x=w3010) -> (x+1=w3009:T15)
        n968 = Search 1D Array(1D array=w3016, element=w3020) -> (index of element=w3019:i32)  [unwired: 1 in]
        n969 = case shown="0, Default" w3019 {
          selector: w3019 -> [w3030 _]
          tunnel: w3018 -> [w3026 w3038]
          tunnel: [w3029 w3038] -> w3017
          tunnel: w3016 -> [w3034 w3037]
          tunnel: [w3033 w3037] -> w3015
          tunnel: w3014 -> [w3032 w3036]
          tunnel: [w3031 w3036] -> w3013
          tunnel: [w3024 w3035] -> w3012
          tunnel: w3011 -> [w3025 w3035]
          frame 0, Default {
            # "Tag found"
            n970 = Delete From Array(array=w3034, index=w3030) -> (array with subset deleted=w3033:string[])  [unwired: 1 in, 1 out]
            n971 = Delete From Array(array=w3032, index=w3030) -> (deleted portion=w3028:T1, array with subset deleted=w3031:T1[])  [unwired: 1 in]
            n972 = call "Decode Single Tag.vi"("Error In"=w3025, "PicoQuant Tag"=w3028) -> ("Error Out"=w3027:errorcluster, "Variant"=w3023:variant)  [unwired: 8 in]
            n973 = Unbundle By Name(w3026) -> ("PQ Image Information.Line Start Marker"=w3022:i64)
            n974 = Variant To Data(error in=w3027, type=w3022, Variant=w3023) -> (data=w3021:i64, error out=w3024:errorcluster)
            n975 = Bundle By Name(cluster=w3026, "PQ Image Information.Line Start Marker"=w3021) -> (w3029:T2)
          }
          frame -1 {
            # "Tag not found"
          }
        }
      }
      frame "ImgHdr_LineStop" {
        n976 = Format Into String(w3040) -> (resulting string=w3050:string)  [unwired: 3 in, 1 out]
        n977 = Increment(x=w3040) -> (x+1=w3039:T15)
        n978 = Search 1D Array(1D array=w3046, element=w3050) -> (index of element=w3049:i32)  [unwired: 1 in]
        n979 = case shown="0, Default" w3049 {
          selector: w3049 -> [w3060 _]
          tunnel: w3048 -> [w3056 w3068]
          tunnel: [w3059 w3068] -> w3047
          tunnel: w3046 -> [w3064 w3067]
          tunnel: [w3063 w3067] -> w3045
          tunnel: w3044 -> [w3062 w3066]
          tunnel: [w3061 w3066] -> w3043
          tunnel: [w3054 w3065] -> w3042
          tunnel: w3041 -> [w3055 w3065]
          frame 0, Default {
            # "Tag found"
            n980 = Delete From Array(array=w3064, index=w3060) -> (array with subset deleted=w3063:string[])  [unwired: 1 in, 1 out]
            n981 = Delete From Array(array=w3062, index=w3060) -> (deleted portion=w3058:T1, array with subset deleted=w3061:T1[])  [unwired: 1 in]
            n982 = call "Decode Single Tag.vi"("Error In"=w3055, "PicoQuant Tag"=w3058) -> ("Error Out"=w3057:errorcluster, "Variant"=w3053:variant)  [unwired: 8 in]
            n983 = Unbundle By Name(w3056) -> ("PQ Image Information.Line Stop Marker"=w3052:i64)
            n984 = Variant To Data(error in=w3057, type=w3052, Variant=w3053) -> (data=w3051:i64, error out=w3054:errorcluster)
            n985 = Bundle By Name(cluster=w3056, "PQ Image Information.Line Stop Marker"=w3051) -> (w3059:T2)
          }
          frame -1 {
            # "Tag not found"
          }
        }
      }
      frame "ImgHdr_MaxFrames" {
        n986 = Format Into String(w3070) -> (resulting string=w3080:string)  [unwired: 3 in, 1 out]
        n987 = Increment(x=w3070) -> (x+1=w3069:T15)
        n988 = Search 1D Array(1D array=w3076, element=w3080) -> (index of element=w3079:i32)  [unwired: 1 in]
        n989 = case shown="0, Default" w3079 {
          selector: w3079 -> [w3090 _]
          tunnel: w3078 -> [w3086 w3098]
          tunnel: [w3089 w3098] -> w3077
          tunnel: w3076 -> [w3094 w3097]
          tunnel: [w3093 w3097] -> w3075
          tunnel: w3074 -> [w3092 w3096]
          tunnel: [w3091 w3096] -> w3073
          tunnel: [w3084 w3095] -> w3072
          tunnel: w3071 -> [w3085 w3095]
          frame 0, Default {
            # "Tag found"
            n990 = Delete From Array(array=w3094, index=w3090) -> (array with subset deleted=w3093:string[])  [unwired: 1 in, 1 out]
            n991 = Delete From Array(array=w3092, index=w3090) -> (deleted portion=w3088:T1, array with subset deleted=w3091:T1[])  [unwired: 1 in]
            n992 = call "Decode Single Tag.vi"("Error In"=w3085, "PicoQuant Tag"=w3088) -> ("Error Out"=w3087:errorcluster, "Variant"=w3083:variant)  [unwired: 8 in]
            n993 = Unbundle By Name(w3086) -> ("PQ Image Information.Max Frames"=w3082:i64)
            n994 = Variant To Data(error in=w3087, type=w3082, Variant=w3083) -> (data=w3081:i64, error out=w3084:errorcluster)
            n995 = Bundle By Name(cluster=w3086, "PQ Image Information.Max Frames"=w3081) -> (w3089:T2)
          }
          frame -1 {
            # "Tag not found"
          }
        }
      }
      frame "ImgHdr_ObjectiveName" {
        n996 = Format Into String(w3100) -> (resulting string=w3110:string)  [unwired: 3 in, 1 out]
        n997 = Increment(x=w3100) -> (x+1=w3099:T15)
        n998 = Search 1D Array(1D array=w3106, element=w3110) -> (index of element=w3109:i32)  [unwired: 1 in]
        n999 = case shown="0, Default" w3109 {
          selector: w3109 -> [w3120 _]
          tunnel: w3108 -> [w3116 w3128]
          tunnel: [w3119 w3128] -> w3107
          tunnel: w3106 -> [w3124 w3127]
          tunnel: [w3123 w3127] -> w3105
          tunnel: w3104 -> [w3122 w3126]
          tunnel: [w3121 w3126] -> w3103
          tunnel: [w3114 w3125] -> w3102
          tunnel: w3101 -> [w3115 w3125]
          frame 0, Default {
            # "Tag found"
            n1000 = Delete From Array(array=w3124, index=w3120) -> (array with subset deleted=w3123:string[])  [unwired: 1 in, 1 out]
            n1001 = Delete From Array(array=w3122, index=w3120) -> (deleted portion=w3118:T1, array with subset deleted=w3121:T1[])  [unwired: 1 in]
            n1002 = call "Decode Single Tag.vi"("Error In"=w3115, "PicoQuant Tag"=w3118) -> ("Error Out"=w3117:errorcluster, "Variant"=w3113:variant)  [unwired: 8 in]
            n1003 = Unbundle By Name(w3116) -> ("PQ Image Information.Objective Name"=w3112:string)
            n1004 = Variant To Data(error in=w3117, type=w3112, Variant=w3113) -> (data=w3111:string, error out=w3114:errorcluster)
            n1005 = Bundle By Name(cluster=w3116, "PQ Image Information.Objective Name"=w3111) -> (w3119:T2)
          }
          frame -1 {
            # "Tag not found"
          }
        }
      }
      frame "ImgHdr_PixResol" {
        n1006 = Format Into String(w3130) -> (resulting string=w3140:string)  [unwired: 3 in, 1 out]
        n1007 = Increment(x=w3130) -> (x+1=w3129:T15)
        n1008 = Search 1D Array(1D array=w3136, element=w3140) -> (index of element=w3139:i32)  [unwired: 1 in]
        n1009 = case shown="0, Default" w3139 {
          selector: w3139 -> [w3150 _]
          tunnel: w3138 -> [w3146 w3158]
          tunnel: [w3149 w3158] -> w3137
          tunnel: w3136 -> [w3154 w3157]
          tunnel: [w3153 w3157] -> w3135
          tunnel: w3134 -> [w3152 w3156]
          tunnel: [w3151 w3156] -> w3133
          tunnel: [w3144 w3155] -> w3132
          tunnel: w3131 -> [w3145 w3155]
          frame 0, Default {
            # "Tag found"
            n1010 = Delete From Array(array=w3154, index=w3150) -> (array with subset deleted=w3153:string[])  [unwired: 1 in, 1 out]
            n1011 = Delete From Array(array=w3152, index=w3150) -> (deleted portion=w3148:T1, array with subset deleted=w3151:T1[])  [unwired: 1 in]
            n1012 = call "Decode Single Tag.vi"("Error In"=w3145, "PicoQuant Tag"=w3148) -> ("Error Out"=w3147:errorcluster, "Variant"=w3143:variant)  [unwired: 8 in]
            n1013 = Unbundle By Name(w3146) -> ("PQ Image Information.Pixel Resolution (um)"=w3142:dbl)
            n1014 = Variant To Data(error in=w3147, type=w3142, Variant=w3143) -> (data=w3141:dbl, error out=w3144:errorcluster)
            n1015 = Bundle By Name(cluster=w3146, "PQ Image Information.Pixel Resolution (um)"=w3141) -> (w3149:T2)
          }
          frame -1 {
            # "Tag not found"
          }
        }
      }
      frame "ImgHdr_PixX" {
        n1016 = Format Into String(w3160) -> (resulting string=w3170:string)  [unwired: 3 in, 1 out]
        n1017 = Increment(x=w3160) -> (x+1=w3159:T15)
        n1018 = Search 1D Array(1D array=w3166, element=w3170) -> (index of element=w3169:i32)  [unwired: 1 in]
        n1019 = case shown="0, Default" w3169 {
          selector: w3169 -> [w3180 _]
          tunnel: w3168 -> [w3176 w3188]
          tunnel: [w3179 w3188] -> w3167
          tunnel: w3166 -> [w3184 w3187]
          tunnel: [w3183 w3187] -> w3165
          tunnel: w3164 -> [w3182 w3186]
          tunnel: [w3181 w3186] -> w3163
          tunnel: [w3174 w3185] -> w3162
          tunnel: w3161 -> [w3175 w3185]
          frame 0, Default {
            # "Tag found"
            n1020 = Delete From Array(array=w3184, index=w3180) -> (array with subset deleted=w3183:string[])  [unwired: 1 in, 1 out]
            n1021 = Delete From Array(array=w3182, index=w3180) -> (deleted portion=w3178:T1, array with subset deleted=w3181:T1[])  [unwired: 1 in]
            n1022 = call "Decode Single Tag.vi"("Error In"=w3175, "PicoQuant Tag"=w3178) -> ("Error Out"=w3177:errorcluster, "Variant"=w3173:variant)  [unwired: 8 in]
            n1023 = Unbundle By Name(w3176) -> ("PQ Image Information.# Pixels X"=w3172:i64)
            n1024 = Variant To Data(error in=w3177, type=w3172, Variant=w3173) -> (data=w3171:i64, error out=w3174:errorcluster)
            n1025 = Bundle By Name(cluster=w3176, "PQ Image Information.# Pixels X"=w3171) -> (w3179:T2)
          }
          frame -1 {
            # "Tag not found"
          }
        }
      }
      frame "ImgHdr_PixY" {
        n1026 = Format Into String(w3190) -> (resulting string=w3200:string)  [unwired: 3 in, 1 out]
        n1027 = Increment(x=w3190) -> (x+1=w3189:T15)
        n1028 = Search 1D Array(1D array=w3196, element=w3200) -> (index of element=w3199:i32)  [unwired: 1 in]
        n1029 = case shown="0, Default" w3199 {
          selector: w3199 -> [w3210 _]
          tunnel: w3198 -> [w3206 w3218]
          tunnel: [w3209 w3218] -> w3197
          tunnel: w3196 -> [w3214 w3217]
          tunnel: [w3213 w3217] -> w3195
          tunnel: w3194 -> [w3212 w3216]
          tunnel: [w3211 w3216] -> w3193
          tunnel: [w3204 w3215] -> w3192
          tunnel: w3191 -> [w3205 w3215]
          frame 0, Default {
            # "Tag found"
            n1030 = Delete From Array(array=w3214, index=w3210) -> (array with subset deleted=w3213:string[])  [unwired: 1 in, 1 out]
            n1031 = Delete From Array(array=w3212, index=w3210) -> (deleted portion=w3208:T1, array with subset deleted=w3211:T1[])  [unwired: 1 in]
            n1032 = call "Decode Single Tag.vi"("Error In"=w3205, "PicoQuant Tag"=w3208) -> ("Error Out"=w3207:errorcluster, "Variant"=w3203:variant)  [unwired: 8 in]
            n1033 = Unbundle By Name(w3206) -> ("PQ Image Information.# Pixels Y"=w3202:i64)
            n1034 = Variant To Data(error in=w3207, type=w3202, Variant=w3203) -> (data=w3201:i64, error out=w3204:errorcluster)
            n1035 = Bundle By Name(cluster=w3206, "PQ Image Information.# Pixels Y"=w3201) -> (w3209:T2)
          }
          frame -1 {
            # "Tag not found"
          }
        }
      }
      frame "ImgHdr_PrevPix" {
        n1036 = Format Into String(w3220) -> (resulting string=w3230:string)  [unwired: 3 in, 1 out]
        n1037 = Increment(x=w3220) -> (x+1=w3219:T15)
        n1038 = Search 1D Array(1D array=w3226, element=w3230) -> (index of element=w3229:i32)  [unwired: 1 in]
        n1039 = case shown="0, Default" w3229 {
          selector: w3229 -> [w3240 _]
          tunnel: w3228 -> [w3236 w3248]
          tunnel: [w3239 w3248] -> w3227
          tunnel: w3226 -> [w3244 w3247]
          tunnel: [w3243 w3247] -> w3225
          tunnel: w3224 -> [w3242 w3246]
          tunnel: [w3241 w3246] -> w3223
          tunnel: [w3234 w3245] -> w3222
          tunnel: w3221 -> [w3235 w3245]
          frame 0, Default {
            # "Tag found"
            n1040 = Delete From Array(array=w3244, index=w3240) -> (array with subset deleted=w3243:string[])  [unwired: 1 in, 1 out]
            n1041 = Delete From Array(array=w3242, index=w3240) -> (deleted portion=w3238:T1, array with subset deleted=w3241:T1[])  [unwired: 1 in]
            n1042 = call "Decode Single Tag.vi"("Error In"=w3235, "PicoQuant Tag"=w3238) -> ("Error Out"=w3237:errorcluster, "Variant"=w3233:variant)  [unwired: 8 in]
            n1043 = Unbundle By Name(w3236) -> ("PQ Image Information.Preview Pixels/Line"=w3232:i64)
            n1044 = Variant To Data(error in=w3237, type=w3232, Variant=w3233) -> (data=w3231:i64, error out=w3234:errorcluster)
            n1045 = Bundle By Name(cluster=w3236, "PQ Image Information.Preview Pixels/Line"=w3231) -> (w3239:T2)
          }
          frame -1 {
            # "Tag not found"
          }
        }
      }
      frame "ImgHdr_ScanDirection" {
        n1046 = Format Into String(w3250) -> (resulting string=w3260:string)  [unwired: 3 in, 1 out]
        n1047 = Increment(x=w3250) -> (x+1=w3249:T15)
        n1048 = Search 1D Array(1D array=w3256, element=w3260) -> (index of element=w3259:i32)  [unwired: 1 in]
        n1049 = case shown="0, Default" w3259 {
          selector: w3259 -> [w3270 _]
          tunnel: w3258 -> [w3266 w3278]
          tunnel: [w3269 w3278] -> w3257
          tunnel: w3256 -> [w3274 w3277]
          tunnel: [w3273 w3277] -> w3255
          tunnel: w3254 -> [w3272 w3276]
          tunnel: [w3271 w3276] -> w3253
          tunnel: [w3264 w3275] -> w3252
          tunnel: w3251 -> [w3265 w3275]
          frame 0, Default {
            # "Tag found"
            n1050 = Delete From Array(array=w3274, index=w3270) -> (array with subset deleted=w3273:string[])  [unwired: 1 in, 1 out]
            n1051 = Delete From Array(array=w3272, index=w3270) -> (deleted portion=w3268:T1, array with subset deleted=w3271:T1[])  [unwired: 1 in]
            n1052 = call "Decode Single Tag.vi"("Error In"=w3265, "PicoQuant Tag"=w3268) -> ("Error Out"=w3267:errorcluster, "Variant"=w3263:variant)  [unwired: 8 in]
            n1053 = Unbundle By Name(w3266) -> ("PQ Image Information.Scan Direction"=w3262:i64)
            n1054 = Variant To Data(error in=w3267, type=w3262, Variant=w3263) -> (data=w3261:i64, error out=w3264:errorcluster)
            n1055 = Bundle By Name(cluster=w3266, "PQ Image Information.Scan Direction"=w3261) -> (w3269:T2)
          }
          frame -1 {
            # "Tag not found"
          }
        }
      }
      frame "ImgHdr_SinCorrection" {
        n1056 = Format Into String(w3280) -> (resulting string=w3290:string)  [unwired: 3 in, 1 out]
        n1057 = Increment(x=w3280) -> (x+1=w3279:T15)
        n1058 = Search 1D Array(1D array=w3286, element=w3290) -> (index of element=w3289:i32)  [unwired: 1 in]
        n1059 = case shown="0, Default" w3289 {
          selector: w3289 -> [w3300 _]
          tunnel: w3288 -> [w3296 w3308]
          tunnel: [w3299 w3308] -> w3287
          tunnel: w3286 -> [w3304 w3307]
          tunnel: [w3303 w3307] -> w3285
          tunnel: w3284 -> [w3302 w3306]
          tunnel: [w3301 w3306] -> w3283
          tunnel: [w3294 w3305] -> w3282
          tunnel: w3281 -> [w3295 w3305]
          frame 0, Default {
            # "Tag found"
            n1060 = Delete From Array(array=w3304, index=w3300) -> (array with subset deleted=w3303:string[])  [unwired: 1 in, 1 out]
            n1061 = Delete From Array(array=w3302, index=w3300) -> (deleted portion=w3298:T1, array with subset deleted=w3301:T1[])  [unwired: 1 in]
            n1062 = call "Decode Single Tag.vi"("Error In"=w3295, "PicoQuant Tag"=w3298) -> ("Error Out"=w3297:errorcluster, "Variant"=w3293:variant)  [unwired: 8 in]
            n1063 = Unbundle By Name(w3296) -> ("PQ Image Information.Sinusoidal Correction"=w3292:i64)
            n1064 = Variant To Data(error in=w3297, type=w3292, Variant=w3293) -> (data=w3291:i64, error out=w3294:errorcluster)
            n1065 = Bundle By Name(cluster=w3296, "PQ Image Information.Sinusoidal Correction"=w3291) -> (w3299:T2)
          }
          frame -1 {
            # "Tag not found"
          }
        }
      }
      frame "ImgHdr_TimePerLine" {
        n1066 = Format Into String(w3310) -> (resulting string=w3320:string)  [unwired: 3 in, 1 out]
        n1067 = Increment(x=w3310) -> (x+1=w3309:T15)
        n1068 = Search 1D Array(1D array=w3316, element=w3320) -> (index of element=w3319:i32)  [unwired: 1 in]
        n1069 = case shown="0, Default" w3319 {
          selector: w3319 -> [w3330 _]
          tunnel: w3318 -> [w3326 w3338]
          tunnel: [w3329 w3338] -> w3317
          tunnel: w3316 -> [w3334 w3337]
          tunnel: [w3333 w3337] -> w3315
          tunnel: w3314 -> [w3332 w3336]
          tunnel: [w3331 w3336] -> w3313
          tunnel: [w3324 w3335] -> w3312
          tunnel: w3311 -> [w3325 w3335]
          frame 0, Default {
            # "Tag found"
            n1070 = Delete From Array(array=w3334, index=w3330) -> (array with subset deleted=w3333:string[])  [unwired: 1 in, 1 out]
            n1071 = Delete From Array(array=w3332, index=w3330) -> (deleted portion=w3328:T1, array with subset deleted=w3331:T1[])  [unwired: 1 in]
            n1072 = call "Decode Single Tag.vi"("Error In"=w3325, "PicoQuant Tag"=w3328) -> ("Error Out"=w3327:errorcluster, "Variant"=w3323:variant)  [unwired: 8 in]
            n1073 = Unbundle By Name(w3326) -> ("PQ Image Information.Time per Line (ms)"=w3322:dbl)
            n1074 = Variant To Data(error in=w3327, type=w3322, Variant=w3323) -> (data=w3321:dbl, error out=w3324:errorcluster)
            n1075 = Bundle By Name(cluster=w3326, "PQ Image Information.Time per Line (ms)"=w3321) -> (w3329:T2)
          }
          frame -1 {
            # "Tag not found"
          }
        }
      }
      frame "ImgHdr_TimePerPixel" {
        n1076 = Format Into String(w3340) -> (resulting string=w3350:string)  [unwired: 3 in, 1 out]
        n1077 = Increment(x=w3340) -> (x+1=w3339:T15)
        n1078 = Search 1D Array(1D array=w3346, element=w3350) -> (index of element=w3349:i32)  [unwired: 1 in]
        n1079 = case shown="0, Default" w3349 {
          selector: w3349 -> [w3360 _]
          tunnel: w3348 -> [w3356 w3368]
          tunnel: [w3359 w3368] -> w3347
          tunnel: w3346 -> [w3364 w3367]
          tunnel: [w3363 w3367] -> w3345
          tunnel: w3344 -> [w3362 w3366]
          tunnel: [w3361 w3366] -> w3343
          tunnel: [w3354 w3365] -> w3342
          tunnel: w3341 -> [w3355 w3365]
          frame 0, Default {
            # "Tag found"
            n1080 = Delete From Array(array=w3364, index=w3360) -> (array with subset deleted=w3363:string[])  [unwired: 1 in, 1 out]
            n1081 = Delete From Array(array=w3362, index=w3360) -> (deleted portion=w3358:T1, array with subset deleted=w3361:T1[])  [unwired: 1 in]
            n1082 = call "Decode Single Tag.vi"("Error In"=w3355, "PicoQuant Tag"=w3358) -> ("Error Out"=w3357:errorcluster, "Variant"=w3353:variant)  [unwired: 8 in]
            n1083 = Unbundle By Name(w3356) -> ("PQ Image Information.Time per Pixel (ms)"=w3352:i64)
            n1084 = Variant To Data(error in=w3357, type=w3352, Variant=w3353) -> (data=w3351:i64, error out=w3354:errorcluster)
            n1085 = Bundle By Name(cluster=w3356, "PQ Image Information.Time per Pixel (ms)"=w3351) -> (w3359:T2)
          }
          frame -1 {
            # "Tag not found"
          }
        }
      }
      frame "ImgHdr_TStartFro" {
        n1086 = Increment(x=w3370) -> (x+1=w3369:T15)
      }
      frame "ImgHdr_TStartTo" {
        n1087 = Increment(x=w3376) -> (x+1=w3375:T15)
      }
      frame "ImgHdr_TStopFro" {
        n1088 = Increment(x=w3382) -> (x+1=w3381:T15)
      }
      frame "ImgHdr_TStopTo" {
        n1089 = Increment(x=w3388) -> (x+1=w3387:T15)
      }
      frame "ImgHdr_Velocity" {
        n1090 = Format Into String(w3394) -> (resulting string=w3404:string)  [unwired: 3 in, 1 out]
        n1091 = Increment(x=w3394) -> (x+1=w3393:T15)
        n1092 = Search 1D Array(1D array=w3400, element=w3404) -> (index of element=w3403:i32)  [unwired: 1 in]
        n1093 = case shown="0, Default" w3403 {
          selector: w3403 -> [w3414 _]
          tunnel: w3402 -> [w3410 w3422]
          tunnel: [w3413 w3422] -> w3401
          tunnel: w3400 -> [w3418 w3421]
          tunnel: [w3417 w3421] -> w3399
          tunnel: w3398 -> [w3416 w3420]
          tunnel: [w3415 w3420] -> w3397
          tunnel: [w3408 w3419] -> w3396
          tunnel: w3395 -> [w3409 w3419]
          frame 0, Default {
            # "Tag found"
            n1094 = Delete From Array(array=w3418, index=w3414) -> (array with subset deleted=w3417:string[])  [unwired: 1 in, 1 out]
            n1095 = Delete From Array(array=w3416, index=w3414) -> (deleted portion=w3412:T1, array with subset deleted=w3415:T1[])  [unwired: 1 in]
            n1096 = call "Decode Single Tag.vi"("Error In"=w3409, "PicoQuant Tag"=w3412) -> ("Error Out"=w3411:errorcluster, "Variant"=w3407:variant)  [unwired: 8 in]
            n1097 = Unbundle By Name(w3410) -> ("PQ Image Information.Velocity"=w3406:i64)
            n1098 = Variant To Data(error in=w3411, type=w3406, Variant=w3407) -> (data=w3405:i64, error out=w3408:errorcluster)
            n1099 = Bundle By Name(cluster=w3410, "PQ Image Information.Velocity"=w3405) -> (w3413:T2)
          }
          frame -1 {
            # "Tag not found"
          }
        }
      }
      frame "ImgHdr_X0" {
        n1100 = Format Into String(w3424) -> (resulting string=w3434:string)  [unwired: 3 in, 1 out]
        n1101 = Increment(x=w3424) -> (x+1=w3423:T15)
        n1102 = Search 1D Array(1D array=w3430, element=w3434) -> (index of element=w3433:i32)  [unwired: 1 in]
        n1103 = case shown="0, Default" w3433 {
          selector: w3433 -> [w3444 _]
          tunnel: w3432 -> [w3440 w3452]
          tunnel: [w3443 w3452] -> w3431
          tunnel: w3430 -> [w3448 w3451]
          tunnel: [w3447 w3451] -> w3429
          tunnel: w3428 -> [w3446 w3450]
          tunnel: [w3445 w3450] -> w3427
          tunnel: [w3438 w3449] -> w3426
          tunnel: w3425 -> [w3439 w3449]
          frame 0, Default {
            # "Tag found"
            n1104 = Delete From Array(array=w3448, index=w3444) -> (array with subset deleted=w3447:string[])  [unwired: 1 in, 1 out]
            n1105 = Delete From Array(array=w3446, index=w3444) -> (deleted portion=w3442:T1, array with subset deleted=w3445:T1[])  [unwired: 1 in]
            n1106 = call "Decode Single Tag.vi"("Error In"=w3439, "PicoQuant Tag"=w3442) -> ("Error Out"=w3441:errorcluster, "Variant"=w3437:variant)  [unwired: 8 in]
            n1107 = Unbundle By Name(w3440) -> ("PQ Image Information.X0 (um)"=w3436:dbl)
            n1108 = Variant To Data(error in=w3441, type=w3436, Variant=w3437) -> (data=w3435:dbl, error out=w3438:errorcluster)
            n1109 = Bundle By Name(cluster=w3440, "PQ Image Information.X0 (um)"=w3435) -> (w3443:T2)
          }
          frame -1 {
            # "Tag not found"
          }
        }
      }
      frame "ImgHdr_X1" {
        n1110 = Format Into String(w3454) -> (resulting string=w3464:string)  [unwired: 3 in, 1 out]
        n1111 = Increment(x=w3454) -> (x+1=w3453:T15)
        n1112 = Search 1D Array(1D array=w3460, element=w3464) -> (index of element=w3463:i32)  [unwired: 1 in]
        n1113 = case shown="0, Default" w3463 {
          selector: w3463 -> [w3474 _]
          tunnel: w3462 -> [w3470 w3482]
          tunnel: [w3473 w3482] -> w3461
          tunnel: w3460 -> [w3478 w3481]
          tunnel: [w3477 w3481] -> w3459
          tunnel: w3458 -> [w3476 w3480]
          tunnel: [w3475 w3480] -> w3457
          tunnel: [w3468 w3479] -> w3456
          tunnel: w3455 -> [w3469 w3479]
          frame 0, Default {
            # "Tag found"
            n1114 = Delete From Array(array=w3478, index=w3474) -> (array with subset deleted=w3477:string[])  [unwired: 1 in, 1 out]
            n1115 = Delete From Array(array=w3476, index=w3474) -> (deleted portion=w3472:T1, array with subset deleted=w3475:T1[])  [unwired: 1 in]
            n1116 = call "Decode Single Tag.vi"("Error In"=w3469, "PicoQuant Tag"=w3472) -> ("Error Out"=w3471:errorcluster, "Variant"=w3467:variant)  [unwired: 8 in]
            n1117 = Unbundle By Name(w3470) -> ("PQ Image Information.X1 (um)"=w3466:dbl)
            n1118 = Variant To Data(error in=w3471, type=w3466, Variant=w3467) -> (data=w3465:dbl, error out=w3468:errorcluster)
            n1119 = Bundle By Name(cluster=w3470, "PQ Image Information.X1 (um)"=w3465) -> (w3473:T2)
          }
          frame -1 {
            # "Tag not found"
          }
        }
      }
      frame "ImgHdr_XCalibOffset" {
        n1120 = Format Into String(w3484) -> (resulting string=w3494:string)  [unwired: 3 in, 1 out]
        n1121 = Increment(x=w3484) -> (x+1=w3483:T15)
        n1122 = Search 1D Array(1D array=w3490, element=w3494) -> (index of element=w3493:i32)  [unwired: 1 in]
        n1123 = case shown="0, Default" w3493 {
          selector: w3493 -> [w3504 _]
          tunnel: w3492 -> [w3500 w3512]
          tunnel: [w3503 w3512] -> w3491
          tunnel: w3490 -> [w3508 w3511]
          tunnel: [w3507 w3511] -> w3489
          tunnel: w3488 -> [w3506 w3510]
          tunnel: [w3505 w3510] -> w3487
          tunnel: [w3498 w3509] -> w3486
          tunnel: w3485 -> [w3499 w3509]
          frame 0, Default {
            # "Tag found"
            n1124 = Delete From Array(array=w3508, index=w3504) -> (array with subset deleted=w3507:string[])  [unwired: 1 in, 1 out]
            n1125 = Delete From Array(array=w3506, index=w3504) -> (deleted portion=w3502:T1, array with subset deleted=w3505:T1[])  [unwired: 1 in]
            n1126 = Unbundle By Name(w3500) -> ("PQ Image Information.X Calibration Offset (V)"=w3496:dbl)
            n1127 = call "Decode Single Tag.vi"("Error In"=w3499, "PicoQuant Tag"=w3502) -> ("Error Out"=w3501:errorcluster, "Variant"=w3497:variant)  [unwired: 8 in]
            n1128 = Variant To Data(error in=w3501, type=w3496, Variant=w3497) -> (data=w3495:dbl, error out=w3498:errorcluster)
            n1129 = Bundle By Name(cluster=w3500, "PQ Image Information.X Calibration Offset (V)"=w3495) -> (w3503:T2)
          }
          frame -1 {
            # "Tag not found"
          }
        }
      }
      frame "ImgHdr_XCalibration" {
        n1130 = Format Into String(w3514) -> (resulting string=w3524:string)  [unwired: 3 in, 1 out]
        n1131 = Increment(x=w3514) -> (x+1=w3513:T15)
        n1132 = Search 1D Array(1D array=w3520, element=w3524) -> (index of element=w3523:i32)  [unwired: 1 in]
        n1133 = case shown="0, Default" w3523 {
          selector: w3523 -> [w3534 _]
          tunnel: w3522 -> [w3530 w3542]
          tunnel: [w3533 w3542] -> w3521
          tunnel: w3520 -> [w3538 w3541]
          tunnel: [w3537 w3541] -> w3519
          tunnel: w3518 -> [w3536 w3540]
          tunnel: [w3535 w3540] -> w3517
          tunnel: [w3528 w3539] -> w3516
          tunnel: w3515 -> [w3529 w3539]
          frame 0, Default {
            # "Tag found"
            n1134 = Delete From Array(array=w3538, index=w3534) -> (array with subset deleted=w3537:string[])  [unwired: 1 in, 1 out]
            n1135 = Delete From Array(array=w3536, index=w3534) -> (deleted portion=w3532:T1, array with subset deleted=w3535:T1[])  [unwired: 1 in]
            n1136 = call "Decode Single Tag.vi"("Error In"=w3529, "PicoQuant Tag"=w3532) -> ("Error Out"=w3531:errorcluster, "Variant"=w3527:variant)  [unwired: 8 in]
            n1137 = Unbundle By Name(w3530) -> ("PQ Image Information.X Calibration (m/V)"=w3526:dbl)
            n1138 = Variant To Data(error in=w3531, type=w3526, Variant=w3527) -> (data=w3525:dbl, error out=w3528:errorcluster)
            n1139 = Bundle By Name(cluster=w3530, "PQ Image Information.X Calibration (m/V)"=w3525) -> (w3533:T2)
          }
          frame -1 {
            # "Tag not found"
          }
        }
      }
      frame "ImgHdr_Y0" {
        n1140 = Format Into String(w3544) -> (resulting string=w3554:string)  [unwired: 3 in, 1 out]
        n1141 = Increment(x=w3544) -> (x+1=w3543:T15)
        n1142 = Search 1D Array(1D array=w3550, element=w3554) -> (index of element=w3553:i32)  [unwired: 1 in]
        n1143 = case shown="0, Default" w3553 {
          selector: w3553 -> [w3564 _]
          tunnel: w3552 -> [w3560 w3572]
          tunnel: [w3563 w3572] -> w3551
          tunnel: w3550 -> [w3568 w3571]
          tunnel: [w3567 w3571] -> w3549
          tunnel: w3548 -> [w3566 w3570]
          tunnel: [w3565 w3570] -> w3547
          tunnel: [w3558 w3569] -> w3546
          tunnel: w3545 -> [w3559 w3569]
          frame 0, Default {
            # "Tag found"
            n1144 = Delete From Array(array=w3568, index=w3564) -> (array with subset deleted=w3567:string[])  [unwired: 1 in, 1 out]
            n1145 = Delete From Array(array=w3566, index=w3564) -> (deleted portion=w3562:T1, array with subset deleted=w3565:T1[])  [unwired: 1 in]
            n1146 = call "Decode Single Tag.vi"("Error In"=w3559, "PicoQuant Tag"=w3562) -> ("Error Out"=w3561:errorcluster, "Variant"=w3557:variant)  [unwired: 8 in]
            n1147 = Unbundle By Name(w3560) -> ("PQ Image Information.Y0 (um)"=w3556:dbl)
            n1148 = Variant To Data(error in=w3561, type=w3556, Variant=w3557) -> (data=w3555:dbl, error out=w3558:errorcluster)
            n1149 = Bundle By Name(cluster=w3560, "PQ Image Information.Y0 (um)"=w3555) -> (w3563:T2)
          }
          frame -1 {
            # "Tag not found"
          }
        }
      }
      frame "ImgHdr_Y1" {
        n1150 = Format Into String(w3574) -> (resulting string=w3584:string)  [unwired: 3 in, 1 out]
        n1151 = Increment(x=w3574) -> (x+1=w3573:T15)
        n1152 = Search 1D Array(1D array=w3580, element=w3584) -> (index of element=w3583:i32)  [unwired: 1 in]
        n1153 = case shown="0, Default" w3583 {
          selector: w3583 -> [w3594 _]
          tunnel: w3582 -> [w3590 w3602]
          tunnel: [w3593 w3602] -> w3581
          tunnel: w3580 -> [w3598 w3601]
          tunnel: [w3597 w3601] -> w3579
          tunnel: w3578 -> [w3596 w3600]
          tunnel: [w3595 w3600] -> w3577
          tunnel: [w3588 w3599] -> w3576
          tunnel: w3575 -> [w3589 w3599]
          frame 0, Default {
            # "Tag found"
            n1154 = Delete From Array(array=w3598, index=w3594) -> (array with subset deleted=w3597:string[])  [unwired: 1 in, 1 out]
            n1155 = Delete From Array(array=w3596, index=w3594) -> (deleted portion=w3592:T1, array with subset deleted=w3595:T1[])  [unwired: 1 in]
            n1156 = call "Decode Single Tag.vi"("Error In"=w3589, "PicoQuant Tag"=w3592) -> ("Error Out"=w3591:errorcluster, "Variant"=w3587:variant)  [unwired: 8 in]
            n1157 = Unbundle By Name(w3590) -> ("PQ Image Information.Y1 (um)"=w3586:dbl)
            n1158 = Variant To Data(error in=w3591, type=w3586, Variant=w3587) -> (data=w3585:dbl, error out=w3588:errorcluster)
            n1159 = Bundle By Name(cluster=w3590, "PQ Image Information.Y1 (um)"=w3585) -> (w3593:T2)
          }
          frame -1 {
            # "Tag not found"
          }
        }
      }
      frame "ImgHdr_YCalibOffset" {
        n1160 = Format Into String(w3604) -> (resulting string=w3614:string)  [unwired: 3 in, 1 out]
        n1161 = Increment(x=w3604) -> (x+1=w3603:T15)
        n1162 = Search 1D Array(1D array=w3610, element=w3614) -> (index of element=w3613:i32)  [unwired: 1 in]
        n1163 = case shown="0, Default" w3613 {
          selector: w3613 -> [w3624 _]
          tunnel: w3612 -> [w3620 w3632]
          tunnel: [w3623 w3632] -> w3611
          tunnel: w3610 -> [w3628 w3631]
          tunnel: [w3627 w3631] -> w3609
          tunnel: w3608 -> [w3626 w3630]
          tunnel: [w3625 w3630] -> w3607
          tunnel: [w3618 w3629] -> w3606
          tunnel: w3605 -> [w3619 w3629]
          frame 0, Default {
            # "Tag found"
            n1164 = Delete From Array(array=w3628, index=w3624) -> (array with subset deleted=w3627:string[])  [unwired: 1 in, 1 out]
            n1165 = Delete From Array(array=w3626, index=w3624) -> (deleted portion=w3622:T1, array with subset deleted=w3625:T1[])  [unwired: 1 in]
            n1166 = Unbundle By Name(w3620) -> ("PQ Image Information.Y Calibration Offset (V)"=w3616:dbl)
            n1167 = call "Decode Single Tag.vi"("Error In"=w3619, "PicoQuant Tag"=w3622) -> ("Error Out"=w3621:errorcluster, "Variant"=w3617:variant)  [unwired: 8 in]
            n1168 = Variant To Data(error in=w3621, type=w3616, Variant=w3617) -> (data=w3615:dbl, error out=w3618:errorcluster)
            n1169 = Bundle By Name(cluster=w3620, "PQ Image Information.Y Calibration Offset (V)"=w3615) -> (w3623:T2)
          }
          frame -1 {
            # "Tag not found"
          }
        }
      }
      frame "ImgHdr_YCalibration" {
        n1170 = Format Into String(w3634) -> (resulting string=w3644:string)  [unwired: 3 in, 1 out]
        n1171 = Increment(x=w3634) -> (x+1=w3633:T15)
        n1172 = Search 1D Array(1D array=w3640, element=w3644) -> (index of element=w3643:i32)  [unwired: 1 in]
        n1173 = case shown="0, Default" w3643 {
          selector: w3643 -> [w3654 _]
          tunnel: w3642 -> [w3650 w3662]
          tunnel: [w3653 w3662] -> w3641
          tunnel: w3640 -> [w3658 w3661]
          tunnel: [w3657 w3661] -> w3639
          tunnel: w3638 -> [w3656 w3660]
          tunnel: [w3655 w3660] -> w3637
          tunnel: [w3648 w3659] -> w3636
          tunnel: w3635 -> [w3649 w3659]
          frame 0, Default {
            # "Tag found"
            n1174 = Delete From Array(array=w3658, index=w3654) -> (array with subset deleted=w3657:string[])  [unwired: 1 in, 1 out]
            n1175 = Delete From Array(array=w3656, index=w3654) -> (deleted portion=w3652:T1, array with subset deleted=w3655:T1[])  [unwired: 1 in]
            n1176 = call "Decode Single Tag.vi"("Error In"=w3649, "PicoQuant Tag"=w3652) -> ("Error Out"=w3651:errorcluster, "Variant"=w3647:variant)  [unwired: 8 in]
            n1177 = Unbundle By Name(w3650) -> ("PQ Image Information.Y Calibration (m/V)"=w3646:dbl)
            n1178 = Variant To Data(error in=w3651, type=w3646, Variant=w3647) -> (data=w3645:dbl, error out=w3648:errorcluster)
            n1179 = Bundle By Name(cluster=w3650, "PQ Image Information.Y Calibration (m/V)"=w3645) -> (w3653:T2)
          }
          frame -1 {
            # "Tag not found"
          }
        }
      }
      frame "ImgHdr_Z0" {
        n1180 = Format Into String(w3664) -> (resulting string=w3674:string)  [unwired: 3 in, 1 out]
        n1181 = Increment(x=w3664) -> (x+1=w3663:T15)
        n1182 = Search 1D Array(1D array=w3670, element=w3674) -> (index of element=w3673:i32)  [unwired: 1 in]
        n1183 = case shown="0, Default" w3673 {
          selector: w3673 -> [w3684 _]
          tunnel: w3672 -> [w3680 w3692]
          tunnel: [w3683 w3692] -> w3671
          tunnel: w3670 -> [w3688 w3691]
          tunnel: [w3687 w3691] -> w3669
          tunnel: w3668 -> [w3686 w3690]
          tunnel: [w3685 w3690] -> w3667
          tunnel: [w3678 w3689] -> w3666
          tunnel: w3665 -> [w3679 w3689]
          frame 0, Default {
            # "Tag found"
            n1184 = Delete From Array(array=w3688, index=w3684) -> (array with subset deleted=w3687:string[])  [unwired: 1 in, 1 out]
            n1185 = Delete From Array(array=w3686, index=w3684) -> (deleted portion=w3682:T1, array with subset deleted=w3685:T1[])  [unwired: 1 in]
            n1186 = call "Decode Single Tag.vi"("Error In"=w3679, "PicoQuant Tag"=w3682) -> ("Error Out"=w3681:errorcluster, "Variant"=w3677:variant)  [unwired: 8 in]
            n1187 = Unbundle By Name(w3680) -> ("PQ Image Information.Z0 (um)"=w3676:dbl)
            n1188 = Variant To Data(error in=w3681, type=w3676, Variant=w3677) -> (data=w3675:dbl, error out=w3678:errorcluster)
            n1189 = Bundle By Name(cluster=w3680, "PQ Image Information.Z0 (um)"=w3675) -> (w3683:T2)
          }
          frame -1 {
            # "Tag not found"
          }
        }
      }
      frame "ImgHdr_Z1" {
        n1190 = Format Into String(w3694) -> (resulting string=w3704:string)  [unwired: 3 in, 1 out]
        n1191 = Increment(x=w3694) -> (x+1=w3693:T15)
        n1192 = Search 1D Array(1D array=w3700, element=w3704) -> (index of element=w3703:i32)  [unwired: 1 in]
        n1193 = case shown="0, Default" w3703 {
          selector: w3703 -> [w3714 _]
          tunnel: w3702 -> [w3710 w3722]
          tunnel: [w3713 w3722] -> w3701
          tunnel: w3700 -> [w3718 w3721]
          tunnel: [w3717 w3721] -> w3699
          tunnel: w3698 -> [w3716 w3720]
          tunnel: [w3715 w3720] -> w3697
          tunnel: [w3708 w3719] -> w3696
          tunnel: w3695 -> [w3709 w3719]
          frame 0, Default {
            # "Tag found"
            n1194 = Delete From Array(array=w3718, index=w3714) -> (array with subset deleted=w3717:string[])  [unwired: 1 in, 1 out]
            n1195 = Delete From Array(array=w3716, index=w3714) -> (deleted portion=w3712:T1, array with subset deleted=w3715:T1[])  [unwired: 1 in]
            n1196 = call "Decode Single Tag.vi"("Error In"=w3709, "PicoQuant Tag"=w3712) -> ("Error Out"=w3711:errorcluster, "Variant"=w3707:variant)  [unwired: 8 in]
            n1197 = Unbundle By Name(w3710) -> ("PQ Image Information.Z1 (um)"=w3706:dbl)
            n1198 = Variant To Data(error in=w3711, type=w3706, Variant=w3707) -> (data=w3705:dbl, error out=w3708:errorcluster)
            n1199 = Bundle By Name(cluster=w3710, "PQ Image Information.Z1 (um)"=w3705) -> (w3713:T2)
          }
          frame -1 {
            # "Tag not found"
          }
        }
      }
      frame "ImgHdr_ZCalibOffset" {
        n1200 = Format Into String(w3724) -> (resulting string=w3734:string)  [unwired: 3 in, 1 out]
        n1201 = Increment(x=w3724) -> (x+1=w3723:T15)
        n1202 = Search 1D Array(1D array=w3730, element=w3734) -> (index of element=w3733:i32)  [unwired: 1 in]
        n1203 = case shown="0, Default" w3733 {
          selector: w3733 -> [w3744 _]
          tunnel: w3732 -> [w3740 w3752]
          tunnel: [w3743 w3752] -> w3731
          tunnel: w3730 -> [w3748 w3751]
          tunnel: [w3747 w3751] -> w3729
          tunnel: w3728 -> [w3746 w3750]
          tunnel: [w3745 w3750] -> w3727
          tunnel: [w3738 w3749] -> w3726
          tunnel: w3725 -> [w3739 w3749]
          frame 0, Default {
            # "Tag found"
            n1204 = Delete From Array(array=w3748, index=w3744) -> (array with subset deleted=w3747:string[])  [unwired: 1 in, 1 out]
            n1205 = Delete From Array(array=w3746, index=w3744) -> (deleted portion=w3742:T1, array with subset deleted=w3745:T1[])  [unwired: 1 in]
            n1206 = Unbundle By Name(w3740) -> ("PQ Image Information.Z Calibration Offset (V)"=w3736:dbl)
            n1207 = call "Decode Single Tag.vi"("Error In"=w3739, "PicoQuant Tag"=w3742) -> ("Error Out"=w3741:errorcluster, "Variant"=w3737:variant)  [unwired: 8 in]
            n1208 = Variant To Data(error in=w3741, type=w3736, Variant=w3737) -> (data=w3735:dbl, error out=w3738:errorcluster)
            n1209 = Bundle By Name(cluster=w3740, "PQ Image Information.Z Calibration Offset (V)"=w3735) -> (w3743:T2)
          }
          frame -1 {
            # "Tag not found"
          }
        }
      }
      frame "ImgHdr_ZCalibration" {
        n1210 = Format Into String(w3754) -> (resulting string=w3764:string)  [unwired: 3 in, 1 out]
        n1211 = Increment(x=w3754) -> (x+1=w3753:T15)
        n1212 = Search 1D Array(1D array=w3760, element=w3764) -> (index of element=w3763:i32)  [unwired: 1 in]
        n1213 = case shown="0, Default" w3763 {
          selector: w3763 -> [w3774 _]
          tunnel: w3762 -> [w3770 w3782]
          tunnel: [w3773 w3782] -> w3761
          tunnel: w3760 -> [w3778 w3781]
          tunnel: [w3777 w3781] -> w3759
          tunnel: w3758 -> [w3776 w3780]
          tunnel: [w3775 w3780] -> w3757
          tunnel: [w3768 w3779] -> w3756
          tunnel: w3755 -> [w3769 w3779]
          frame 0, Default {
            # "Tag found"
            n1214 = Delete From Array(array=w3778, index=w3774) -> (array with subset deleted=w3777:string[])  [unwired: 1 in, 1 out]
            n1215 = Delete From Array(array=w3776, index=w3774) -> (deleted portion=w3772:T1, array with subset deleted=w3775:T1[])  [unwired: 1 in]
            n1216 = call "Decode Single Tag.vi"("Error In"=w3769, "PicoQuant Tag"=w3772) -> ("Error Out"=w3771:errorcluster, "Variant"=w3767:variant)  [unwired: 8 in]
            n1217 = Unbundle By Name(w3770) -> ("PQ Image Information.Z  Calibration (m/V)"=w3766:dbl)
            n1218 = Variant To Data(error in=w3771, type=w3766, Variant=w3767) -> (data=w3765:dbl, error out=w3768:errorcluster)
            n1219 = Bundle By Name(cluster=w3770, "PQ Image Information.Z  Calibration (m/V)"=w3765) -> (w3773:T2)
          }
          frame -1 {
            # "Tag not found"
          }
        }
      }
      frame "<TT Measurement Results>" {
        n1220 = Increment(x=w3784) -> (x+1=w3783:T15)
      }
      frame "TTResult_StopReason" {
        n1221 = Format Into String(w3790) -> (resulting string=w3800:string)  [unwired: 3 in, 1 out]
        n1222 = Increment(x=w3790) -> (x+1=w3789:T15)
        n1223 = Search 1D Array(1D array=w3796, element=w3800) -> (index of element=w3799:i32)  [unwired: 1 in]
        n1224 = case shown="0, Default" w3799 {
          selector: w3799 -> [w3810 _]
          tunnel: w3798 -> [w3806 w3818]
          tunnel: [w3809 w3818] -> w3797
          tunnel: w3796 -> [w3814 w3817]
          tunnel: [w3813 w3817] -> w3795
          tunnel: w3794 -> [w3812 w3816]
          tunnel: [w3811 w3816] -> w3793
          tunnel: [w3804 w3815] -> w3792
          tunnel: w3791 -> [w3805 w3815]
          frame 0, Default {
            # "Tag found"
            n1225 = Delete From Array(array=w3814, index=w3810) -> (array with subset deleted=w3813:string[])  [unwired: 1 in, 1 out]
            n1226 = Delete From Array(array=w3812, index=w3810) -> (deleted portion=w3808:T1, array with subset deleted=w3811:T1[])  [unwired: 1 in]
            n1227 = call "Decode Single Tag.vi"("Error In"=w3805, "PicoQuant Tag"=w3808) -> ("Error Out"=w3807:errorcluster, "Variant"=w3803:variant)  [unwired: 8 in]
            n1228 = Unbundle By Name(w3806) -> ("PQ Measurement Results.Stop Reason"=w3802:i64)
            n1229 = Variant To Data(error in=w3807, type=w3802, Variant=w3803) -> (data=w3801:i64, error out=w3804:errorcluster)
            n1230 = Bundle By Name(cluster=w3806, "PQ Measurement Results.Stop Reason"=w3801) -> (w3809:T2)
          }
          frame -1 {
            # "Tag not found"
          }
        }
      }
      frame "TTResult_InputRate" {
        n1231 = Format Into String(w3820) -> (resulting string=w3830:string)  [unwired: 3 in, 1 out]
        n1232 = Search 1D Array(1D array=w3826, element=w3830) -> (index of element=w3829:i32)  [unwired: 1 in]
        n1233 = case shown="-1" w3829 {
          selector: w3829 -> [w3843 _]
          tunnel: w3828 -> [w3839 w3853]
          tunnel: [w3842 w3853] -> w3827
          tunnel: w3826 -> [w3847 w3852]
          tunnel: [w3846 w3852] -> w3825
          tunnel: w3824 -> [w3845 w3851]
          tunnel: [w3844 w3851] -> w3823
          tunnel: [w3837 w3850] -> w3822
          tunnel: w3821 -> [w3838 w3850]
          tunnel: w3820 -> [w3831 w3849]
          tunnel: [w3831 w3848] -> w3819
          frame 0, Default {
            # "Tag found"
            n1234 = Delete From Array(array=w3847, index=w3843) -> (array with subset deleted=w3846:string[])  [unwired: 1 in, 1 out]
            n1235 = Delete From Array(array=w3845, index=w3843) -> (deleted portion=w3841:T1, array with subset deleted=w3844:T1[])  [unwired: 1 in]
            n1236 = call "Decode Single Tag.vi"("Error In"=w3838, "PicoQuant Tag"=w3841) -> ("Error Out"=w3840:errorcluster, "Variant"=w3836:variant)  [unwired: 8 in]
            n1237 = Unbundle By Name(w3839) -> ("PQ Measurement Results.Input Rates (cps)"=w3833:i64[])
            n1238 = Variant To Data(error in=w3840, type=i64 0 ("PQ Measurement Results.Input Rates (cps)"), Variant=w3836) -> (data=w3835:i64, error out=w3837:errorcluster)
            n1239 = Build Array (concatenate)(w3833, w3835) -> (w3834:i64[])
            n1240 = Bundle By Name(cluster=w3839, "PQ Measurement Results.Input Rates (cps)"=w3834) -> (w3842:T2)
          }
          frame -1 {
            # "Tag not found"
            n1241 = Increment(x=w3849) -> (x+1=w3848:T15)
          }
        }
      }
      frame "TTResult_MDescWarningFlags" {
        n1242 = Format Into String(w3855) -> (resulting string=w3865:string)  [unwired: 3 in, 1 out]
        n1243 = Increment(x=w3855) -> (x+1=w3854:T15)
        n1244 = Search 1D Array(1D array=w3861, element=w3865) -> (index of element=w3864:i32)  [unwired: 1 in]
        n1245 = case shown="0, Default" w3864 {
          selector: w3864 -> [w3875 _]
          tunnel: w3863 -> [w3871 w3883]
          tunnel: [w3874 w3883] -> w3862
          tunnel: w3861 -> [w3879 w3882]
          tunnel: [w3878 w3882] -> w3860
          tunnel: w3859 -> [w3877 w3881]
          tunnel: [w3876 w3881] -> w3858
          tunnel: [w3869 w3880] -> w3857
          tunnel: w3856 -> [w3870 w3880]
          frame 0, Default {
            # "Tag found"
            n1246 = Delete From Array(array=w3879, index=w3875) -> (array with subset deleted=w3878:string[])  [unwired: 1 in, 1 out]
            n1247 = Delete From Array(array=w3877, index=w3875) -> (deleted portion=w3873:T1, array with subset deleted=w3876:T1[])  [unwired: 1 in]
            n1248 = call "Decode Single Tag.vi"("Error In"=w3870, "PicoQuant Tag"=w3873) -> ("Error Out"=w3872:errorcluster, "Variant"=w3868:variant)  [unwired: 8 in]
            n1249 = Unbundle By Name(w3871) -> ("PQ Measurement Results.Warning Flags"=w3866:u64)
            n1250 = Variant To Data(error in=w3872, type=w3866, Variant=w3868) -> (data=w3867:u64, error out=w3869:errorcluster)
            n1251 = Bundle By Name(cluster=w3871, "PQ Measurement Results.Warning Flags"=w3867) -> (w3874:T2)
          }
          frame -1 {
            # "Tag not found"
          }
        }
      }
      frame "TTResult_NumberOfRecords" {
        n1252 = Format Into String(w3885) -> (resulting string=w3895:string)  [unwired: 3 in, 1 out]
        n1253 = Increment(x=w3885) -> (x+1=w3884:T15)
        n1254 = Search 1D Array(1D array=w3891, element=w3895) -> (index of element=w3894:i32)  [unwired: 1 in]
        n1255 = case shown="0, Default" w3894 {
          selector: w3894 -> [w3905 _]
          tunnel: w3893 -> [w3901 w3913]
          tunnel: [w3904 w3913] -> w3892
          tunnel: w3891 -> [w3909 w3912]
          tunnel: [w3908 w3912] -> w3890
          tunnel: w3889 -> [w3907 w3911]
          tunnel: [w3906 w3911] -> w3888
          tunnel: [w3899 w3910] -> w3887
          tunnel: w3886 -> [w3900 w3910]
          frame 0, Default {
            # "Tag found"
            n1256 = Delete From Array(array=w3909, index=w3905) -> (array with subset deleted=w3908:string[])  [unwired: 1 in, 1 out]
            n1257 = Delete From Array(array=w3907, index=w3905) -> (deleted portion=w3903:T1, array with subset deleted=w3906:T1[])  [unwired: 1 in]
            n1258 = call "Decode Single Tag.vi"("Error In"=w3900, "PicoQuant Tag"=w3903) -> ("Error Out"=w3902:errorcluster, "Variant"=w3898:variant)  [unwired: 8 in]
            n1259 = Unbundle By Name(w3901) -> ("PQ Measurement Results.# Records"=w3896:i64)
            n1260 = Variant To Data(error in=w3902, type=w3896, Variant=w3898) -> (data=w3897:i64, error out=w3899:errorcluster)
            n1261 = Bundle By Name(cluster=w3901, "PQ Measurement Results.# Records"=w3897) -> (w3904:T2)
          }
          frame -1 {
            # "Tag not found"
          }
        }
      }
      frame "TTResult_StopAfter" {
        n1262 = Format Into String(w3915) -> (resulting string=w3925:string)  [unwired: 3 in, 1 out]
        n1263 = Increment(x=w3915) -> (x+1=w3914:T15)
        n1264 = Search 1D Array(1D array=w3921, element=w3925) -> (index of element=w3924:i32)  [unwired: 1 in]
        n1265 = case shown="0, Default" w3924 {
          selector: w3924 -> [w3935 _]
          tunnel: w3923 -> [w3931 w3943]
          tunnel: [w3934 w3943] -> w3922
          tunnel: w3921 -> [w3939 w3942]
          tunnel: [w3938 w3942] -> w3920
          tunnel: w3919 -> [w3937 w3941]
          tunnel: [w3936 w3941] -> w3918
          tunnel: [w3929 w3940] -> w3917
          tunnel: w3916 -> [w3930 w3940]
          frame 0, Default {
            # "Tag found"
            n1266 = Delete From Array(array=w3939, index=w3935) -> (array with subset deleted=w3938:string[])  [unwired: 1 in, 1 out]
            n1267 = Delete From Array(array=w3937, index=w3935) -> (deleted portion=w3933:T1, array with subset deleted=w3936:T1[])  [unwired: 1 in]
            n1268 = call "Decode Single Tag.vi"("Error In"=w3930, "PicoQuant Tag"=w3933) -> ("Error Out"=w3932:errorcluster, "Variant"=w3928:variant)  [unwired: 8 in]
            n1269 = Unbundle By Name(w3931) -> ("PQ Measurement Results.Stop After (ms)"=w3926:i64)
            n1270 = Variant To Data(error in=w3932, type=w3926, Variant=w3928) -> (data=w3927:i64, error out=w3929:errorcluster)
            n1271 = Bundle By Name(cluster=w3931, "PQ Measurement Results.Stop After (ms)"=w3927) -> (w3934:T2)
          }
          frame -1 {
            # "Tag not found"
          }
        }
      }
      frame "TTResult_SyncRate" {
        n1272 = Format Into String(w3945) -> (resulting string=w3955:string)  [unwired: 3 in, 1 out]
        n1273 = Increment(x=w3945) -> (x+1=w3944:T15)
        n1274 = Search 1D Array(1D array=w3951, element=w3955) -> (index of element=w3954:i32)  [unwired: 1 in]
        n1275 = case shown="0, Default" w3954 {
          selector: w3954 -> [w3965 _]
          tunnel: w3953 -> [w3961 w3973]
          tunnel: [w3964 w3973] -> w3952
          tunnel: w3951 -> [w3969 w3972]
          tunnel: [w3968 w3972] -> w3950
          tunnel: w3949 -> [w3967 w3971]
          tunnel: [w3966 w3971] -> w3948
          tunnel: [w3959 w3970] -> w3947
          tunnel: w3946 -> [w3960 w3970]
          frame 0, Default {
            # "Tag found"
            n1276 = Delete From Array(array=w3969, index=w3965) -> (array with subset deleted=w3968:string[])  [unwired: 1 in, 1 out]
            n1277 = Delete From Array(array=w3967, index=w3965) -> (deleted portion=w3963:T1, array with subset deleted=w3966:T1[])  [unwired: 1 in]
            n1278 = call "Decode Single Tag.vi"("Error In"=w3960, "PicoQuant Tag"=w3963) -> ("Error Out"=w3962:errorcluster, "Variant"=w3958:variant)  [unwired: 8 in]
            n1279 = Unbundle By Name(w3961) -> ("PQ Measurement Results.Sync Rate (cps)"=w3956:i64)
            n1280 = Variant To Data(error in=w3962, type=w3956, Variant=w3958) -> (data=w3957:i64, error out=w3959:errorcluster)
            n1281 = Bundle By Name(cluster=w3961, "PQ Measurement Results.Sync Rate (cps)"=w3957) -> (w3964:T2)
          }
          frame -1 {
            # "Tag not found"
          }
        }
      }
      frame "<TT Results Format>" {
        n1282 = Increment(x=w3975) -> (x+1=w3974:T15)
      }
      frame "TTResultFormat_BitsPerRecord" {
        n1283 = Format Into String(w3981) -> (resulting string=w3991:string)  [unwired: 3 in, 1 out]
        n1284 = Increment(x=w3981) -> (x+1=w3980:T15)
        n1285 = Search 1D Array(1D array=w3987, element=w3991) -> (index of element=w3990:i32)  [unwired: 1 in]
        n1286 = case shown="0, Default" w3990 {
          selector: w3990 -> [w4001 _]
          tunnel: w3989 -> [w3997 w4009]
          tunnel: [w4000 w4009] -> w3988
          tunnel: w3987 -> [w4005 w4008]
          tunnel: [w4004 w4008] -> w3986
          tunnel: w3985 -> [w4003 w4007]
          tunnel: [w4002 w4007] -> w3984
          tunnel: [w3995 w4006] -> w3983
          tunnel: w3982 -> [w3996 w4006]
          frame 0, Default {
            # "Tag found"
            n1287 = Delete From Array(array=w4005, index=w4001) -> (array with subset deleted=w4004:string[])  [unwired: 1 in, 1 out]
            n1288 = Delete From Array(array=w4003, index=w4001) -> (deleted portion=w3999:T1, array with subset deleted=w4002:T1[])  [unwired: 1 in]
            n1289 = call "Decode Single Tag.vi"("Error In"=w3996, "PicoQuant Tag"=w3999) -> ("Error Out"=w3998:errorcluster, "Variant"=w3994:variant)  [unwired: 8 in]
            n1290 = Unbundle By Name(w3997) -> ("PQ TT Results Format Information.Bits per Record"=w3992:i64)
            n1291 = Variant To Data(error in=w3998, type=w3992, Variant=w3994) -> (data=w3993:i64, error out=w3995:errorcluster)
            n1292 = Bundle By Name(cluster=w3997, "PQ TT Results Format Information.Bits per Record"=w3993) -> (w4000:T2)
          }
          frame -1 {
            # "Tag not found"
          }
        }
      }
      frame "TTResultFormat_ChannelMask" {
        n1293 = Format Into String(w4011) -> (resulting string=w4021:string)  [unwired: 3 in, 1 out]
        n1294 = Increment(x=w4011) -> (x+1=w4010:T15)
        n1295 = Search 1D Array(1D array=w4017, element=w4021) -> (index of element=w4020:i32)  [unwired: 1 in]
        n1296 = case shown="0, Default" w4020 {
          selector: w4020 -> [w4031 _]
          tunnel: w4019 -> [w4027 w4039]
          tunnel: [w4030 w4039] -> w4018
          tunnel: w4017 -> [w4035 w4038]
          tunnel: [w4034 w4038] -> w4016
          tunnel: w4015 -> [w4033 w4037]
          tunnel: [w4032 w4037] -> w4014
          tunnel: [w4025 w4036] -> w4013
          tunnel: w4012 -> [w4026 w4036]
          frame 0, Default {
            # "Tag found"
            n1297 = Delete From Array(array=w4035, index=w4031) -> (array with subset deleted=w4034:string[])  [unwired: 1 in, 1 out]
            n1298 = Delete From Array(array=w4033, index=w4031) -> (deleted portion=w4029:T1, array with subset deleted=w4032:T1[])  [unwired: 1 in]
            n1299 = call "Decode Single Tag.vi"("Error In"=w4026, "PicoQuant Tag"=w4029) -> ("Error Out"=w4028:errorcluster, "Variant"=w4024:variant)  [unwired: 8 in]
            n1300 = Unbundle By Name(w4027) -> ("PQ TT Results Format Information.Channel Mask"=w4022:i64)
            n1301 = Variant To Data(error in=w4028, type=w4022, Variant=w4024) -> (data=w4023:i64, error out=w4025:errorcluster)
            n1302 = Bundle By Name(cluster=w4027, "PQ TT Results Format Information.Channel Mask"=w4023) -> (w4030:T2)
          }
          frame -1 {
            # "Tag not found"
          }
        }
      }
      frame "TTResultFormat_ChannelShift" {
        n1303 = Format Into String(w4041) -> (resulting string=w4051:string)  [unwired: 3 in, 1 out]
        n1304 = Increment(x=w4041) -> (x+1=w4040:T15)
        n1305 = Search 1D Array(1D array=w4047, element=w4051) -> (index of element=w4050:i32)  [unwired: 1 in]
        n1306 = case shown="0, Default" w4050 {
          selector: w4050 -> [w4061 _]
          tunnel: w4049 -> [w4057 w4069]
          tunnel: [w4060 w4069] -> w4048
          tunnel: w4047 -> [w4065 w4068]
          tunnel: [w4064 w4068] -> w4046
          tunnel: w4045 -> [w4063 w4067]
          tunnel: [w4062 w4067] -> w4044
          tunnel: [w4055 w4066] -> w4043
          tunnel: w4042 -> [w4056 w4066]
          frame 0, Default {
            # "Tag found"
            n1307 = Delete From Array(array=w4065, index=w4061) -> (array with subset deleted=w4064:string[])  [unwired: 1 in, 1 out]
            n1308 = Delete From Array(array=w4063, index=w4061) -> (deleted portion=w4059:T1, array with subset deleted=w4062:T1[])  [unwired: 1 in]
            n1309 = call "Decode Single Tag.vi"("Error In"=w4056, "PicoQuant Tag"=w4059) -> ("Error Out"=w4058:errorcluster, "Variant"=w4054:variant)  [unwired: 8 in]
            n1310 = Unbundle By Name(w4057) -> ("PQ TT Results Format Information.Channel Shift"=w4052:i64)
            n1311 = Variant To Data(error in=w4058, type=w4052, Variant=w4054) -> (data=w4053:i64, error out=w4055:errorcluster)
            n1312 = Bundle By Name(cluster=w4057, "PQ TT Results Format Information.Channel Shift"=w4053) -> (w4060:T2)
          }
          frame -1 {
            # "Tag not found"
          }
        }
      }
      frame "TTResultFormat_DTimeMask" {
        n1313 = Format Into String(w4071) -> (resulting string=w4081:string)  [unwired: 3 in, 1 out]
        n1314 = Increment(x=w4071) -> (x+1=w4070:T15)
        n1315 = Search 1D Array(1D array=w4077, element=w4081) -> (index of element=w4080:i32)  [unwired: 1 in]
        n1316 = case shown="0, Default" w4080 {
          selector: w4080 -> [w4091 _]
          tunnel: w4079 -> [w4087 w4099]
          tunnel: [w4090 w4099] -> w4078
          tunnel: w4077 -> [w4095 w4098]
          tunnel: [w4094 w4098] -> w4076
          tunnel: w4075 -> [w4093 w4097]
          tunnel: [w4092 w4097] -> w4074
          tunnel: [w4085 w4096] -> w4073
          tunnel: w4072 -> [w4086 w4096]
          frame 0, Default {
            # "Tag found"
            n1317 = Delete From Array(array=w4095, index=w4091) -> (array with subset deleted=w4094:string[])  [unwired: 1 in, 1 out]
            n1318 = Delete From Array(array=w4093, index=w4091) -> (deleted portion=w4089:T1, array with subset deleted=w4092:T1[])  [unwired: 1 in]
            n1319 = call "Decode Single Tag.vi"("Error In"=w4086, "PicoQuant Tag"=w4089) -> ("Error Out"=w4088:errorcluster, "Variant"=w4084:variant)  [unwired: 8 in]
            n1320 = Unbundle By Name(w4087) -> ("PQ TT Results Format Information.DTime Mask"=w4082:i64)
            n1321 = Variant To Data(error in=w4088, type=w4082, Variant=w4084) -> (data=w4083:i64, error out=w4085:errorcluster)
            n1322 = Bundle By Name(cluster=w4087, "PQ TT Results Format Information.DTime Mask"=w4083) -> (w4090:T2)
          }
          frame -1 {
            # "Tag not found"
          }
        }
      }
      frame "TTResultFormat_DTimeShift" {
        n1323 = Format Into String(w4101) -> (resulting string=w4111:string)  [unwired: 3 in, 1 out]
        n1324 = Increment(x=w4101) -> (x+1=w4100:T15)
        n1325 = Search 1D Array(1D array=w4107, element=w4111) -> (index of element=w4110:i32)  [unwired: 1 in]
        n1326 = case shown="0, Default" w4110 {
          selector: w4110 -> [w4121 _]
          tunnel: w4109 -> [w4117 w4129]
          tunnel: [w4120 w4129] -> w4108
          tunnel: w4107 -> [w4125 w4128]
          tunnel: [w4124 w4128] -> w4106
          tunnel: w4105 -> [w4123 w4127]
          tunnel: [w4122 w4127] -> w4104
          tunnel: [w4115 w4126] -> w4103
          tunnel: w4102 -> [w4116 w4126]
          frame 0, Default {
            # "Tag found"
            n1327 = Delete From Array(array=w4125, index=w4121) -> (array with subset deleted=w4124:string[])  [unwired: 1 in, 1 out]
            n1328 = Delete From Array(array=w4123, index=w4121) -> (deleted portion=w4119:T1, array with subset deleted=w4122:T1[])  [unwired: 1 in]
            n1329 = call "Decode Single Tag.vi"("Error In"=w4116, "PicoQuant Tag"=w4119) -> ("Error Out"=w4118:errorcluster, "Variant"=w4114:variant)  [unwired: 8 in]
            n1330 = Unbundle By Name(w4117) -> ("PQ TT Results Format Information.DTime Shift"=w4112:i64)
            n1331 = Variant To Data(error in=w4118, type=w4112, Variant=w4114) -> (data=w4113:i64, error out=w4115:errorcluster)
            n1332 = Bundle By Name(cluster=w4117, "PQ TT Results Format Information.DTime Shift"=w4113) -> (w4120:T2)
          }
          frame -1 {
            # "Tag not found"
          }
        }
      }
      frame "TTResultFormat_MarkerMask" {
        n1333 = Format Into String(w4131) -> (resulting string=w4141:string)  [unwired: 3 in, 1 out]
        n1334 = Increment(x=w4131) -> (x+1=w4130:T15)
        n1335 = Search 1D Array(1D array=w4137, element=w4141) -> (index of element=w4140:i32)  [unwired: 1 in]
        n1336 = case shown="0, Default" w4140 {
          selector: w4140 -> [w4151 _]
          tunnel: w4139 -> [w4147 w4159]
          tunnel: [w4150 w4159] -> w4138
          tunnel: w4137 -> [w4155 w4158]
          tunnel: [w4154 w4158] -> w4136
          tunnel: w4135 -> [w4153 w4157]
          tunnel: [w4152 w4157] -> w4134
          tunnel: [w4145 w4156] -> w4133
          tunnel: w4132 -> [w4146 w4156]
          frame 0, Default {
            # "Tag found"
            n1337 = Delete From Array(array=w4155, index=w4151) -> (array with subset deleted=w4154:string[])  [unwired: 1 in, 1 out]
            n1338 = Delete From Array(array=w4153, index=w4151) -> (deleted portion=w4149:T1, array with subset deleted=w4152:T1[])  [unwired: 1 in]
            n1339 = call "Decode Single Tag.vi"("Error In"=w4146, "PicoQuant Tag"=w4149) -> ("Error Out"=w4148:errorcluster, "Variant"=w4144:variant)  [unwired: 8 in]
            n1340 = Unbundle By Name(w4147) -> ("PQ TT Results Format Information.Marker Mask"=w4142:i64)
            n1341 = Variant To Data(error in=w4148, type=w4142, Variant=w4144) -> (data=w4143:i64, error out=w4145:errorcluster)
            n1342 = Bundle By Name(cluster=w4147, "PQ TT Results Format Information.Marker Mask"=w4143) -> (w4150:T2)
          }
          frame -1 {
            # "Tag not found"
          }
        }
      }
      frame "TTResultFormat_MarkerShift" {
        n1343 = Format Into String(w4161) -> (resulting string=w4171:string)  [unwired: 3 in, 1 out]
        n1344 = Increment(x=w4161) -> (x+1=w4160:T15)
        n1345 = Search 1D Array(1D array=w4167, element=w4171) -> (index of element=w4170:i32)  [unwired: 1 in]
        n1346 = case shown="0, Default" w4170 {
          selector: w4170 -> [w4181 _]
          tunnel: w4169 -> [w4177 w4189]
          tunnel: [w4180 w4189] -> w4168
          tunnel: w4167 -> [w4185 w4188]
          tunnel: [w4184 w4188] -> w4166
          tunnel: w4165 -> [w4183 w4187]
          tunnel: [w4182 w4187] -> w4164
          tunnel: [w4175 w4186] -> w4163
          tunnel: w4162 -> [w4176 w4186]
          frame 0, Default {
            # "Tag found"
            n1347 = Delete From Array(array=w4185, index=w4181) -> (array with subset deleted=w4184:string[])  [unwired: 1 in, 1 out]
            n1348 = Delete From Array(array=w4183, index=w4181) -> (deleted portion=w4179:T1, array with subset deleted=w4182:T1[])  [unwired: 1 in]
            n1349 = call "Decode Single Tag.vi"("Error In"=w4176, "PicoQuant Tag"=w4179) -> ("Error Out"=w4178:errorcluster, "Variant"=w4174:variant)  [unwired: 8 in]
            n1350 = Unbundle By Name(w4177) -> ("PQ TT Results Format Information.Marker Shift"=w4172:i64)
            n1351 = Variant To Data(error in=w4178, type=w4172, Variant=w4174) -> (data=w4173:i64, error out=w4175:errorcluster)
            n1352 = Bundle By Name(cluster=w4177, "PQ TT Results Format Information.Marker Shift"=w4173) -> (w4180:T2)
          }
          frame -1 {
            # "Tag not found"
          }
        }
      }
      frame "TTResultFormat_NSyncMask" {
        n1353 = Format Into String(w4191) -> (resulting string=w4201:string)  [unwired: 3 in, 1 out]
        n1354 = Increment(x=w4191) -> (x+1=w4190:T15)
        n1355 = Search 1D Array(1D array=w4197, element=w4201) -> (index of element=w4200:i32)  [unwired: 1 in]
        n1356 = case shown="0, Default" w4200 {
          selector: w4200 -> [w4211 _]
          tunnel: w4199 -> [w4207 w4219]
          tunnel: [w4210 w4219] -> w4198
          tunnel: w4197 -> [w4215 w4218]
          tunnel: [w4214 w4218] -> w4196
          tunnel: w4195 -> [w4213 w4217]
          tunnel: [w4212 w4217] -> w4194
          tunnel: [w4205 w4216] -> w4193
          tunnel: w4192 -> [w4206 w4216]
          frame 0, Default {
            # "Tag found"
            n1357 = Delete From Array(array=w4215, index=w4211) -> (array with subset deleted=w4214:string[])  [unwired: 1 in, 1 out]
            n1358 = Delete From Array(array=w4213, index=w4211) -> (deleted portion=w4209:T1, array with subset deleted=w4212:T1[])  [unwired: 1 in]
            n1359 = call "Decode Single Tag.vi"("Error In"=w4206, "PicoQuant Tag"=w4209) -> ("Error Out"=w4208:errorcluster, "Variant"=w4204:variant)  [unwired: 8 in]
            n1360 = Unbundle By Name(w4207) -> ("PQ TT Results Format Information.NSync Mask"=w4202:i64)
            n1361 = Variant To Data(error in=w4208, type=w4202, Variant=w4204) -> (data=w4203:i64, error out=w4205:errorcluster)
            n1362 = Bundle By Name(cluster=w4207, "PQ TT Results Format Information.NSync Mask"=w4203) -> (w4210:T2)
          }
          frame -1 {
            # "Tag not found"
          }
        }
      }
      frame "TTResultFormat_NSyncShift" {
        n1363 = Format Into String(w4221) -> (resulting string=w4231:string)  [unwired: 3 in, 1 out]
        n1364 = Increment(x=w4221) -> (x+1=w4220:T15)
        n1365 = Search 1D Array(1D array=w4227, element=w4231) -> (index of element=w4230:i32)  [unwired: 1 in]
        n1366 = case shown="0, Default" w4230 {
          selector: w4230 -> [w4241 _]
          tunnel: w4229 -> [w4237 w4249]
          tunnel: [w4240 w4249] -> w4228
          tunnel: w4227 -> [w4245 w4248]
          tunnel: [w4244 w4248] -> w4226
          tunnel: w4225 -> [w4243 w4247]
          tunnel: [w4242 w4247] -> w4224
          tunnel: [w4235 w4246] -> w4223
          tunnel: w4222 -> [w4236 w4246]
          frame 0, Default {
            # "Tag found"
            n1367 = Delete From Array(array=w4245, index=w4241) -> (array with subset deleted=w4244:string[])  [unwired: 1 in, 1 out]
            n1368 = Delete From Array(array=w4243, index=w4241) -> (deleted portion=w4239:T1, array with subset deleted=w4242:T1[])  [unwired: 1 in]
            n1369 = call "Decode Single Tag.vi"("Error In"=w4236, "PicoQuant Tag"=w4239) -> ("Error Out"=w4238:errorcluster, "Variant"=w4234:variant)  [unwired: 8 in]
            n1370 = Unbundle By Name(w4237) -> ("PQ TT Results Format Information.NSync Shift"=w4232:i64)
            n1371 = Variant To Data(error in=w4238, type=w4232, Variant=w4234) -> (data=w4233:i64, error out=w4235:errorcluster)
            n1372 = Bundle By Name(cluster=w4237, "PQ TT Results Format Information.NSync Shift"=w4233) -> (w4240:T2)
          }
          frame -1 {
            # "Tag not found"
          }
        }
      }
      frame "TTResultFormat_SpecialMask" {
        n1373 = Format Into String(w4251) -> (resulting string=w4261:string)  [unwired: 3 in, 1 out]
        n1374 = Increment(x=w4251) -> (x+1=w4250:T15)
        n1375 = Search 1D Array(1D array=w4257, element=w4261) -> (index of element=w4260:i32)  [unwired: 1 in]
        n1376 = case shown="0, Default" w4260 {
          selector: w4260 -> [w4271 _]
          tunnel: w4259 -> [w4267 w4279]
          tunnel: [w4270 w4279] -> w4258
          tunnel: w4257 -> [w4275 w4278]
          tunnel: [w4274 w4278] -> w4256
          tunnel: w4255 -> [w4273 w4277]
          tunnel: [w4272 w4277] -> w4254
          tunnel: [w4265 w4276] -> w4253
          tunnel: w4252 -> [w4266 w4276]
          frame 0, Default {
            # "Tag found"
            n1377 = Delete From Array(array=w4275, index=w4271) -> (array with subset deleted=w4274:string[])  [unwired: 1 in, 1 out]
            n1378 = Delete From Array(array=w4273, index=w4271) -> (deleted portion=w4269:T1, array with subset deleted=w4272:T1[])  [unwired: 1 in]
            n1379 = call "Decode Single Tag.vi"("Error In"=w4266, "PicoQuant Tag"=w4269) -> ("Error Out"=w4268:errorcluster, "Variant"=w4264:variant)  [unwired: 8 in]
            n1380 = Unbundle By Name(w4267) -> ("PQ TT Results Format Information.Special Mask"=w4262:i64)
            n1381 = Variant To Data(error in=w4268, type=w4262, Variant=w4264) -> (data=w4263:i64, error out=w4265:errorcluster)
            n1382 = Bundle By Name(cluster=w4267, "PQ TT Results Format Information.Special Mask"=w4263) -> (w4270:T2)
          }
          frame -1 {
            # "Tag not found"
          }
        }
      }
      frame "TTResultFormat_TTTRRecType" {
        n1383 = Format Into String(w4281) -> (resulting string=w4291:string)  [unwired: 3 in, 1 out]
        n1384 = Increment(x=w4281) -> (x+1=w4280:T15)
        n1385 = Search 1D Array(1D array=w4287, element=w4291) -> (index of element=w4290:i32)  [unwired: 1 in]
        n1386 = case shown="0, Default" w4290 {
          selector: w4290 -> [w4301 _]
          tunnel: w4289 -> [w4297 w4309]
          tunnel: [w4300 w4309] -> w4288
          tunnel: w4287 -> [w4305 w4308]
          tunnel: [w4304 w4308] -> w4286
          tunnel: w4285 -> [w4303 w4307]
          tunnel: [w4302 w4307] -> w4284
          tunnel: [w4295 w4306] -> w4283
          tunnel: w4282 -> [w4296 w4306]
          frame 0, Default {
            # "Tag found"
            n1387 = Delete From Array(array=w4305, index=w4301) -> (array with subset deleted=w4304:string[])  [unwired: 1 in, 1 out]
            n1388 = Delete From Array(array=w4303, index=w4301) -> (deleted portion=w4299:T1, array with subset deleted=w4302:T1[])  [unwired: 1 in]
            n1389 = call "Decode Single Tag.vi"("Error In"=w4296, "PicoQuant Tag"=w4299) -> ("Error Out"=w4298:errorcluster, "Variant"=w4294:variant)  [unwired: 8 in]
            n1390 = Unbundle By Name(w4297) -> ("PQ TT Results Format Information.TTTR Record Type"=w4292:i64)
            n1391 = Variant To Data(error in=w4298, type=w4292, Variant=w4294) -> (data=w4293:i64, error out=w4295:errorcluster)
            n1392 = Bundle By Name(cluster=w4297, "PQ TT Results Format Information.TTTR Record Type"=w4293) -> (w4300:T2)
          }
          frame -1 {
            # "Tag not found"
          }
        }
      }
      frame "TTResultFormat_WrapAround" {
        n1393 = Format Into String(w4311) -> (resulting string=w4321:string)  [unwired: 3 in, 1 out]
        n1394 = Increment(x=w4311) -> (x+1=w4310:T15)
        n1395 = Search 1D Array(1D array=w4317, element=w4321) -> (index of element=w4320:i32)  [unwired: 1 in]
        n1396 = case shown="0, Default" w4320 {
          selector: w4320 -> [w4331 _]
          tunnel: w4319 -> [w4327 w4339]
          tunnel: [w4330 w4339] -> w4318
          tunnel: w4317 -> [w4335 w4338]
          tunnel: [w4334 w4338] -> w4316
          tunnel: w4315 -> [w4333 w4337]
          tunnel: [w4332 w4337] -> w4314
          tunnel: [w4325 w4336] -> w4313
          tunnel: w4312 -> [w4326 w4336]
          frame 0, Default {
            # "Tag found"
            n1397 = Delete From Array(array=w4335, index=w4331) -> (array with subset deleted=w4334:string[])  [unwired: 1 in, 1 out]
            n1398 = Delete From Array(array=w4333, index=w4331) -> (deleted portion=w4329:T1, array with subset deleted=w4332:T1[])  [unwired: 1 in]
            n1399 = call "Decode Single Tag.vi"("Error In"=w4326, "PicoQuant Tag"=w4329) -> ("Error Out"=w4328:errorcluster, "Variant"=w4324:variant)  [unwired: 8 in]
            n1400 = Unbundle By Name(w4327) -> ("PQ TT Results Format Information.Wrap Around"=w4322:i64)
            n1401 = Variant To Data(error in=w4328, type=w4322, Variant=w4324) -> (data=w4323:i64, error out=w4325:errorcluster)
            n1402 = Bundle By Name(cluster=w4327, "PQ TT Results Format Information.Wrap Around"=w4323) -> (w4330:T2)
          }
          frame -1 {
            # "Tag not found"
          }
        }
      }
      frame "Header_End" {
      }
    }
    n1403 = Format Into String(w13) -> (resulting string=w12:string)  [unwired: 3 in, 1 out]
    n1404 = Unbundle By Name(w15) -> ("status"=w14:bool)
  }
  "PicoQuant Data File Information" <- w6
  "Tags with Error" <- w1
  n1405 = Merge Errors(w3) -> (→"error out":errorcluster)
